vi "myRIO_BRig_RT_v0,78__PortC.vi"() -> ()   [LabVIEW 2014]
uses:
  myRIO_BRig_RT__Case_Exp_stateList.ctl
  myRIO_BRig_RT__Case_NonExp_stateList.ctl
  <vilib>/Platform/TimedLoop/XDataNode/timing_clust.ctl
  <vilib>/Platform/TimedLoop/XDataNode/nitl_modes.ctl
  <vilib>/Platform/TimedLoop/XDataNode/wakeup.ctl
  <vilib>/WebDAVClient/Advanced/SessionHandle.ctl
  <vilib>/myRIO/Common/Instrument Driver Framework/myRIO v1.0/UART/vis/myRIO v1.0 Close UART.vi
  <vilib>/FPGAPlugInAG/myRIO-1900/niLvFpga_Open_myRIO-1900.vi
  <vilib>/rvi/interface/common/dynamic/niFpgaDynamicAddResources.vi
  <vilib>/Utility/error.llb/Error Cluster From Error Code.vi
  <vilib>/rvi/errors/niLvFpgaAdjustHostInterfaceError.vi
  <vilib>/FPGAPlugInAG/Dynamic/niLvFpga_Close_Dynamic.vi
  <vilib>/myRIO/Common/Instrument Driver Framework/Utilities/vis/FPGA Ref Manager.vi
  <vilib>/myRIO/Common/Instrument Driver Framework/myRIO v1.0/myRIO v1.0 Reset FPGA.vi
  <vilib>/myRIO/Common/Instrument Driver Framework/myRIO v1.0/IRQ/vis/myRIO v1.0 IRQ Info FGV.vi
  <vilib>/myRIO/Common/Instrument Driver Framework/myRIO v1.0/IRQ/vis/myRIO v1.0 Timer IRQ Info FGV.vi
  <vilib>/myRIO/Common/Instrument Driver Framework/myRIO v1.0/IRQ/vis/myRIO v1.0 ISR Agent.vi
  <vilib>/rvi/interface/nirviOpenFPGA/nirviOpenFPGA.xnode
  FPGA Bitfiles/myRIOBRig_FPGATarget_myRIOBRigFPGAv3,_Jim92IOu6W4.lvbitx
  myRIO_BRig_FPGA_v3,70__PortC.vi
  <vilib>/rvi/interface/nirviReadWriteControl/nirviReadWriteControl.xnode
  <vilib>/Platform/TimedLoop/XDataNode/XDataNode.xnode
  <vilib>/rvi/interface/nirviCloseFPGA/nirviCloseFPGA.xnode
  <vilib>/Platform/TimedLoop/XDataNode/XDNodeRunTimeDep.lvlib
  <vilib>/rvi/interface/Simulation/niFpgaSimulationCallBeginRW.vi
  <vilib>/myRIO/Instrument Drivers/Utilities/Utilities.lvlib
  <vilib>/WebDAVClient/NI_WebDAV.lvlib
  NiFpgaLv.dll
panel:
  out "error out 6":errorcluster
  in  "MTrig_Laser_Switch":bool
  in  "Cue1Param_AudioLed_Count_NS":u16
  in  "Cue1Param_AudioLed_Count_Switch":u16
  in  "Cue1Param_AudioLed_Probability_NS":u16
  in  "Cue1Param_CueType_NS":u16(slide) max=2 step=1 scale=0.0..2.0
  in  "Cue1Param_AudioLed_Probability_Switch":u16
  in  "Cue1Param_CueType_Switch":u16(slide) max=2 step=1 scale=0.0..2.0
  in  "CueLed_Freq":dbl=10.0
  in  "CueLed_Tpeak":dbl=2.0
  in  "CueLed_duration":u16
  in  "Laser_power_step_l2":dbl
  in  "Laser_power_max_l2":dbl
  in  "Laser_power_min_l2":dbl
  in  "Laser_Tshutter_l2":dbl=2.0
  in  "Laser_Freq_l2":dbl=10.0
  in  "Laser_Tpeak_l2":dbl=2.0
  in  "Laser_duration_l2":u16
  in  "LC_Sel_Count_NS_l2":u16
  in  "LC_Sel_Count_Switch_l2":u16
  in  "LC_Sel_Probability_NS_l2":u16
  in  "LC_Sel_Block_NS_l2":u16(slide) max=2 step=1 scale=0.0..2.0
  in  "LC_Sel_OnOff_NS_l2":bool
  in  "LC_Sel_Probability_Switch_l2":u16
  in  "LC_Sel_Block_Switch_l2":u16(slide) max=2 step=1 scale=0.0..2.0
  in  "LC_Sel_OnOff_Switch_l2":bool
  in  "LC_Sel_Tdelay_NS_l2":u16
  in  "LC_Sel_Tdelay_Switch_l2":u16
  in  "LC_Cue1_Count_NS_l2":u16
  in  "LC_Cue1_Count_Switch_l2":u16
  in  "LC_Cue1_delayOpt_NS_l2":bool
  in  "LC_ENL1_delayOpt_NS_l2":bool
  in  "LC_ENL1_Count_NS_l2":u16
  in  "LC_ENL1_Count_Switch_l2":u16
  in  "LC_Cue1_delayOpt_Switch_l2":bool
  in  "LC_ENL1_delayOpt_Switch_l2":bool
  in  "LC_Cue1_Probability_NS_l2":u16
  in  "LC_Cue1_Block_NS_l2":u16(slide) max=2 step=1 scale=0.0..2.0
  in  "LC_Cue1_OnOff_NS_l2":bool
  in  "LC_Cue1_Probability_Switch_l2":u16
  in  "LC_Cue1_Block_Switch_l2":u16(slide) max=2 step=1 scale=0.0..2.0
  in  "LC_Cue1_OnOff_Switch_l2":bool
  in  "LC_ENL1_Probability_NS_l2":u16 max=100 step=1
  in  "LC_ENL1_Block_NS_l2":u16(slide) max=2 step=1 scale=0.0..2.0
  in  "LC_ENL1_OnOff_NS_l2":bool
  in  "LC_ENL1_Probability_Switch_l2":u16 max=100 step=1
  in  "LC_ENL1_Block_Switch_l2":u16(slide) max=2 step=1 scale=0.0..2.0
  in  "LC_Cue1_Tdelay_NS_l2":u16
  in  "LC_ENL1_Tdelay_NS_l2":u16
  in  "LC_Cue1_Tdelay_Switch_l2":u16
  in  "LC_ENL1_Tdelay_Switch_l2":u16
  in  "LC_ENL1_OnOff_Switch_l2":bool
  in  "LC_Wrong_Probability_l2":u16
  in  "LC_Wrong_Trial_l2":u16(slide) max=2 step=1 scale=0.0..2.0
  in  "LC_Wrong_Block_l2":u16(slide) max=2 step=1 scale=0.0..2.0
  in  "LC_Wrong_OnOff_l2":bool
  in  "LC_Reward_Probability_l2":u16
  in  "LC_Reward_Trial_l2":u16(slide) max=2 step=1 scale=0.0..2.0
  in  "LC_Reward_Block_l2":u16(slide) max=2 step=1 scale=0.0..2.0
  in  "LC_Reward_OnOff_l2":bool
  in  "LC_Wrong_Tdelay_l2":u16
  in  "LC_Reward_Tdelay_l2":u16
  in  "LC_Sel_Count_NS_l1":u16
  in  "LC_Sel_Count_Switch_l1":u16
  in  "LC_Sel_Probability_NS_l1":u16
  in  "LC_Sel_Block_NS_l1":u16(slide) max=2 step=1 scale=0.0..2.0
  in  "LC_Sel_OnOff_NS_l1":bool
  in  "LC_Sel_Probability_Switch_l1":u16
  in  "LC_Sel_Block_Switch_l1":u16(slide) max=2 step=1 scale=0.0..2.0
  in  "LC_Sel_OnOff_Switch_l1":bool
  in  "LC_Sel_Tdelay_NS_l1":u16
  in  "LC_Sel_Tdelay_Switch_l1":u16
  out "I_connect_TCP":bool
  out "error out 5":errorcluster
  in  "get_countPerMS":bool
  in  "count_warmup_R_reset":bool
  in  "count_warmup_L_reset":bool
  out "count_warmup_R":u16
  out "count_warmup_L":u16
  out "SolenoidReward":bool
  in  "SolenoidProbability_L":u16=50 caption="Reward Time [ms]" min=1 max=1000 step=1
  in  "SolenoidProbability_R":u16=50 caption="Reward Time [ms]" min=1 max=1000 step=1
  out "output_PortA":dbl caption="LaserPower"
  out "error out 4":errorcluster
  in  "Laser_power_step_l1":dbl
  in  "Laser_power_max_l1":dbl
  in  "Recording":bool
  out "error out 3":errorcluster
  out "error out 2":errorcluster
  in  "Laser_power_min_l1":dbl
  in  "FPGA_count2ms":dbl=159.0
  in  "Laser_Tshutter_l1":dbl=2.0
  in  "Laser_Freq_l1":dbl=10.0
  in  "Laser_Tpeak_l1":dbl=2.0
  in  "Laser_duration_l1":u16
  out "error out":errorcluster
  in  "LC_Cue1_Count_NS_l1":u16
  in  "LC_Cue1_Count_Switch_l1":u16
  in  "LC_Cue1_delayOpt_NS_l1":bool
  in  "LC_ENL1_delayOpt_NS_l1":bool
  in  "LC_ENL1_Count_NS_l1":u16
  in  "LC_ENL1_Count_Switch_l1":u16
  in  "LC_Cue1_delayOpt_Switch_l1":bool
  in  "LC_ENL1_delayOpt_Switch_l1":bool
  in  "Tcycle_Cue_max":u16=1000 caption="Max" min=5 max=5000 step=5
  in  "Tcycle_Cue_min":u16=1000 caption="Min" min=5 max=5000 step=5
  in  "SendData":bool
  out "cSpout":enum16{"Left", "Right"}(ring) caption="Left or Right Spout"
  out "A4":u32 caption="LickCounter_Right"
  out "A2":u32 caption="LickCounter_Left"
  in  "LR_wrong_Event":bool
  out "error_initTrial":errorcluster
  out "error_Selection_pre":errorcluster
  out "error_Selection":errorcluster
  out "SelectWrong":bool
  out "SelectReward":bool
  in  "Left(F)_or_Right(T)":bool
  in  "ignoreWrong":bool
  in  "SelectionState":bool
  in  "LR_wrong_Laser":bool
  in  "LR_reward_Laser":bool
  in  "LR_reward_Event":bool
  out "nRewards_Right":u16 caption="# Rewards Total (Right)"
  out "nRewards_Left":u16 caption="# Rewards Total (Left)"
  out "nRewards_cur":u16 caption="# Rewards in Current Block"
  out "TpB_target":u16 caption="Target Trials Per Block"
  out "cState_NonExp":T1 caption="WarmUp State"
  out "iBlock":u16 caption="Current Block"
  out "cState":T2 caption="Experimental State"
  out "iTrial":u16 caption="Current Trial"
  in  "warmupType":u8(slide) max=2 step=1 scale=0.0..2.0
  in  "TestConnection":bool
  in  "warmup":bool caption="WarmUp"
  in  "Data Set Prefix":string="Exp1_TM2"
  out "Connected To Host?":bool
  in  "Host Password":string="sabalab"
  in  "Host UserName":string="Test2"
  in  "sp_RightSpout":u16(slide)=2 max=2 step=1 scale=0.0..2.0
  in  "sp_LeftSpout":u16(slide)=2 max=2 step=1 scale=0.0..2.0
  in  "BUR_max":u16 caption="Count Reward Structure  (0 = off)"
  in  "LC_Wrong_Probability_l1":u16
  in  "LC_Wrong_Trial_l1":u16(slide) max=2 step=1 scale=0.0..2.0
  in  "LC_Wrong_Block_l1":u16(slide) max=2 step=1 scale=0.0..2.0
  in  "LC_Wrong_OnOff_l1":bool
  in  "LC_Reward_Probability_l1":u16
  in  "LC_Reward_Trial_l1":u16(slide) max=2 step=1 scale=0.0..2.0
  in  "LC_Reward_Block_l1":u16(slide) max=2 step=1 scale=0.0..2.0
  in  "LC_Reward_OnOff_l1":bool
  in  "LC_Cue1_Probability_NS_l1":u16
  in  "LC_Cue1_Block_NS_l1":u16(slide) max=2 step=1 scale=0.0..2.0
  in  "LC_Cue1_OnOff_NS_l1":bool
  in  "LC_Cue1_Probability_Switch_l1":u16
  in  "LC_Cue1_Block_Switch_l1":u16(slide) max=2 step=1 scale=0.0..2.0
  in  "LC_Cue1_OnOff_Switch_l1":bool
  in  "LC_ENL1_Probability_NS_l1":u16 max=100 step=1
  in  "LC_ENL1_Block_NS_l1":u16(slide) max=2 step=1 scale=0.0..2.0
  in  "LC_ENL1_OnOff_NS_l1":bool
  in  "LC_ENL1_Probability_Switch_l1":u16 max=100 step=1
  in  "LC_ENL1_Block_Switch_l1":u16(slide) max=2 step=1 scale=0.0..2.0
  in  "Tcycle_Timeout":u16=1000 caption="Timeout Time [ms]" min=10 max=10000 step=1
  in  "Tcycle_Wrong":u16=1000 caption="Wrong Time [ms]" min=10 max=10000 step=1
  in  "Tcycle_Selection":u16=1000 caption="Answer Time [ms]" min=1 max=10000 step=1
  in  "Tcycle_RewardPost":u16=1000 caption="Consumption Time [ms]" min=250 max=10000 step=250
  in  "Tcycle_Reward_L":u16=500 caption="Reward Time [ms]" min=1 max=1000 step=1
  in  "Tcycle_Reward_R":u16=500 caption="Reward Time [ms]" min=1 max=1000 step=1
  in  "TpB_Max_R":u16=4 caption="Max TrialsPerBlock" min=1 max=12 step=1
  in  "TpB_Min_R":u16=4 caption="Min TrialsPerBlock" min=1 max=12 step=1
  in  "TpB_Max_L":u16=4 caption="Max TrialsPerBlock" min=1 max=12 step=1
  in  "TpB_Min_L":u16=4 caption="Min TrialsPerBlock" min=1 max=12 step=1
  in  "BUR_min":u16 caption="Count Reward Structure\n(0 = off)"
  in  "TrialUntilReward":bool caption="Ignore Wrong Selection"
  in  "CueCycles":u16=1 caption="Cue Structure" min=1 max=1 step=1
  in  "MTrig_Laser_Tcycle":u16=10 caption="Time [ms]"
  in  "MTrig_Laser_trig":bool
  in  "MTrig_Audio_trig__R":bool caption="Trigger Audio"
  in  "MTrig_Audio_trig__L":bool caption="Trigger Audio"
  in  "RewCalib_Trig_R":bool caption="Calibrate_R"
  in  "RewCalib_Trig_L":bool caption="Calibrate_L"
  in  "MTrig_Solenoid_Tcycle__R":u16=300 caption="Time [ms]"
  in  "MTrig_Solenoid_Tcycle__L":u16=300 caption="Time [ms]"
  in  "MTrig_Solenoid_trig__R":bool caption="Solenoid"
  in  "MTrig_Solenoid_trig__L":bool caption="Solenoid"
  in  "STOP_abort":bool caption="Stop LabView\n(Stops myRio and FPGA)"
  in  "STOP_endBlock":bool caption="Stop Experiment\n@ End of Block"
  in  "STOP_endTrial":bool caption="Stop Experiment\n@ End of Trial"
  in  "START":bool caption="Start Experiment"
  in  "Tcycle_CuePenalty":u16=1000 caption="Penalty" min=1 max=10000 step=1
  in  "Audio_Amp__R":u16=100 caption="Amp"
  in  "Audio_Freq__R":u8=5 caption="Freq [kHz]" max=14 step=1
  in  "Audio_Amp__L":u16=100 caption="Amp"
  in  "Audio_Freq__L":u8=5 caption="Freq [kHz]" max=14 step=1
  in  "LC_Wrong_Tdelay_l1":u16
  in  "LC_Cue1_Tdelay_NS_l1":u16
  in  "LC_ENL1_Tdelay_NS_l1":u16
  in  "LC_Reward_Tdelay_l1":u16
  in  "LC_Cue1_Tdelay_Switch_l1":u16
  in  "LC_ENL1_Tdelay_Switch_l1":u16
  in  "LC_ENL1_OnOff_Switch_l1":bool
  in  "Tcycle_ENLPenalty":u16=100 caption="Penalty" min=10 max=10000 step=10
  in  "Tcycle_ENL_max":u16=1000 caption="Max" min=250 max=10000 step=250
  in  "Tcycle_ENL_min":u16=1000 caption="Min" min=250 max=10000 step=250
  # "Communication (Host PC)"
  # "Recording Rig"
  # "Experimental Run"
  # "Current State"
  # "STOP experiment at"
  # "Global Parameters                                                         Trial Parameters"
  # "Left/Right        Give Reward?        Laser Power [V]"
  # "FPGA Count per [ms]"
  # "Experiment Task Structure"
  # "Timing [ms]"
  # "Block                   Trial            Target Trials       # Rewards \n                                                            Per Block             Current"
  # "Min            Max            Penalty"
  # "(1) = Switching\n(2) = Two Choice"
  # "WarmUp State"
  # "Lick Counter"
  # "Enforced\nNonLick"
  # "WarmUp"
  # "Left           Right"
  # "Cue then reward (no lick)\n \nLeft                    Right"
  # "# Rewards Total\n                                                                  Left                    Right"
  # "Cue"
  # "Experimental State"
  # "Selection\n \n\n \nReward\n    Dispense\n    Time\n \n    Dispense\n    Probability\n \n\n    Consumption\n    Time\n\nWrong Choice\n \n \nTimeout Penalty"
  # "Laser1 Control\n                               On/Off      Block        Probability [%]   Delay [ms]                              Count"
  # "Left                  Right"
  # "Manual Control"
  # "Enforced\nNonLick\n      1"
  # "Min"
  # "Max"
  # "from end"
  # "Solenoid\n \nLeft              Right"
  # "Switch\nTrial"
  # "Speaker\n \nLeft                    Right"
  # "Laser 1  |  Laser 2"
  # "from start"
  # "Trial Per Block Structure \n               Left                        Right"
  # "from end"
  # "NonSwitch\nTrials"
  # "from start"
  # "Time\n[ms]"
  # "Time\n[ms]"
  # "Time = Cue Min"
  # "Min"
  # "Cue 1"
  # "Power = Min"
  # "from end"
  # "Switch\nTrial"
  # "Max"
  # "from start"
  # "Cue Audio Parameters"
  # "Laser1 Parameters"
  # "Left                  Right"
  # "from end"
  # "Laser1 Response\n                               On/Off      Block       Trial       Probability [%]   Delay [ms]"
  # "Frequency\n[Hz]"
  # "NonSwitch\nTrials"
  # "Frequency\n[kHz]"
  # "from start"
  # "Timing [ms]\n Duration     Peak Width   Shutter"
  # "Selection Reward"
  # "Selection"
  # "Amp\n(0 - 32,000)"
  # "from start"
  # "Switch\nTrial"
  # "Laser Power [V]\nMin          Max              Step"
  # "Speaker\nPattern\nDuring Cue"
  # "Selection Wrong"
  # "from start"
  # "NonSwitch\nTrials"
  # "Cue LED Parameters"
  # "Laser2 Parameters"
  # "Laser2 Response\n                               On/Off      Block       Trial       Probability [%]   Delay [ms]"
  # "Laser2 Control\n                               On/Off      Block        Probability [%]   Delay [ms]                              Count"
  # "Frequency\n[Hz]"
  # "Frequency\n[Hz]"
  # "Selection Reward"
  # "Enforced\nNonLick\n      1"
  # "from end"
  # "Timing [ms]\n Duration     Peak Width"
  # "Timing [ms]\n Duration     Peak Width   Shutter"
  # "Switch\nTrial"
  # "from start"
  # "Selection Wrong"
  # "from end"
  # "Laser Power [V]\nMin          Max              Step"
  # "NonSwitch\nTrials"
  # "from start"
  # "Cue 1"
  # "from end"
  # "Switch\nTrial"
  # "from start"
  # "Cue1 Control\n                                         Cue Type                     Audio or LED       LED Probability [%]      Count"
  # "from end"
  # "NonSwitch\nTrials"
  # "Cue 1"
  # "from start"
  # "Switch\nTrial"
  # "Selection"
  # "from start"
  # "Switch\nTrial"
  # "NonSwitch\nTrials"
  # "from start"
  # "NonSwitch\nTrials"
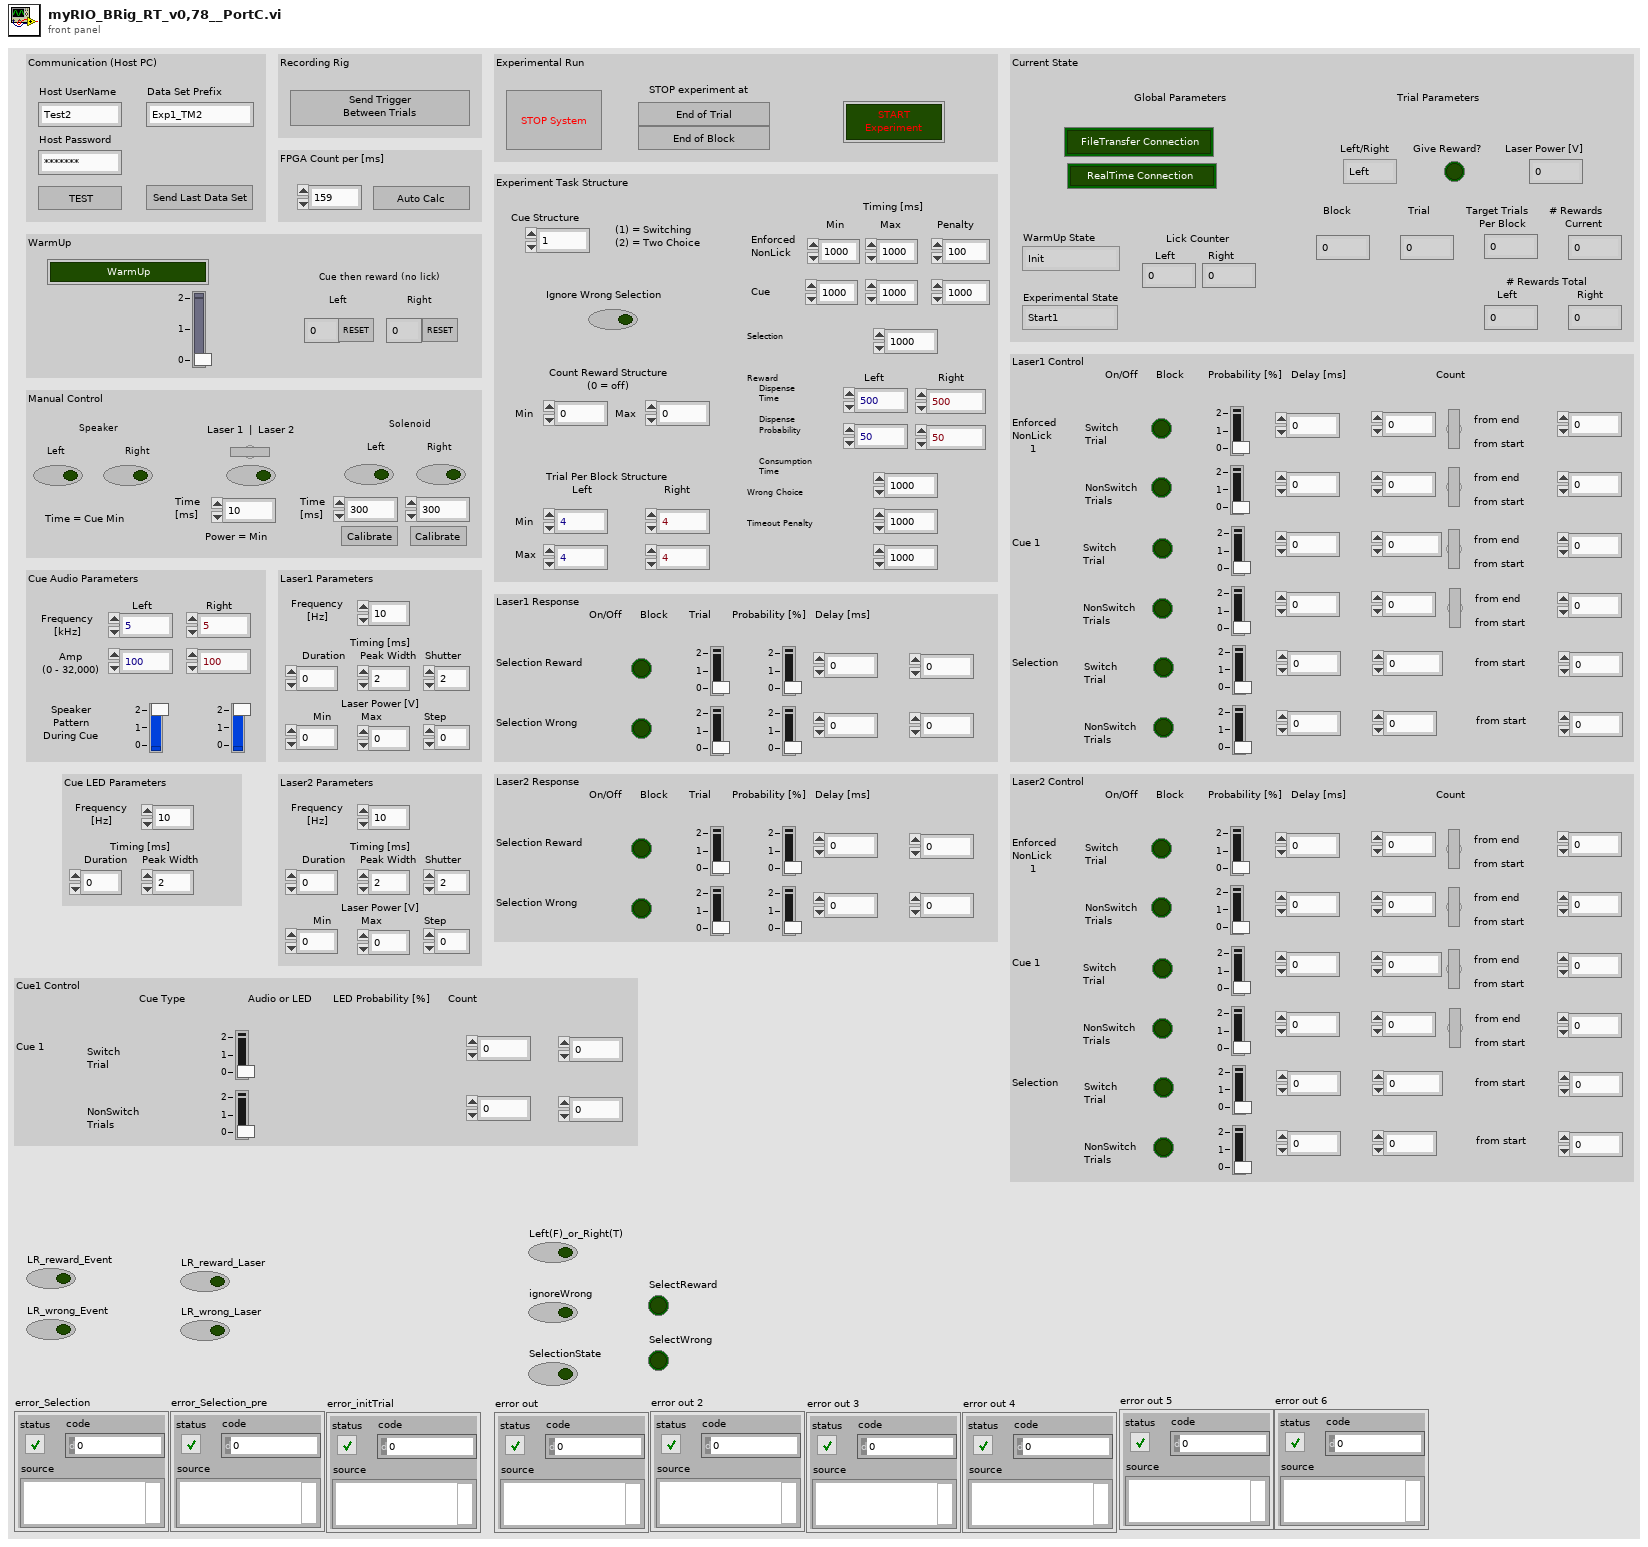
[diagram p1: front panel]
types:
  T1 = typedef "myRIO_BRig_RT__Case_NonExp_stateList.ctl" = enum16{"Init", "UploadSettings_pre", "UploadSettings_Read_dataExp", "UploadSettings_dataExp_1", "UploadSettings_dataExp_2", "UploadSettings_Read_dataLC", "UploadSettings_dataLC_1", "UploadSettings_dataLC_2", "UploadSettings_dataLC_3", "UploadSettings_dataLC_4", "UploadSettings_Read_dataMTrig", "UploadSettings_dataMTrig_1", "UploadSettings_post", "Idle_pre", "IdleEmpty", "IdleEmpty2", "IdleEmpty3", "IdleEmpty4", "Idle", "Idle_2", "Idle_3", "Idle_4", "Idle_5", "Idle_6", "Idle_post", "Cue_pre__pre", "Cue_pre", "Cue", "Cue_LED", "Cue_post", "RewardCalibration_pre", "DispenseWater_pre__pre", "DispenseWater_pre", "DispenseWater", "DispenseWater_post", "TestConnection", "SendData", "Get_FPGA_count_per_ms", "End"}
  T2 = typedef "myRIO_BRig_RT__Case_Exp_stateList.ctl" = enum16{"Start1", "Start2", "Start3", "saveSettings1", "saveSettings2", "saveSettings3", "saveSettings4", "saveSettings_LC_ENL_l1", "saveSettings_LC_ENL_l2", "saveSettings_LC_Cue_l1", "saveSettings_LC_Cue_l2", "saveSettings6_LC_l1_Other", "SaveSettings6_LC_l2_Other", "setSettings_Audio", "setSettings_Laser", "initBlock_pre", "initBlock", "initBlock2", "initBlock_post", "initTrial_pre", "initTrial", "initTrial2", "initTrial3", "initTrial4", "initTrial_LC_ENL1", "initTrial_LC_Cue1", "initTrial_LC_Cue1_2", "initTrial_LC_Sel", "initTrial_post", "ENL1_pre", "ENL1", "ENL1_post", "ENL1Penalty_pre", "ENL1Penalty", "ENL2_pre", "ENL2", "ENL2Penalty_pre", "ENL2Penalty", "Cue1_pre", "Cue1", "Cue1_post", "Cue1Penalty_pre", "Cue1Penalty", "Cue2_pre", "Cue2", "Cue2Penalty_pre", "Cue2Penalty", "Selection_pre", "Selection", "Select_post", "SelectReward_pre", "SelectReward", "SelectRewardPost_pre", "SelectRewardPost", "SelectWrong_pre", "SelectWrong", "SelectWrong_post", "SelectTimeout_pre", "SelectTimeout", "SelectTimeout_post", "endTrial_pre", "endTrial1", "endTrial2", "endTrial3", "endTrial_post", "endBlock_pre", "endBlock", "endBlock_post", "endExp", "commConnect", "commUpload_pre", "commUpload_dataBlock", "commUpload_dataCurrent", "commUpload_dataExp", "commUpload_dataLC", "commUpload_dataTrial", "commUpload_post", "saveData_pre", "saveData_dataBlock", "saveData_dataCurrent", "saveData_dataExp", "saveData_dataLC", "saveData_dataTrial", "saveData_post", "empty_endBlock1", "empty_endBlock2", "empty_endTrial1", "empty_endTrial2", "empty_endTrial3", "empty_endTrial4", "empty_endTrial5", "dummyState", "dummyState_endBlock"}
  T3 = typedef "XDNodeRunTimeDep.lvlib/timing_clust.ctl" = cluster{"Expected End [f-1]":u64, "Actual End [f-1]":u64, "Finished Late? [f-1]":bool, "Expected End [i-1]":u64, "Actual End [i-1]":u64, "Finished Late? [i-1]":bool, "Expected Start [i]":u64, "Actual Start [i]":u64, "Expected Start [f]":u64, "Actual Start [f]":u64, "Source Name":string, "Structure Name":string, "Period":i64, "Deadline":i64, "Offset":i64, "Start":i64, "Priority":i32, "Timeout":i32, "Mode":T4, "Wakeup Reason":T5, "Error":errorcluster, "Source Type":string, "Secondary Source Type":string, "Global End Time":u64, "Global Start Time":u64, "Frame Duration":u64, "Iteration Duration":u64, "Assigned CPU":i32, "I/O Scan Engine Mode":u32}
  T4 = typedef "XDNodeRunTimeDep.lvlib/nitl_modes.ctl" = enum32{"No Change", "Process missed periods, maintain original phase", "Discard missed periods, maintain original phase", "Process missed periods, ignore original phase", "Discard missed periods, ignore original phase"}
  T5 = typedef "XDNodeRunTimeDep.lvlib/wakeup.ctl" = enum32{"Normal", "Aborted", "Asynchronous wakeup", "Timing source error", "Timed loop error", "Timeout"}
  T6 = typedef "NI_WebDAV.lvlib/SessionHandle.ctl" = refnum<k1>
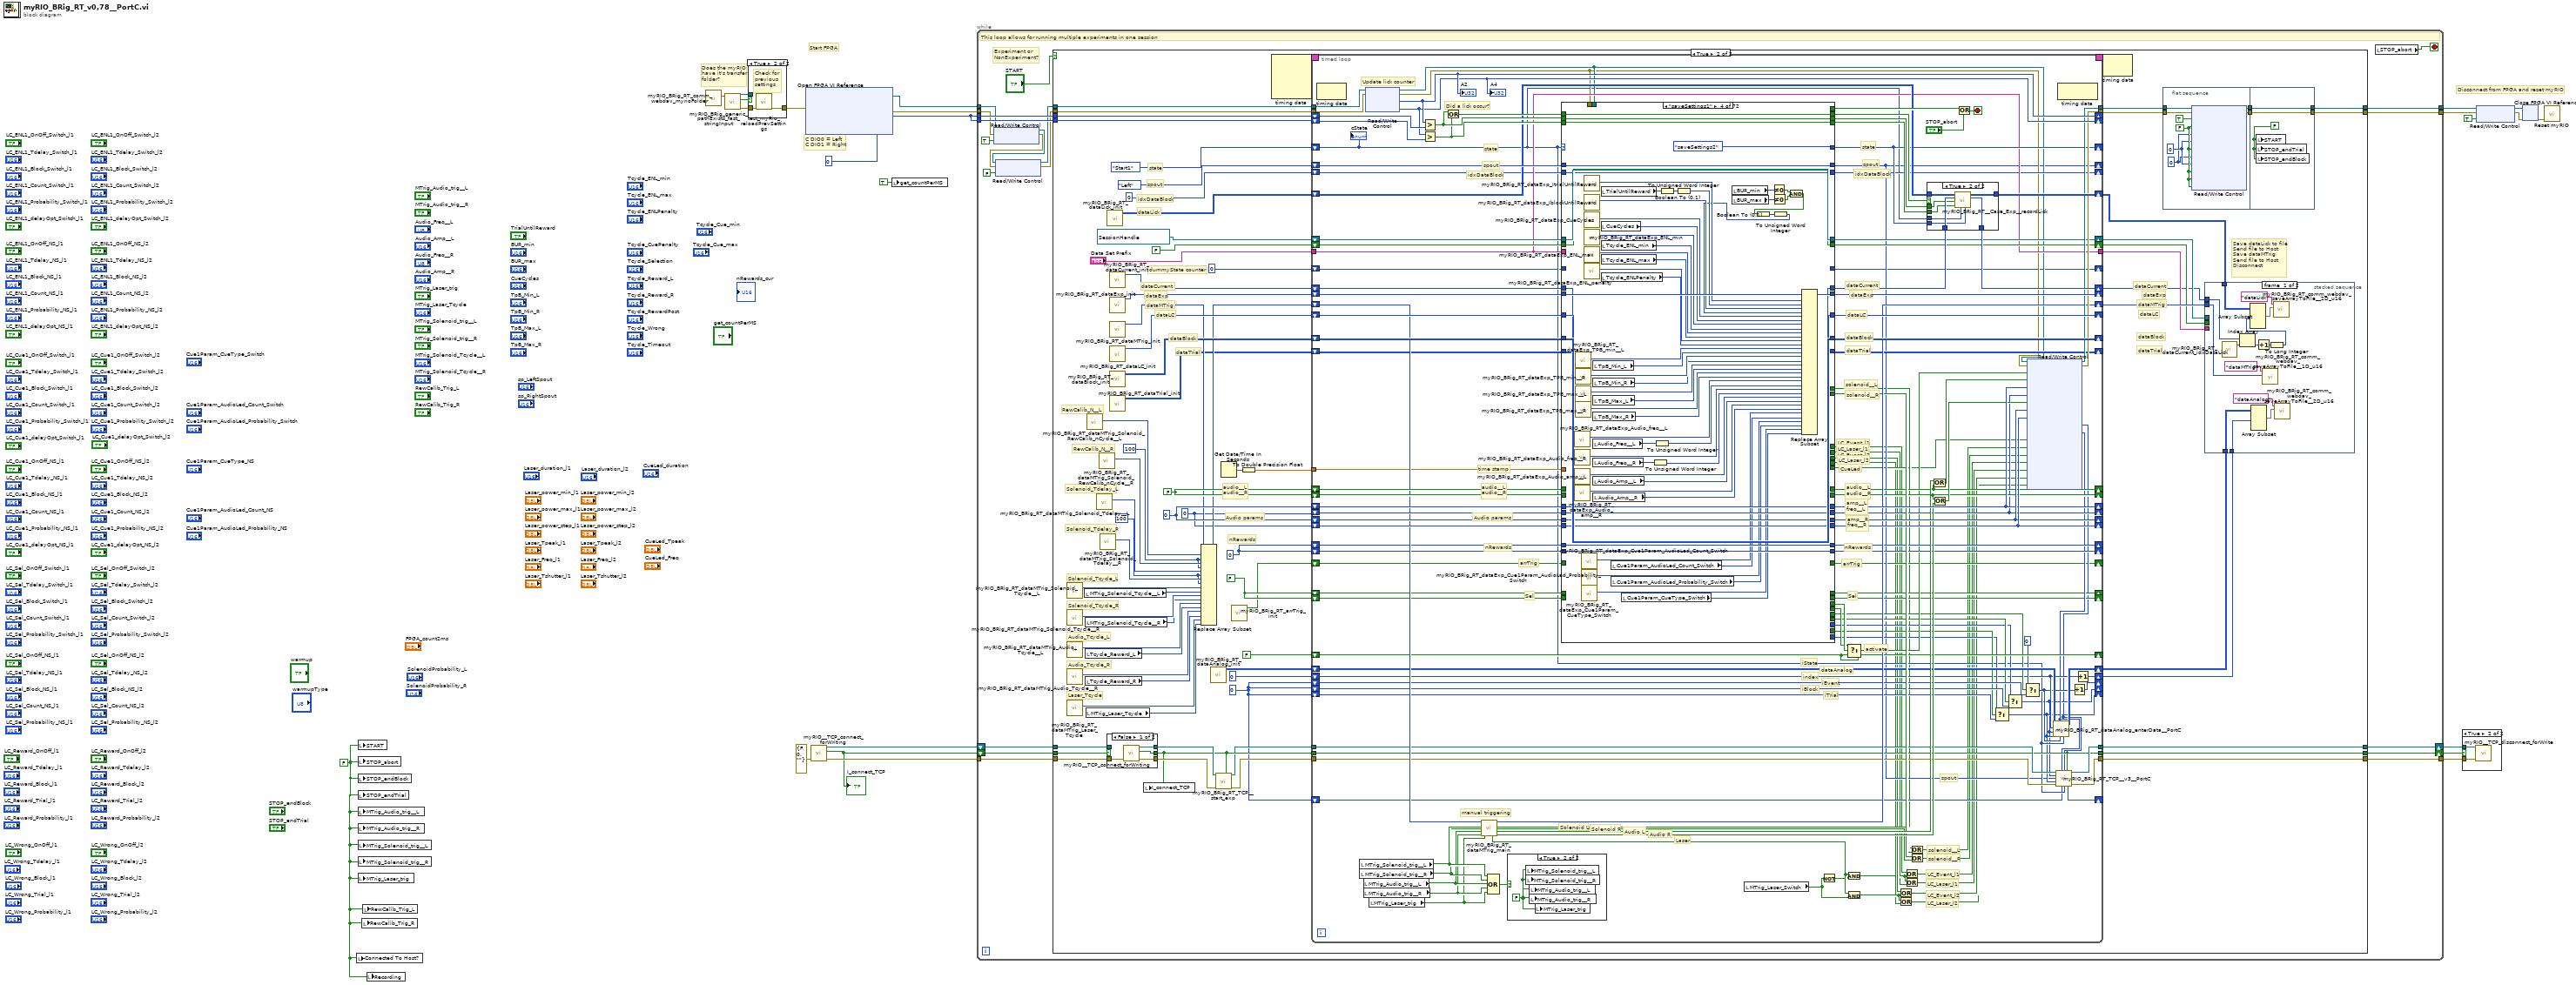
[diagram p0: block diagram]
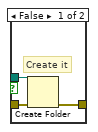
[diagram p3: hidden frame]
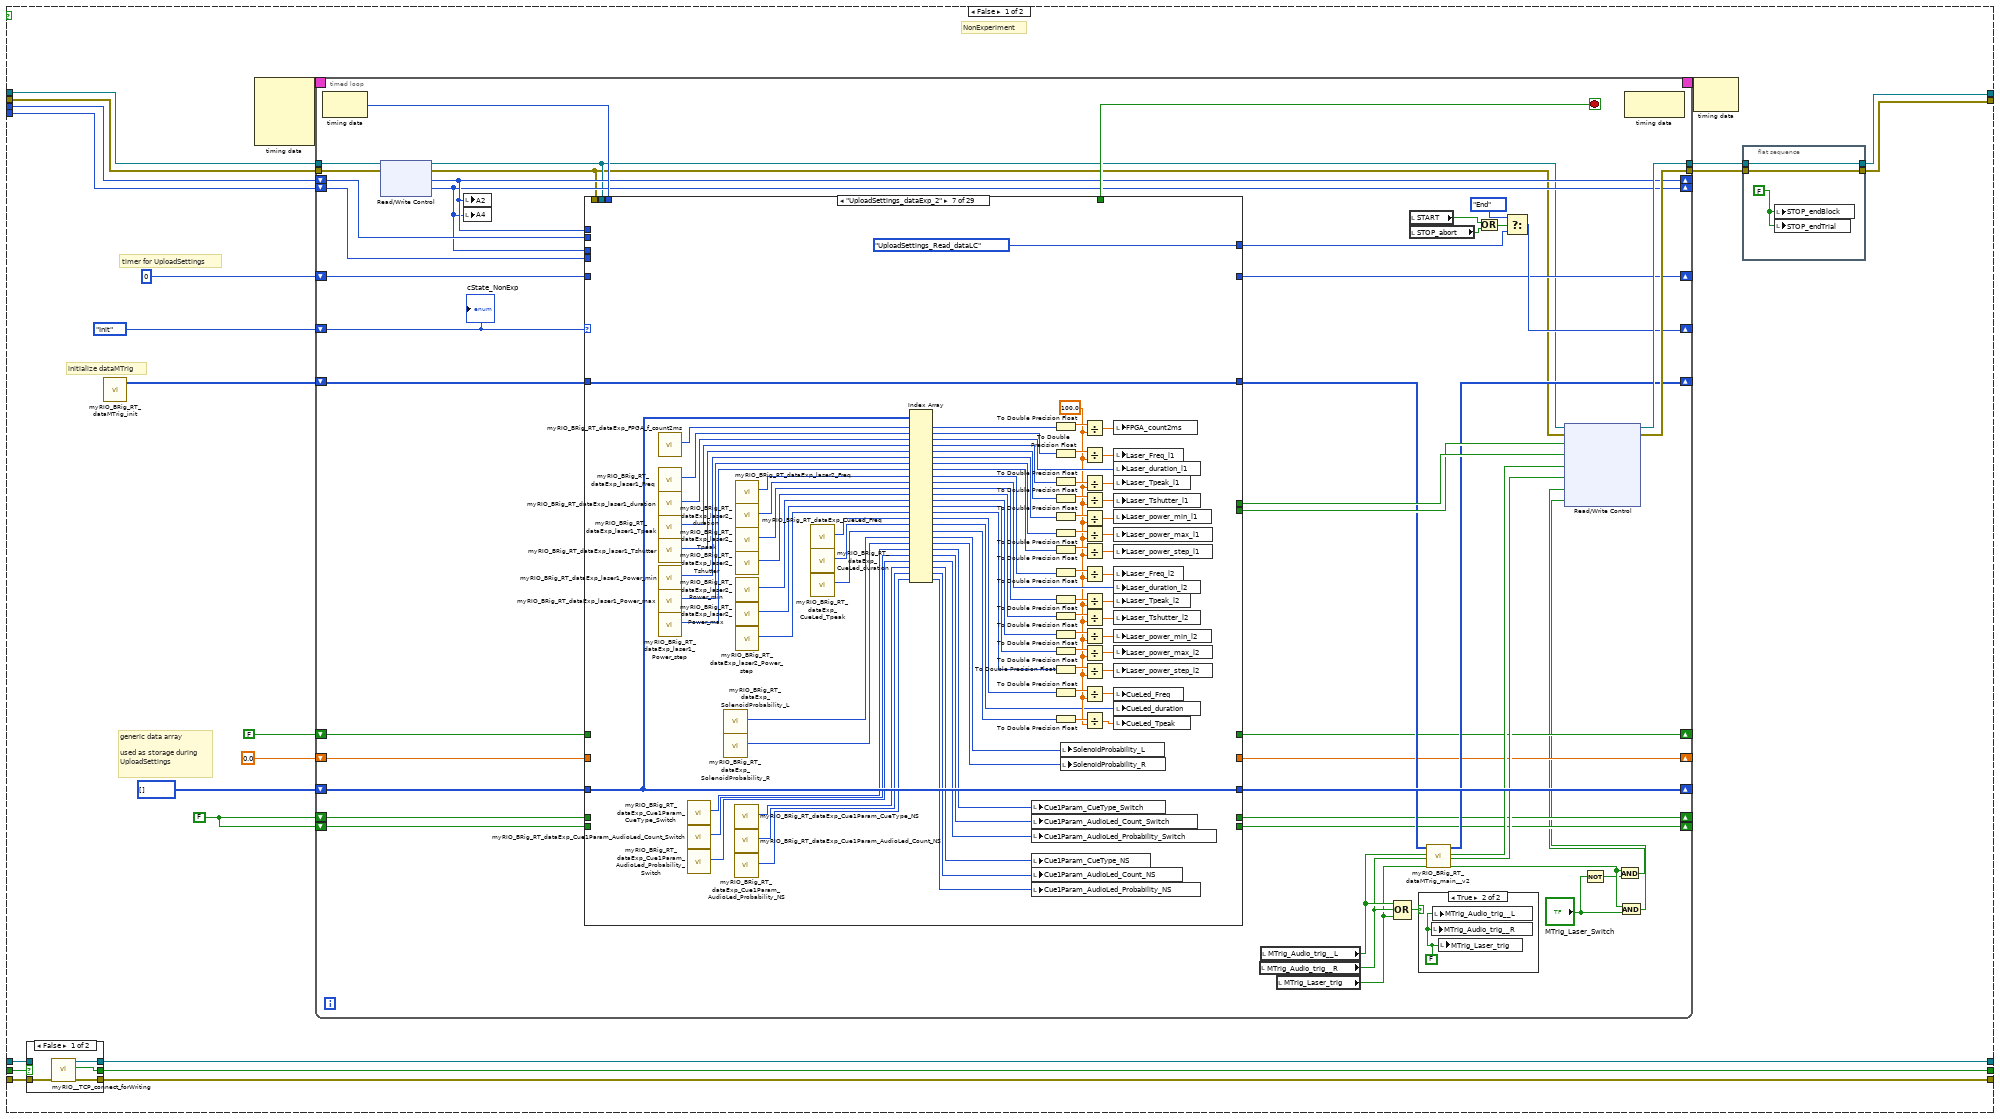
[diagram p4: hidden frame]
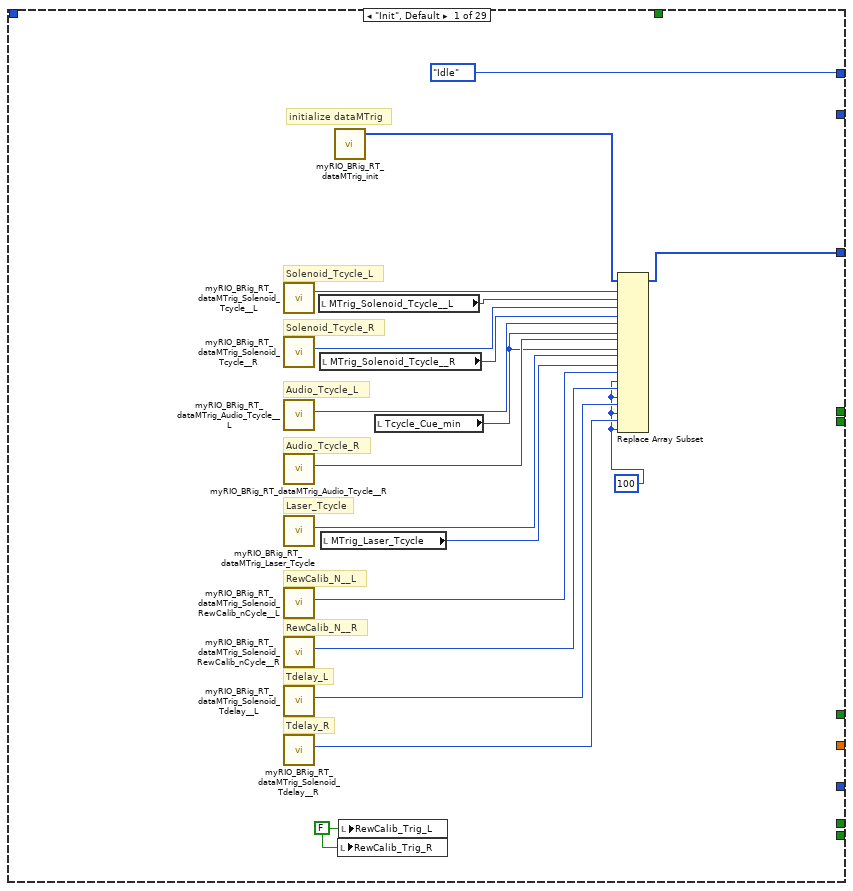
[diagram p7: hidden frame]
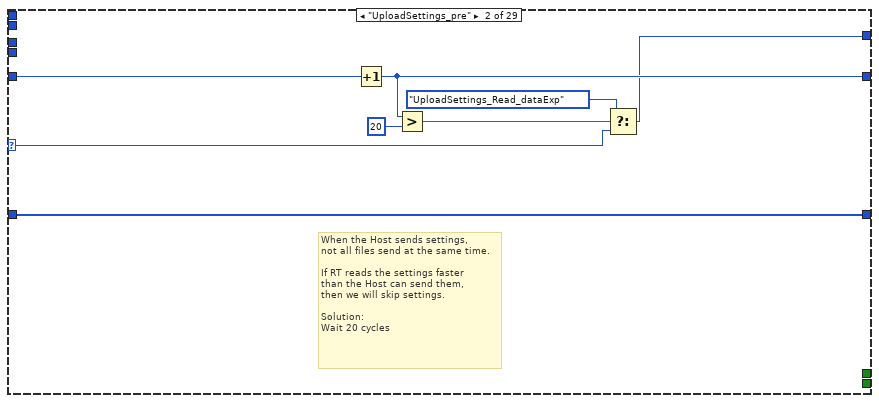
[diagram p8: hidden frame]
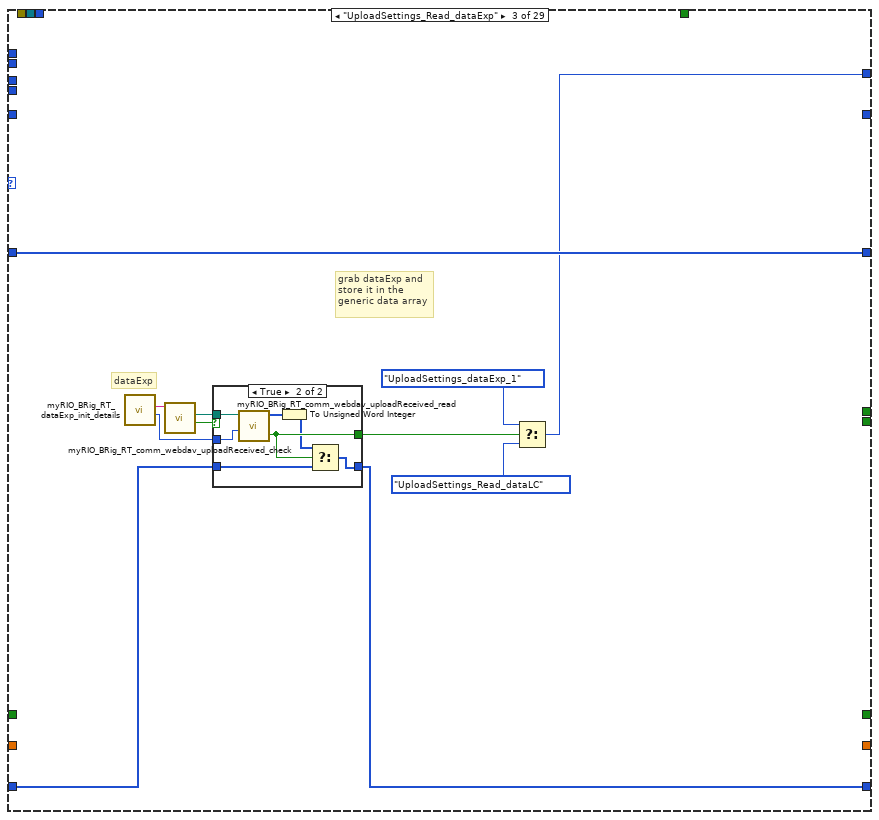
[diagram p9: hidden frame]
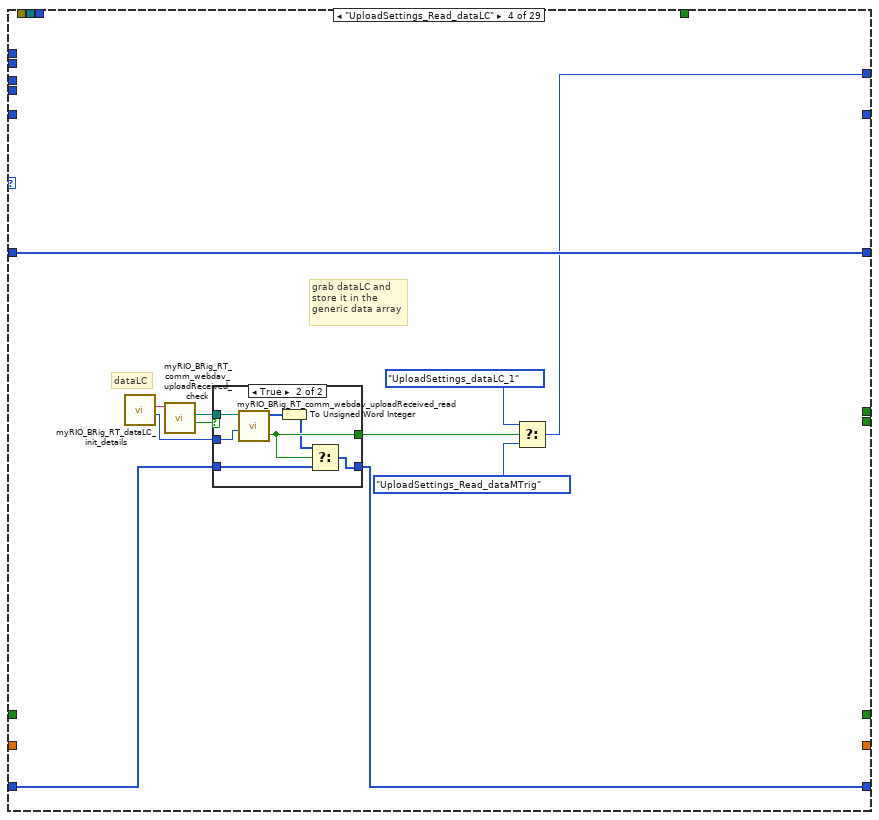
[diagram p11: hidden frame]
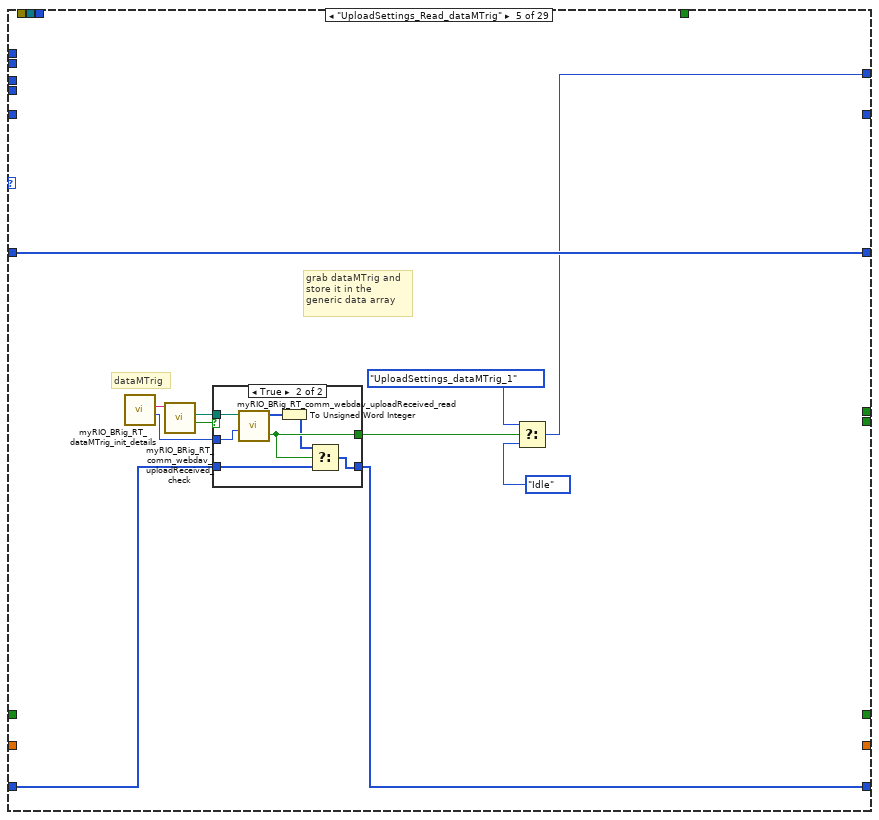
[diagram p13: hidden frame]
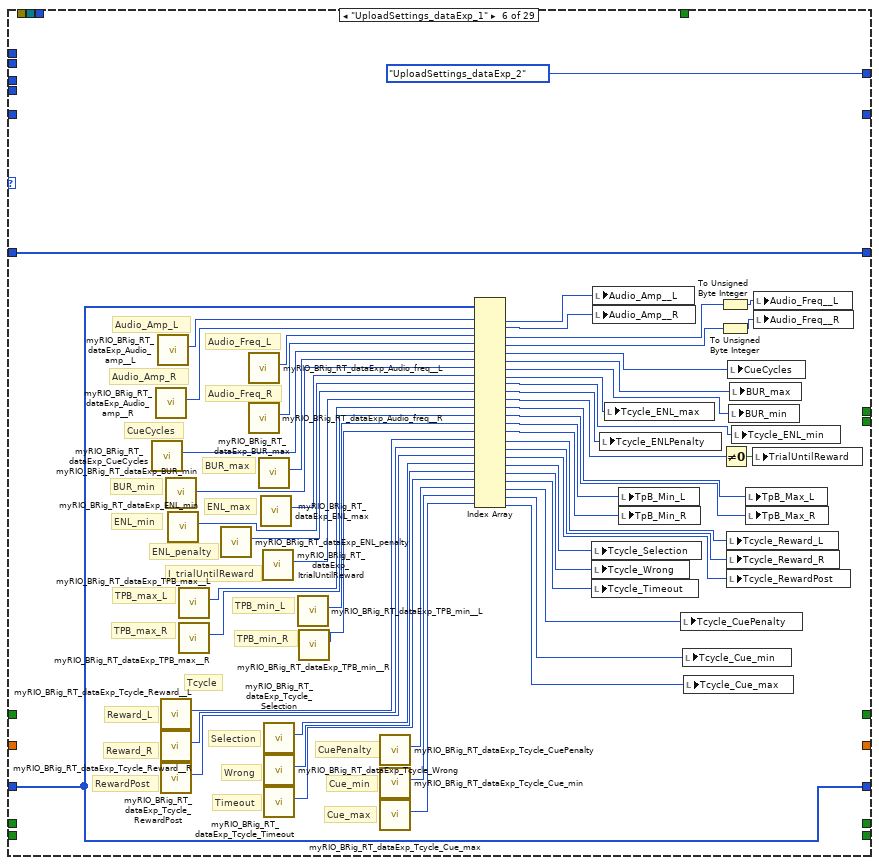
[diagram p15: hidden frame]
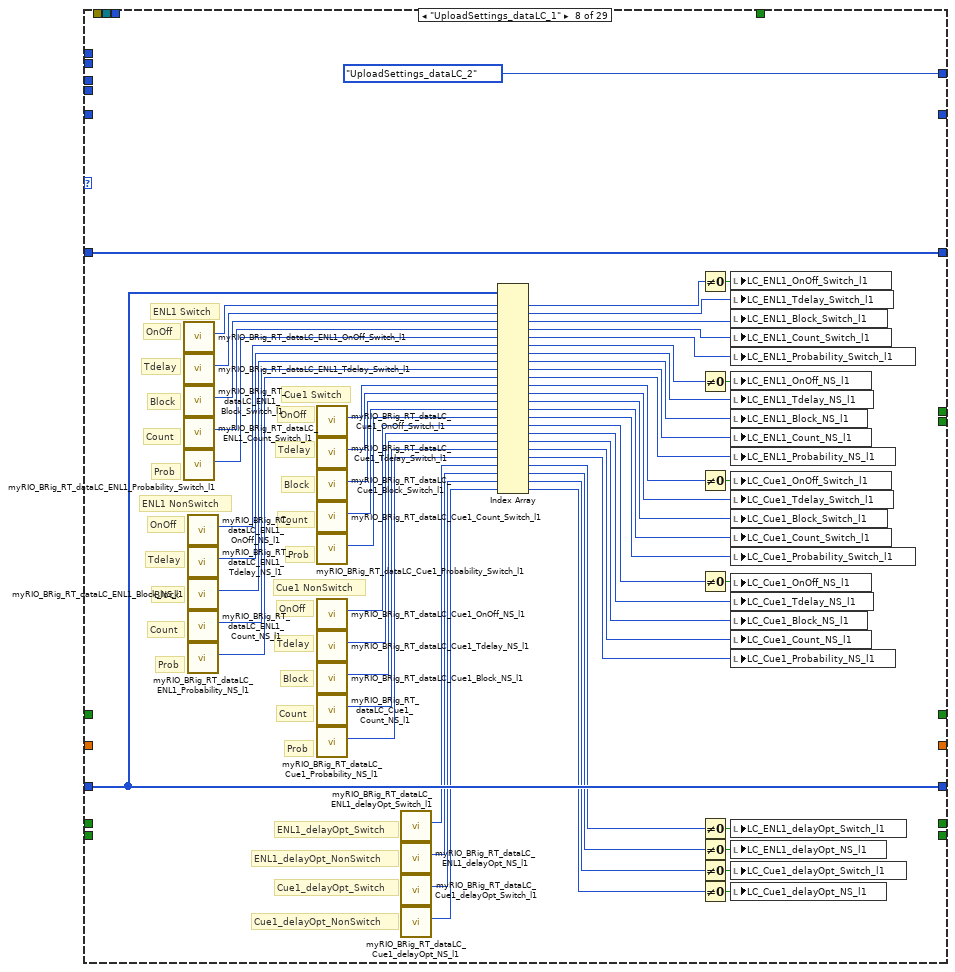
[diagram p16: hidden frame]
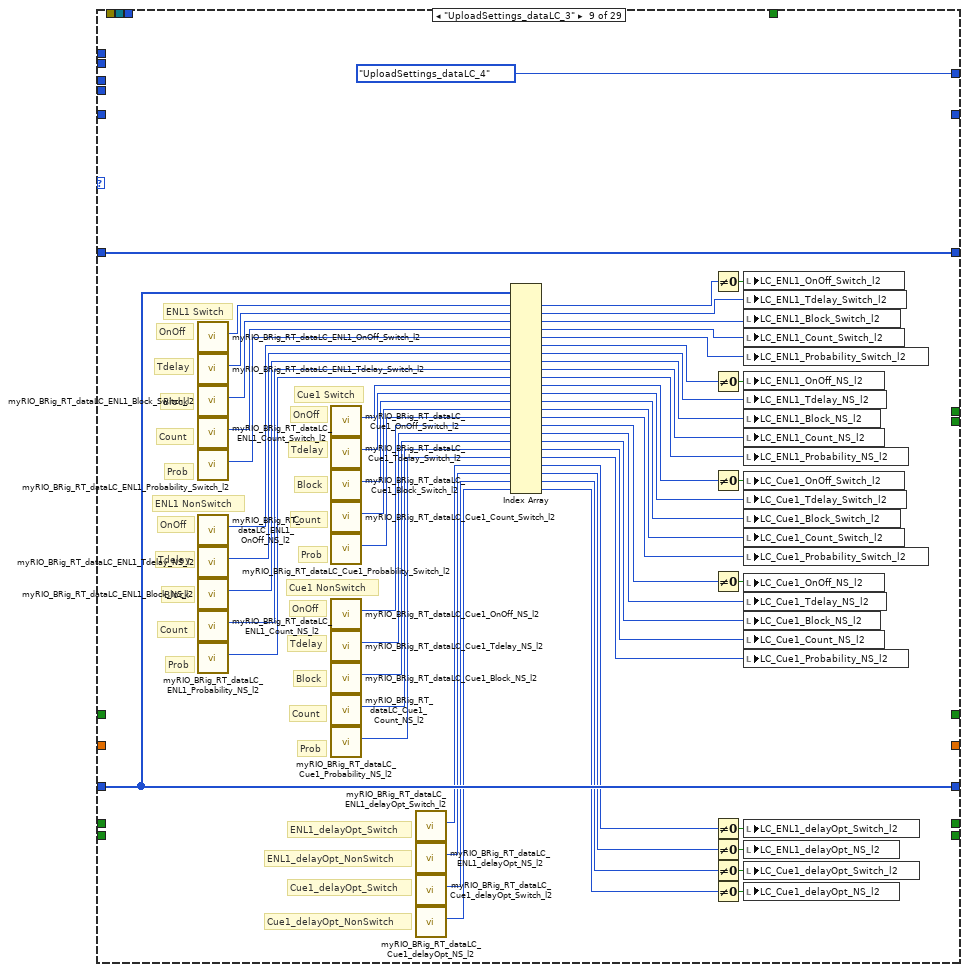
[diagram p17: hidden frame]
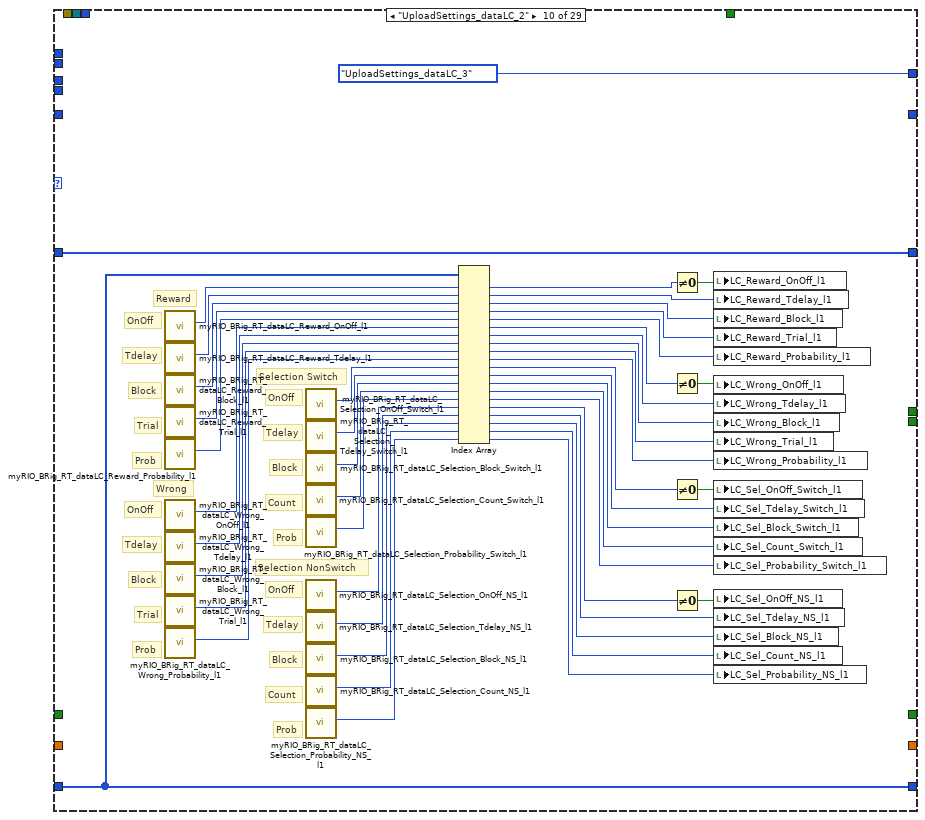
[diagram p18: hidden frame]
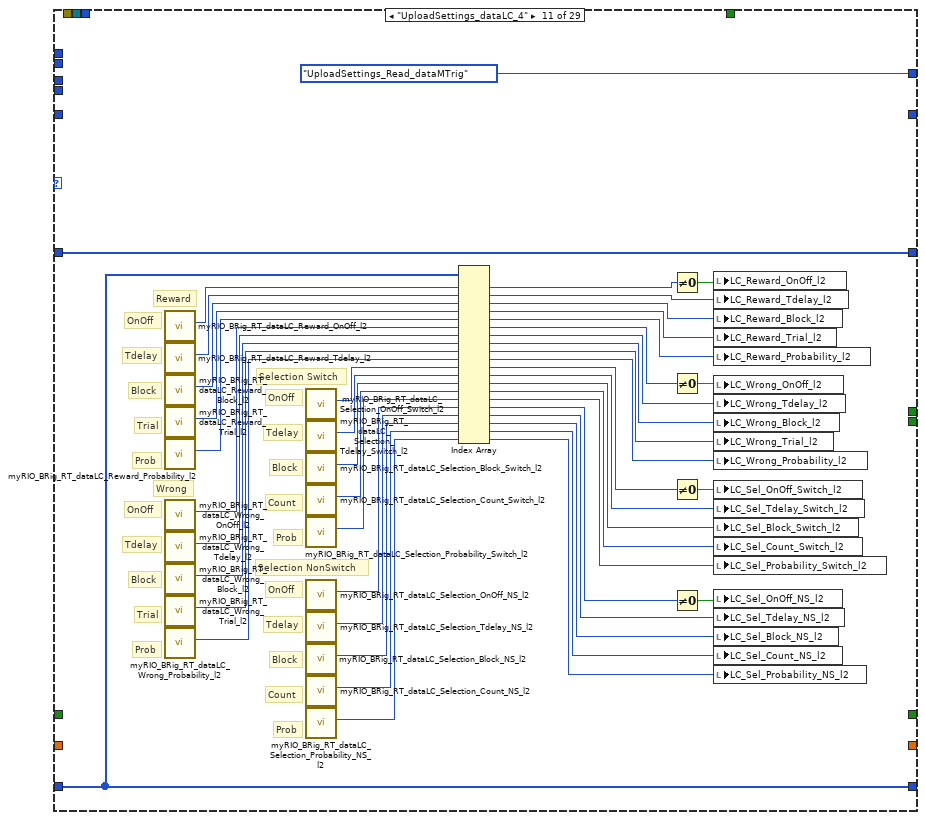
[diagram p19: hidden frame]
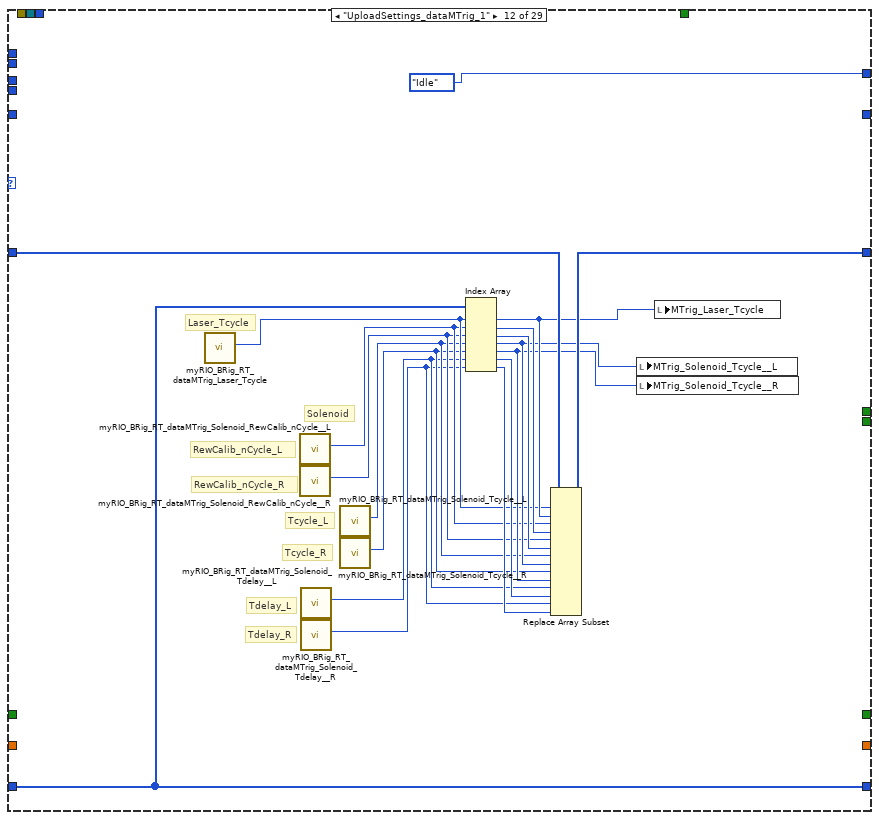
[diagram p20: hidden frame]
diagram:
  w17 = u32 0
  w1 = FALSE
  # "Does the myRIO\nhave it's transfer\nfolder?"
  # "C DIO0 = Left\nC DIO1 = Right"
  # "Start FPGA"
  # "Disconnect from FPGA and reset myRIO"
  n1 = local write "Connected To Host?"(w1) -> ()
  n2 = local write "START"(w1) -> ()
  n3 = local write "STOP_abort"(w1) -> ()
  n4 = local write "STOP_endBlock"(w1) -> ()
  n5 = local write "STOP_endTrial"(w1) -> ()
  n6 = local write "MTrig_Audio_trig__L"(w1) -> ()
  n7 = local write "MTrig_Audio_trig__R"(w1) -> ()
  n8 = local write "MTrig_Solenoid_trig__L"(w1) -> ()
  n9 = local write "MTrig_Solenoid_trig__R"(w1) -> ()
  n10 = local write "MTrig_Laser_trig"(w1) -> ()
  n11 = local write "RewCalib_Trig_R"(w1) -> ()
  n12 = local write "RewCalib_Trig_L"(w1) -> ()
  n13 = local write "Recording"(w1) -> ()
  n14 = call "myRIO_BRig_RT_comm_webdav_myrioFolder.vi"() -> ("output_myrioFolder"=w14:string)  [unwired: 11 in]
  n15 = call "myRIO_BRig_generic_pathExists_fast_stringInput.vi"("input_filePath"=w14) -> ("output_error"=w13:errorcluster, "output_Iexist"=w12:bool, "output_filePath"=w11:path)  [unwired: 8 in]
  n16 = case shown="True" w12 {
    tunnel: w11 -> [w26 _]
    tunnel: w13 -> [w25 w28]
    tunnel: [w24 w27] -> w9
    frame False {
      # "Create it"
      n17 = Create Folder(path (use dialog)=w26, error in=w25) -> (error out=w24:errorcluster)  [unwired: 1 in, 2 out]
    }
    frame True {
      # "Check for\nprevious\nsettings"
      n18 = call "test_myRio_reloadPrevSettings.vi"("input_error"=w28) -> ("output_error"=w27:errorcluster)  [unwired: 10 in]
    }
  }
  n19 = xnode "Open FPGA VI Reference"("error in"=w9) -> ("FPGA VI Reference Out"=w19:refnum<k20>, "error out"=w18:errorcluster)  [unwired: 1 in]
  n20 = call "myRIO__TCP_connect_forWriting.vi"("input_error"=errorcluster {"status"=FALSE, "code"=0, "source"=""}) -> ("output_error"=w7:errorcluster, "output_connected"=w6:bool, "output_hTCP"=w10:refnum<k5>)  [unwired: 8 in]
  "I_connect_TCP" <- w6
  n21 = local write "get_countPerMS"(TRUE ("get_countPerMS")) -> ()
  n22 = while {
    tunnel: w19 -> [w38]
    tunnel: w18 -> [w43]
    tunnel: w17 -> [w46]
    tunnel: w17 -> [w45]
    tunnel: [w36] -> w16
    tunnel: [w35] -> w15
    shift-right: [w32] -> w5
    shift-left: w6 -> [w33]
    tunnel: w7 -> [w31]
    shift-right: [w30] -> w4
    shift-left: w10 -> [w34]
    tunnel: [w29] -> w3
    stop <- w44 stop-if-true
    # "Experiment or\nNonExperiment?"
    # "This loop allows for running multiple experiments in one session"
    n23 = xnode "Read/Write Control"("FPGA VI Reference In"=w38, "error in"=w43, "Counts_Reset"=TRUE) -> ("FPGA VI Reference Out"=w40:refnum<k20>, "error out"=w41:errorcluster)
    n24 = xnode "Read/Write Control"("FPGA VI Reference In"=w40, "error in"=w41, "Counts_Reset"=FALSE) -> ("FPGA VI Reference Out"=w37:refnum<k20>, "error out"=w39:errorcluster)
    n25 = case shown="True" "START" {
      tunnel: w46 -> [w67 w1291]
      tunnel: w45 -> [w66 w1290]
      tunnel: w39 -> [w64 w1221]
      tunnel: w37 -> [w65 w1222]
      tunnel: [w62 w1287] -> w36
      tunnel: [w60 w1282] -> w35
      tunnel: w34 -> [w53 w1233]
      tunnel: [w51 w1237] -> w30
      tunnel: w33 -> [w52 w1235]
      tunnel: [w50 w1236] -> w32
      tunnel: w31 -> [w54 w1234]
      tunnel: [w49 w1232] -> w29
      frame False {
        w57 = FALSE
        # "generic data array\n\nused as storage during\nUploadSettings"
        # "timer for UploadSettings"
        # "initialize dataMTrig"
        # "NonExperiment"
        n26 = case shown="False" w52 {
          selector: w52 -> [_ w76]
          tunnel: w54 -> [w73 w78]
          tunnel: [w74 w78] -> w49
          tunnel: w53 -> [_ w77]
          tunnel: [w75 w77] -> w51
          tunnel: [w72 w76] -> w50
          frame False {
            n27 = call "myRIO__TCP_connect_forWriting.vi"("input_error"=w73) -> ("output_error"=w74:errorcluster, "output_connected"=w72:bool, "output_hTCP"=w75:refnum<k5>)  [unwired: 8 in]
          }
          frame True {
          }
        }
        n28 = call "myRIO_BRig_RT_dataMTrig_init.vi"() -> ("output_dataMTrig"=w68:u16[])  [unwired: 5 in]
        n29 = node-c288() -> (w71:T3)  [unwired: 4 in]
        n30 = timed-loop {
          timing: w71 -> [_]
          timing-out: [_] -> w70
          shift-right: [w115] -> _
          shift-left: w68 -> [w127]
          shift-right: [w109] -> _
          shift-left: myRIO_BRig_RT__Case_NonExp_stateList."Init" ("Enum") -> [w121]
          shift-right: [w103] -> _
          shift-left: w67 -> [w104]
          shift-right: [w101] -> _
          shift-left: w66 -> [w102]
          tunnel: [w123] -> w63
          tunnel: [w122] -> w61
          tunnel: w64 -> [w125]
          tunnel: w65 -> [w124]
          shift-right: [w120] -> _
          shift-left: u16[] [] ("output_data") -> [w119]
          shift-right: [w105] -> _
          shift-left: u16 0 ("Audio_Amp__L") -> [w106]
          shift-right: [w98] -> _
          shift-left: w57 -> [w100]
          shift-right: [w97] -> _
          shift-left: w57 -> [w99]
          shift-right: [w93] -> _
          shift-left: FALSE -> [w94]
          shift-right: [w91] -> _
          shift-left: 0.0 -> [w92]
          stop <- w128 stop-if-true
          n31 = node-c288() -> (w126:i64)  [unwired: 1 in]
          n32 = xnode "Read/Write Control"("FPGA VI Reference In"=w124, "error in"=w125) -> ("FPGA VI Reference Out"=w96:refnum<k20>, "error out"=w95:errorcluster, "A2_LickL"=w103:u32, "A4_LickR"=w101:u32)
          n33 = local write "A2"(w103) -> ()
          n34 = local write "A4"(w101) -> ()
          n35 = case shown="\"UploadSettings_dataExp_2\"" w121 {
            selector: w121 -> [_ w151 _ _ _ _ _ _ _ _ _ _ _ _ _ _ _ _ _ w840 w896 _ _ w1101 _ _ _ w1173 w1215]
            tunnel: [myRIO_BRig_RT__Case_NonExp_stateList."Idle" ("Enum") w149 w156 w175 w194 myRIO_BRig_RT__Case_NonExp_stateList."UploadSettings_dataExp_2" ("Enum") myRIO_BRig_RT__Case_NonExp_stateList."UploadSettings_Read_dataLC" ("Enum") myRIO_BRig_RT__Case_NonExp_stateList."UploadSettings_dataLC_2" ("Enum") myRIO_BRig_RT__Case_NonExp_stateList."UploadSettings_dataLC_4" ("Enum") myRIO_BRig_RT__Case_NonExp_stateList."UploadSettings_dataLC_3" ("f") myRIO_BRig_RT__Case_NonExp_stateList."UploadSettings_Read_dataMTrig" ("f") myRIO_BRig_RT__Case_NonExp_stateList."Idle" ("Enum") w600 w615 myRIO_BRig_RT__Case_NonExp_stateList."Idle_4" ("Enum") myRIO_BRig_RT__Case_NonExp_stateList."Idle_5" ("Enum") w712 w792 w802 w835 w891 myRIO_BRig_RT__Case_NonExp_stateList."DispenseWater_pre" ("Enum") w1047 w1099 w1121 myRIO_BRig_RT__Case_NonExp_stateList."Idle" ("Enum") myRIO_BRig_RT__Case_NonExp_stateList."Idle" ("Enum") w1172 w1215] -> w110
            tunnel: [w139 w148 w166 w185 w204 w266 w352 w405 w464 w517 w564 w580 w604 w630 w643 w698 w717 w790 w817 w841 w897 w958 w1084 w1106 w1132 w1166 w1171 w1183 w1213] -> w116
            tunnel: [_ _ _ _ _ _ _ _ _ _ _ _ _ _ _ _ _ _ _ _ _ _ _ _ _ _ _ _ TRUE] -> w128
            tunnel: w127 -> [_ w148 w166 w185 w204 w266 w352 w405 w464 w517 w564 w581 w603 w630 w643 w698 w718 w790 w818 w842 w898 w944 w1080 w1107 w1133 w1166 w1171 w1183 w1213]
            tunnel: w126 -> [_ _ _ _ _ _ _ _ _ _ _ _ _ _ _ _ _ _ _ _ _ _ _ w1111 _ _ _ _ _]
            tunnel: [_ _ w157 w176 w195 w215 w350 w406 w465 w513 w560 w565 _ _ _ _ _ _ w798 _ w885 _ _ _ _ _ _ _ _] -> w120
            tunnel: w119 -> [_ _ w158 w177 w196 w215 w350 w406 w465 w513 w560 w565 _ _ _ _ _ _ _ _ w886 _ _ _ _ _ _ _ _]
            tunnel: [_ _ _ _ _ _ _ _ _ _ _ _ _ _ _ _ _ _ _ _ _ _ _ w1108 _ _ _ _ _] -> w118
            tunnel: [_ _ _ _ _ _ _ _ _ _ _ _ _ _ _ _ _ _ _ _ _ _ _ w1090 _ _ _ _ _] -> w117
            tunnel: w106 -> [_ w155 _ _ _ _ _ _ _ _ _ _ _ _ _ _ _ _ _ _ _ _ _ _ _ _ _ _ _]
            tunnel: [_ w154 _ _ _ _ _ _ _ _ _ _ _ _ _ _ _ _ _ _ _ _ _ _ _ _ _ _ _] -> w105
            tunnel: w104 -> [_ _ _ _ _ _ _ _ _ _ _ _ _ _ _ _ _ _ _ w846 w902 _ _ _ _ _ _ _ _]
            tunnel: w103 -> [_ _ _ _ _ _ _ _ _ _ _ _ _ _ _ _ _ _ _ w847 w903 _ _ _ _ _ _ _ _]
            tunnel: w102 -> [_ _ _ _ _ _ _ _ _ _ _ _ _ _ _ _ _ _ _ w844 w900 _ _ _ _ _ _ _ _]
            tunnel: w101 -> [_ _ _ _ _ _ _ _ _ _ _ _ _ _ _ _ _ _ _ w845 w901 _ _ _ _ _ _ _ _]
            tunnel: w100 -> [_ _ _ _ _ _ _ _ _ _ _ _ _ _ _ _ _ _ _ w832 w888 _ _ _ _ _ _ _ _]
            tunnel: w99 -> [_ _ _ _ _ _ _ _ _ _ _ _ _ _ _ _ _ _ _ w831 w887 _ _ _ _ _ _ _ _]
            tunnel: [_ _ _ _ _ _ _ _ _ _ _ _ _ _ _ _ _ _ w800 w832 w888 _ _ _ _ _ _ _ _] -> w98
            tunnel: [_ _ _ _ _ _ _ _ _ _ _ _ _ _ _ _ _ _ w799 w831 w887 _ _ _ _ _ _ _ _] -> w97
            tunnel: w96 -> [_ _ _ _ _ _ _ _ _ _ _ _ w593 _ w664 w700 _ _ _ _ w884 _ _ _ _ _ _ w1178 _]
            tunnel: w95 -> [_ _ _ _ _ _ _ _ _ _ _ _ w592 _ w663 w699 _ _ _ _ w883 _ _ _ _ _ _ w1177 _]
            tunnel: w94 -> [_ _ _ _ _ _ _ _ _ _ _ _ _ _ _ _ _ _ _ _ _ _ _ _ _ _ _ w1182 _]
            tunnel: [_ _ _ _ _ _ _ _ _ _ _ _ _ _ _ _ _ _ _ _ _ _ _ _ _ _ _ TRUE _] -> w93
            tunnel: w92 -> [_ _ _ _ _ _ _ _ _ _ _ _ _ _ _ _ _ _ _ _ _ _ _ _ _ _ _ w1180 _]
            tunnel: [_ _ _ _ _ _ _ _ _ _ _ _ _ _ _ _ _ _ _ _ _ _ _ _ _ _ _ w1179 _] -> w91
            frame "Init", Default {
              w133 = FALSE ("RewCalib_Trig_L")
              w130 = u16 100 ("new element/subarray")
              # "Tdelay_R"
              # "Tdelay_L"
              # "RewCalib_N__R"
              # "RewCalib_N__L"
              # "Solenoid_Tcycle_R"
              # "Solenoid_Tcycle_L"
              # "Laser_Tcycle"
              # "Audio_Tcycle_R"
              # "Audio_Tcycle_L"
              # "initialize dataMTrig"
              n36 = call "myRIO_BRig_RT_dataMTrig_Solenoid_Tcycle__L.vi"() -> ("output_Solenoid_Tcycle__L"=w141:i32)  [unwired: 11 in]
              n37 = call "myRIO_BRig_RT_dataMTrig_Solenoid_Tcycle__R.vi"() -> ("output_Solenoid_Tcycle__R"=w142:i32)  [unwired: 11 in]
              n38 = call "myRIO_BRig_RT_dataMTrig_Audio_Tcycle__L.vi"() -> ("output_Audio_Tcycle__L"=w143:i32)  [unwired: 11 in]
              n39 = call "myRIO_BRig_RT_dataMTrig_Audio_Tcycle__R.vi"() -> ("output_Audio_Tcycle__R"=w144:i32)  [unwired: 11 in]
              n40 = call "myRIO_BRig_RT_dataMTrig_Laser_Tcycle.vi"() -> ("output_Laser_Tcycle"=w145:i32)  [unwired: 11 in]
              n41 = call "myRIO_BRig_RT_dataMTrig_Solenoid_RewCalib_nCycle__L.vi"() -> ("output_Solenoid_RewCalib_nCycle__L"=w137:i32)  [unwired: 11 in]
              n42 = call "myRIO_BRig_RT_dataMTrig_Solenoid_RewCalib_nCycle__R.vi"() -> ("output_Solenoid_RewCalib_nCycle__R"=w136:i32)  [unwired: 11 in]
              n43 = call "myRIO_BRig_RT_dataMTrig_Solenoid_Tdelay__L.vi"() -> ("output_Solenoid_Tdelay__L"=w135:i32)  [unwired: 11 in]
              n44 = call "myRIO_BRig_RT_dataMTrig_Solenoid_Tdelay__R.vi"() -> ("output_Solenoid_Tdelay__R"=w134:i32)  [unwired: 11 in]
              n45 = local read "MTrig_Solenoid_Tcycle__L"() -> (w146:u16)
              n46 = local read "MTrig_Solenoid_Tcycle__R"() -> (w147:u16)
              n47 = local read "MTrig_Laser_Tcycle"() -> (w131:u16)
              n48 = call "myRIO_BRig_RT_dataMTrig_init.vi"() -> ("output_dataMTrig"=w140:u16[])  [unwired: 5 in]
              n49 = local write "RewCalib_Trig_R"(w133) -> ()
              n50 = local write "RewCalib_Trig_L"(w133) -> ()
              n51 = local read "Tcycle_Cue_min"() -> (w132:u16)
              n52 = Replace Array Subset(array=w140, new element #1=w146, index #1=w141, new element #2=w147, index #2=w142, new element #3=w132, index #3=w143, new element #4=w132, index #4=w144, new element #5=w131, index #5=w145, new element #6=w130, index #6=w137, new element #7=w130, index #7=w136, new element #8=w130, index #8=w135, new element #9=w130, index #9=w134) -> (w139:u16[])
            }
            frame "UploadSettings_pre" {
              # "When the Host sends settings,\nnot all files send at the same time.\n\nIf RT reads the settings faster\nthan the Host can send them,\nthen we will skip settings.\n\nSolution:\nWait 20 cycles"
              n53 = Increment(x=w155) -> (x+1=w154:u16)
              n54 = Greater?(x=w154, y=u16 20) -> (0:w152:bool)
              n55 = Select(t=myRIO_BRig_RT__Case_NonExp_stateList."UploadSettings_Read_dataExp", s=w152, f=w151) -> (s? t:f=w149:T1)
            }
            frame "UploadSettings_Read_dataExp" {
              # "grab dataExp and\nstore it in the\ngeneric data array"
              # "dataExp"
              n56 = call "myRIO_BRig_RT_dataExp_init_details.vi"() -> ("output_dataSize"=w162:i32, "output_dataName"=w165:string)  [unwired: 10 in]
              n57 = call "myRIO_BRig_RT_comm_webdav_uploadReceived_check.vi"("input_dataName"=w165) -> ("output_Iexist"=w164:bool, "output_dataPath"=w163:path)  [unwired: 9 in]
              n58 = case shown="True" w164 {
                tunnel: w163 -> [_ w174]
                tunnel: w162 -> [_ w173]
                tunnel: [_ w172] -> w161
                tunnel: w158 -> [w167 w171]
                tunnel: [w167 w168] -> w157
                frame False {
                }
                frame True {
                  n59 = call "myRIO_BRig_RT_comm_webdav_uploadReceived_read.vi"("input_dataSize"=w173, "input_filePath"=w174) -> ("output_Ivalid"=w172:bool, "output_data"=w170:i64[])  [unwired: 8 in]
                  n60 = To Unsigned Word Integer(number=w170) -> (unsigned 16bit integer=w169:u16[])
                  n61 = Select(t=w169, s=w172, f=w171) -> (s? t:f=w168:u16[])
                }
              }
              n62 = Select(t=myRIO_BRig_RT__Case_NonExp_stateList."UploadSettings_dataExp_1", s=w161, f=myRIO_BRig_RT__Case_NonExp_stateList."UploadSettings_Read_dataLC" ("t")) -> (s? t:f=w156:T1)
            }
            frame "UploadSettings_Read_dataLC" {
              # "grab dataLC and\nstore it in the\ngeneric data array"
              # "dataLC"
              n63 = call "myRIO_BRig_RT_dataLC_init_details.vi"() -> ("output_dataSize"=w181:i32, "output_dataName"=w184:string)  [unwired: 10 in]
              n64 = call "myRIO_BRig_RT_comm_webdav_uploadReceived_check.vi"("input_dataName"=w184) -> ("output_Iexist"=w183:bool, "output_dataPath"=w182:path)  [unwired: 9 in]
              n65 = case shown="True" w183 {
                tunnel: w182 -> [_ w193]
                tunnel: w181 -> [_ w192]
                tunnel: [_ w191] -> w180
                tunnel: w177 -> [w186 w190]
                tunnel: [w186 w187] -> w176
                frame False {
                }
                frame True {
                  n66 = call "myRIO_BRig_RT_comm_webdav_uploadReceived_read.vi"("input_dataSize"=w192, "input_filePath"=w193) -> ("output_Ivalid"=w191:bool, "output_data"=w189:i64[])  [unwired: 8 in]
                  n67 = To Unsigned Word Integer(number=w189) -> (unsigned 16bit integer=w188:u16[])
                  n68 = Select(t=w188, s=w191, f=w190) -> (s? t:f=w187:u16[])
                }
              }
              n69 = Select(t=myRIO_BRig_RT__Case_NonExp_stateList."UploadSettings_dataLC_1", s=w180, f=myRIO_BRig_RT__Case_NonExp_stateList."UploadSettings_Read_dataMTrig" ("t")) -> (s? t:f=w175:T1)
            }
            frame "UploadSettings_Read_dataMTrig" {
              # "grab dataMTrig and\nstore it in the\ngeneric data array"
              # "dataMTrig"
              n70 = call "myRIO_BRig_RT_dataMTrig_init_details.vi"() -> ("output_dataSize"=w200:i32, "output_dataName"=w203:string)  [unwired: 10 in]
              n71 = call "myRIO_BRig_RT_comm_webdav_uploadReceived_check.vi"("input_dataName"=w203) -> ("output_Iexist"=w202:bool, "output_dataPath"=w201:path)  [unwired: 9 in]
              n72 = case shown="True" w202 {
                tunnel: w201 -> [_ w212]
                tunnel: w200 -> [_ w211]
                tunnel: [_ w210] -> w199
                tunnel: w196 -> [w205 w209]
                tunnel: [w205 w206] -> w195
                frame False {
                }
                frame True {
                  n73 = call "myRIO_BRig_RT_comm_webdav_uploadReceived_read.vi"("input_dataSize"=w211, "input_filePath"=w212) -> ("output_Ivalid"=w210:bool, "output_data"=w208:i64[])  [unwired: 8 in]
                  n74 = To Unsigned Word Integer(number=w208) -> (unsigned 16bit integer=w207:u16[])
                  n75 = Select(t=w207, s=w210, f=w209) -> (s? t:f=w206:u16[])
                }
              }
              n76 = Select(t=myRIO_BRig_RT__Case_NonExp_stateList."UploadSettings_dataMTrig_1", s=w199, f=myRIO_BRig_RT__Case_NonExp_stateList."Idle" ("t")) -> (s? t:f=w194:T1)
            }
            frame "UploadSettings_dataExp_1" {
              # "Cue_max"
              # "Cue_min"
              # "CuePenalty"
              # "Timeout"
              # "Wrong"
              # "Selection"
              # "RewardPost"
              # "Reward_R"
              # "Reward_L"
              # "Tcycle"
              # "TPB_min_R"
              # "TPB_min_L"
              # "TPB_max_R"
              # "TPB_max_L"
              # "I_trialUntilReward"
              # "ENL_penalty"
              # "ENL_min"
              # "ENL_max"
              # "BUR_max"
              # "BUR_min"
              # "CueCycles"
              # "Audio_Freq_R"
              # "Audio_Freq_L"
              # "Audio_Amp_R"
              # "Audio_Amp_L"
              n77 = call "myRIO_BRig_RT_dataExp_CueCycles.vi"() -> ("output_CueCycles"=w258:i32)  [unwired: 11 in]
              n78 = call "myRIO_BRig_RT_dataExp_Audio_amp__R.vi"() -> ("output_Audio_amp__R"=w262:i32)  [unwired: 11 in]
              n79 = call "myRIO_BRig_RT_dataExp_Audio_amp__L.vi"() -> ("output_Audio_amp__L"=w264:i32)  [unwired: 11 in]
              n80 = call "myRIO_BRig_RT_dataExp_Tcycle_Reward__L.vi"() -> ("output_Tcycle_Reward__L"=w235:i32)  [unwired: 11 in]
              n81 = call "myRIO_BRig_RT_dataExp_Tcycle_Reward__R.vi"() -> ("output_Tcycle_Reward__R"=w234:i32)  [unwired: 11 in]
              n82 = call "myRIO_BRig_RT_dataExp_Tcycle_RewardPost.vi"() -> ("output_Tcycle_RewardPost"=w233:i32)  [unwired: 11 in]
              n83 = call "myRIO_BRig_RT_dataExp_BUR_min.vi"() -> ("output_BUR_min"=w255:i32)  [unwired: 11 in]
              n84 = call "myRIO_BRig_RT_dataExp_ENL_min.vi"() -> ("output_ENL_min"=w251:i32)  [unwired: 11 in]
              n85 = call "myRIO_BRig_RT_dataExp_TPB_max__L.vi"() -> ("output_TPB_max__L"=w243:i32)  [unwired: 11 in]
              n86 = call "myRIO_BRig_RT_dataExp_TPB_max__R.vi"() -> ("output_TPB_max__R"=w242:i32)  [unwired: 11 in]
              n87 = call "myRIO_BRig_RT_dataExp_ENL_penalty.vi"() -> ("output_ENL_penalty"=w250:i32)  [unwired: 11 in]
              n88 = call "myRIO_BRig_RT_dataExp_Audio_freq__L.vi"() -> ("output_Audio_freq__L"=w260:i32)  [unwired: 11 in]
              n89 = call "myRIO_BRig_RT_dataExp_Audio_freq__R.vi"() -> ("output_Audio_freq__R"=w259:i32)  [unwired: 11 in]
              n90 = call "myRIO_BRig_RT_dataExp_BUR_max.vi"() -> ("output_BUR_max"=w256:i32)  [unwired: 11 in]
              n91 = call "myRIO_BRig_RT_dataExp_ENL_max.vi"() -> ("output_ENL_max"=w252:i32)  [unwired: 11 in]
              n92 = call "myRIO_BRig_RT_dataExp_ItrialUntilReward.vi"() -> ("output_I_trialUntilReward"=w246:i32)  [unwired: 11 in]
              n93 = call "myRIO_BRig_RT_dataExp_Tcycle_Selection.vi"() -> ("output_Tcycle_Selection"=w232:i32)  [unwired: 11 in]
              n94 = call "myRIO_BRig_RT_dataExp_Tcycle_Wrong.vi"() -> ("output_Tcycle_Wrong"=w231:i32)  [unwired: 11 in]
              n95 = call "myRIO_BRig_RT_dataExp_Tcycle_Timeout.vi"() -> ("output_Tcycle_Timeout"=w230:i32)  [unwired: 11 in]
              n96 = call "myRIO_BRig_RT_dataExp_TPB_min__L.vi"() -> ("output_TPB_min__L"=w241:i32)  [unwired: 11 in]
              n97 = call "myRIO_BRig_RT_dataExp_TPB_min__R.vi"() -> ("output_TPB_min__R"=w240:i32)  [unwired: 11 in]
              n98 = call "myRIO_BRig_RT_dataExp_Tcycle_CuePenalty.vi"() -> ("output_Tcycle_CuePenalty"=w223:i32)  [unwired: 11 in]
              n99 = call "myRIO_BRig_RT_dataExp_Tcycle_Cue_min.vi"() -> ("output_Tcycle_Cue_min"=w222:i32)  [unwired: 11 in]
              n100 = call "myRIO_BRig_RT_dataExp_Tcycle_Cue_max.vi"() -> ("output_Tcycle_Cue_max"=w221:i32)  [unwired: 11 in]
              n101 = Index Array(array=w215, index #1=w264, index #2=w262, index #3=w260, index #4=w259, index #5=w258, index #6=w256, index #7=w255, index #8=w252, index #9=w251, index #10=w250, index #11=w246, index #12=w243, index #13=w242, index #14=w241, index #15=w240, index #16=w235, index #17=w234, index #18=w233, index #19=w232, index #20=w231, index #21=w230, index #22=w223, index #23=w222, index #24=w221) -> (element #1=w263:u16, element #2=w261:u16, element #3=w218:u16, element #4=w217:u16, element #5=w257:u16, element #6=w254:u16, element #7=w253:u16, element #8=w249:u16, element #9=w248:u16, element #10=w247:u16, element #11=w244:u16, element #12=w239:u16, element #13=w238:u16, element #14=w237:u16, element #15=w236:u16, element #16=w229:u16, element #17=w228:u16, element #18=w227:u16, element #19=w226:u16, element #20=w225:u16, element #21=w224:u16, element #22=w220:u16, element #23=w214:u16, element #24=w213:u16)
              n102 = local write "Tcycle_Selection"(w226) -> ()
              n103 = local write "Tcycle_Wrong"(w225) -> ()
              n104 = local write "Tcycle_Timeout"(w224) -> ()
              n105 = local write "Audio_Amp__L"(w263) -> ()
              n106 = local write "Audio_Amp__R"(w261) -> ()
              n107 = local write "Tcycle_ENLPenalty"(w247) -> ()
              n108 = local write "Tcycle_ENL_max"(w249) -> ()
              n109 = local write "TpB_Min_L"(w237) -> ()
              n110 = local write "TpB_Min_R"(w236) -> ()
              n111 = local write "Tcycle_CuePenalty"(w220) -> ()
              n112 = local write "Tcycle_Cue_min"(w214) -> ()
              n113 = local write "Tcycle_Cue_max"(w213) -> ()
              n114 = To Unsigned Byte Integer(number=w218) -> (unsigned 8bit integer=w219:u8)
              n115 = To Unsigned Byte Integer(number=w217) -> (unsigned 8bit integer=w216:u8)
              n116 = Not Equal To 0?(x=w244) -> (x != 0?=w245:bool)
              n117 = local write "Tcycle_Reward_L"(w229) -> ()
              n118 = local write "Tcycle_Reward_R"(w228) -> ()
              n119 = local write "Tcycle_RewardPost"(w227) -> ()
              n120 = local write "CueCycles"(w257) -> ()
              n121 = local write "BUR_min"(w253) -> ()
              n122 = local write "BUR_max"(w254) -> ()
              n123 = local write "Tcycle_ENL_min"(w248) -> ()
              n124 = local write "TpB_Max_L"(w239) -> ()
              n125 = local write "TpB_Max_R"(w238) -> ()
              n126 = local write "TrialUntilReward"(w245) -> ()
              n127 = local write "Audio_Freq__L"(w219) -> ()
              n128 = local write "Audio_Freq__R"(w216) -> ()
            }
            frame "UploadSettings_dataExp_2" {
              w286 = 100.0 ("y")
              n129 = call "myRIO_BRig_RT_dataExp_FPGA_f_count2ms.vi"() -> ("output_FPGA_f_count2ms"=w349:i32)  [unwired: 11 in]
              n130 = call "myRIO_BRig_RT_dataExp_laser1_Freq.vi"() -> ("output_laser1_Freq"=w337:i32)  [unwired: 11 in]
              n131 = call "myRIO_BRig_RT_dataExp_laser1_duration.vi"() -> ("output_laser1_duration"=w336:i32)  [unwired: 11 in]
              n132 = call "myRIO_BRig_RT_dataExp_laser1_Tpeak.vi"() -> ("output_laser1_Tpeak"=w335:i32)  [unwired: 11 in]
              n133 = call "myRIO_BRig_RT_dataExp_laser1_Tshutter.vi"() -> ("output_laser1_Tshutter"=w334:i32)  [unwired: 11 in]
              n134 = call "myRIO_BRig_RT_dataExp_laser1_Power_min.vi"() -> ("output_laser1_Power_min"=w333:i32)  [unwired: 11 in]
              n135 = call "myRIO_BRig_RT_dataExp_laser1_Power_max.vi"() -> ("output_laser1_Power_max"=w332:i32)  [unwired: 11 in]
              n136 = call "myRIO_BRig_RT_dataExp_laser1_Power_step.vi"() -> ("output_laser1_Power_step"=w331:i32)  [unwired: 11 in]
              n137 = call "myRIO_BRig_RT_dataExp_Cue1Param_CueType_Switch.vi"() -> ("output_Cue1Param_CueType_Switch"=w278:i32)  [unwired: 11 in]
              n138 = call "myRIO_BRig_RT_dataExp_Cue1Param_AudioLed_Count_Switch.vi"() -> ("output_Cue1Param_AudioLed_Count_Switch"=w277:i32)  [unwired: 11 in]
              n139 = call "myRIO_BRig_RT_dataExp_Cue1Param_AudioLed_Probability_Switch.vi"() -> ("output_Cue1Param_AudioLed_Probability_Switch"=w276:i32)  [unwired: 11 in]
              n140 = call "myRIO_BRig_RT_dataExp_SolenoidProbability_L.vi"() -> ("output_SolenoidProbability_L"=w282:i32)  [unwired: 11 in]
              n141 = call "myRIO_BRig_RT_dataExp_SolenoidProbability_R.vi"() -> ("output_SolenoidProbability_R"=w281:i32)  [unwired: 11 in]
              n142 = call "myRIO_BRig_RT_dataExp_Cue1Param_CueType_NS.vi"() -> ("output_Cue1Param_CueType_NS"=w275:i32)  [unwired: 11 in]
              n143 = call "myRIO_BRig_RT_dataExp_Cue1Param_AudioLed_Count_NS.vi"() -> ("output_Cue1Param_AudioLed_Count_NS"=w274:i32)  [unwired: 11 in]
              n144 = call "myRIO_BRig_RT_dataExp_Cue1Param_AudioLed_Probability_NS.vi"() -> ("output_Cue1Param_AudioLed_Probability_NS"=w273:i32)  [unwired: 11 in]
              n145 = call "myRIO_BRig_RT_dataExp_laser2_Freq.vi"() -> ("output_laser2_Freq"=w330:i32)  [unwired: 11 in]
              n146 = call "myRIO_BRig_RT_dataExp_laser2_duration.vi"() -> ("output_laser2_duration"=w329:i32)  [unwired: 11 in]
              n147 = call "myRIO_BRig_RT_dataExp_laser2_Tpeak.vi"() -> ("output_laser2_Tpeak"=w328:i32)  [unwired: 11 in]
              n148 = call "myRIO_BRig_RT_dataExp_laser2_Tshutter.vi"() -> ("output_laser2_Tshutter"=w327:i32)  [unwired: 11 in]
              n149 = call "myRIO_BRig_RT_dataExp_laser2_Power_min.vi"() -> ("output_laser2_Power_min"=w326:i32)  [unwired: 11 in]
              n150 = call "myRIO_BRig_RT_dataExp_laser2_Power_max.vi"() -> ("output_laser2_Power_max"=w325:i32)  [unwired: 11 in]
              n151 = call "myRIO_BRig_RT_dataExp_laser2_Power_step.vi"() -> ("output_laser2_Power_step"=w324:i32)  [unwired: 11 in]
              n152 = call "myRIO_BRig_RT_dataExp_CueLed_Freq.vi"() -> ("output_CueLed_Freq"=w293:i32)  [unwired: 11 in]
              n153 = call "myRIO_BRig_RT_dataExp_CueLed_duration.vi"() -> ("output_CueLed_duration"=w292:i32)  [unwired: 11 in]
              n154 = call "myRIO_BRig_RT_dataExp_CueLed_Tpeak.vi"() -> ("output_CueLed_Tpeak"=w291:i32)  [unwired: 11 in]
              n155 = Index Array(array=w350, index #1=w349, index #2=w337, index #3=w336, index #4=w335, index #5=w334, index #6=w333, index #7=w332, index #8=w331, index #9=w330, index #10=w329, index #11=w328, index #12=w327, index #13=w326, index #14=w325, index #15=w324, index #16=w293, index #17=w292, index #18=w291, index #19=w282, index #20=w281, index #21=w278, index #22=w277, index #23=w276, index #24=w275, index #25=w274, index #26=w273) -> (element #1=w348:u16, element #2=w323:u16, element #3=w322:u16, element #4=w321:u16, element #5=w320:u16, element #6=w319:u16, element #7=w309:u16, element #8=w308:u16, element #9=w304:u16, element #10=w303:u16, element #11=w302:u16, element #12=w301:u16, element #13=w300:u16, element #14=w295:u16, element #15=w294:u16, element #16=w285:u16, element #17=w284:u16, element #18=w283:u16, element #19=w280:u16, element #20=w279:u16, element #21=w272:u16, element #22=w271:u16, element #23=w270:u16, element #24=w269:u16, element #25=w268:u16, element #26=w267:u16)
              n156 = local write "Cue1Param_CueType_Switch"(w272) -> ()
              n157 = local write "Cue1Param_AudioLed_Count_Switch"(w271) -> ()
              n158 = local write "Cue1Param_AudioLed_Probability_Switch"(w270) -> ()
              n159 = local write "Cue1Param_CueType_NS"(w269) -> ()
              n160 = local write "Cue1Param_AudioLed_Count_NS"(w268) -> ()
              n161 = local write "Cue1Param_AudioLed_Probability_NS"(w267) -> ()
              n162 = To Double Precision Float(number=w348) -> (double precision float=w347:dbl)
              n163 = To Double Precision Float(number=w323) -> (double precision float=w345:dbl)
              n164 = To Double Precision Float(number=w321) -> (double precision float=w342:dbl)
              n165 = To Double Precision Float(number=w320) -> (double precision float=w341:dbl)
              n166 = To Double Precision Float(number=w319) -> (double precision float=w343:dbl)
              n167 = To Double Precision Float(number=w309) -> (double precision float=w314:dbl)
              n168 = To Double Precision Float(number=w308) -> (double precision float=w310:dbl)
              n169 = To Double Precision Float(number=w304) -> (double precision float=w315:dbl)
              n170 = To Double Precision Float(number=w302) -> (double precision float=w317:dbl)
              n171 = To Double Precision Float(number=w301) -> (double precision float=w318:dbl)
              n172 = To Double Precision Float(number=w300) -> (double precision float=w316:dbl)
              n173 = To Double Precision Float(number=w295) -> (double precision float=w298:dbl)
              n174 = To Double Precision Float(number=w294) -> (double precision float=w299:dbl)
              n175 = To Double Precision Float(number=w285) -> (double precision float=w290:dbl)
              n176 = To Double Precision Float(number=w283) -> (double precision float=w289:dbl)
              n177 = local write "SolenoidProbability_L"(w280) -> ()
              n178 = local write "SolenoidProbability_R"(w279) -> ()
              n179 = Divide(x=w347, y=w286) -> (x/y=w346:dbl)
              n180 = Divide(x=w345, y=w286) -> (x/y=w344:dbl)
              n181 = Divide(x=w342, y=w286) -> (x/y=w339:dbl)
              n182 = Divide(x=w341, y=w286) -> (x/y=w338:dbl)
              n183 = Divide(x=w343, y=w286) -> (x/y=w340:dbl)
              n184 = Divide(x=w314, y=w286) -> (x/y=w312:dbl)
              n185 = Divide(x=w310, y=w286) -> (x/y=w311:dbl)
              n186 = Divide(x=w315, y=w286) -> (x/y=w313:dbl)
              n187 = Divide(x=w317, y=w286) -> (x/y=w307:dbl)
              n188 = Divide(x=w318, y=w286) -> (x/y=w306:dbl)
              n189 = Divide(x=w316, y=w286) -> (x/y=w305:dbl)
              n190 = Divide(x=w298, y=w286) -> (x/y=w297:dbl)
              n191 = Divide(x=w299, y=w286) -> (x/y=w296:dbl)
              n192 = Divide(x=w290, y=w286) -> (x/y=w288:dbl)
              n193 = Divide(x=w289, y=w286) -> (x/y=w287:dbl)
              n194 = local write "FPGA_count2ms"(w346) -> ()
              n195 = local write "Laser_Freq_l1"(w344) -> ()
              n196 = local write "Laser_duration_l1"(w322) -> ()
              n197 = local write "Laser_Tpeak_l1"(w339) -> ()
              n198 = local write "Laser_Tshutter_l1"(w338) -> ()
              n199 = local write "Laser_power_min_l1"(w340) -> ()
              n200 = local write "Laser_power_max_l1"(w312) -> ()
              n201 = local write "Laser_power_step_l1"(w311) -> ()
              n202 = local write "Laser_Freq_l2"(w313) -> ()
              n203 = local write "Laser_duration_l2"(w303) -> ()
              n204 = local write "Laser_Tpeak_l2"(w307) -> ()
              n205 = local write "Laser_Tshutter_l2"(w306) -> ()
              n206 = local write "Laser_power_min_l2"(w305) -> ()
              n207 = local write "Laser_power_max_l2"(w297) -> ()
              n208 = local write "Laser_power_step_l2"(w296) -> ()
              n209 = local write "CueLed_Freq"(w288) -> ()
              n210 = local write "CueLed_duration"(w284) -> ()
              n211 = local write "CueLed_Tpeak"(w287) -> ()
            }
            frame "UploadSettings_dataLC_1" {
              # "Cue1_delayOpt_NonSwitch"
              # "ENL1_delayOpt_NonSwitch"
              # "Cue1_delayOpt_Switch"
              # "ENL1_delayOpt_Switch"
              # "Count"
              # "Tdelay"
              # "Prob"
              # "OnOff"
              # "Block"
              # "Count"
              # "Tdelay"
              # "Prob"
              # "OnOff"
              # "Block"
              # "Count"
              # "Tdelay"
              # "Prob"
              # "OnOff"
              # "Block"
              # "ENL1 Switch"
              # "Cue1 NonSwitch"
              # "Cue1 Switch"
              # "ENL1 NonSwitch"
              # "Count"
              # "Tdelay"
              # "Prob"
              # "OnOff"
              # "Block"
              n212 = call "myRIO_BRig_RT_dataLC_ENL1_OnOff_Switch_l1.vi"() -> ("output_ENL1_OnOff_Switch_l1"=w404:i32)  [unwired: 11 in]
              n213 = call "myRIO_BRig_RT_dataLC_ENL1_Tdelay_Switch_l1.vi"() -> ("output_ENL1_Tdelay_Switch_l1"=w403:i32)  [unwired: 11 in]
              n214 = call "myRIO_BRig_RT_dataLC_ENL1_Block_Switch_l1.vi"() -> ("output_ENL1_Block_Switch_l1"=w402:i32)  [unwired: 11 in]
              n215 = call "myRIO_BRig_RT_dataLC_ENL1_Count_Switch_l1.vi"() -> ("output_ENL1_Count_Switch_l1"=w401:i32)  [unwired: 11 in]
              n216 = call "myRIO_BRig_RT_dataLC_ENL1_Probability_Switch_l1.vi"() -> ("output_ENL1_Probability_Switch_l1"=w400:i32)  [unwired: 11 in]
              n217 = call "myRIO_BRig_RT_dataLC_ENL1_OnOff_NS_l1.vi"() -> ("output_ENL1_OnOff_NS_l1"=w399:i32)  [unwired: 11 in]
              n218 = call "myRIO_BRig_RT_dataLC_ENL1_Tdelay_NS_l1.vi"() -> ("output_ENL1_Tdelay_NS_l1"=w398:i32)  [unwired: 11 in]
              n219 = call "myRIO_BRig_RT_dataLC_ENL1_Block_NS_l1.vi"() -> ("output_ENL1_All_Block"=w397:i32)  [unwired: 11 in]
              n220 = call "myRIO_BRig_RT_dataLC_ENL1_Count_NS_l1.vi"() -> ("output_ENL1_Count_NS_l1"=w396:i32)  [unwired: 11 in]
              n221 = call "myRIO_BRig_RT_dataLC_ENL1_Probability_NS_l1.vi"() -> ("output_ENL1_Probability_NS_l1"=w395:i32)  [unwired: 11 in]
              n222 = call "myRIO_BRig_RT_dataLC_Cue1_OnOff_Switch_l1.vi"() -> ("output_Cue1_OnOff_Switch_l1"=w394:i32)  [unwired: 11 in]
              n223 = call "myRIO_BRig_RT_dataLC_Cue1_Tdelay_Switch_l1.vi"() -> ("output_Cue1_Tdelay_Switch_l1"=w393:i32)  [unwired: 11 in]
              n224 = call "myRIO_BRig_RT_dataLC_Cue1_Block_Switch_l1.vi"() -> ("output_Cue1_Block_Switch_l1"=w392:i32)  [unwired: 11 in]
              n225 = call "myRIO_BRig_RT_dataLC_Cue1_Count_Switch_l1.vi"() -> ("output_Cue1_Count_Switch_l1"=w391:i32)  [unwired: 11 in]
              n226 = call "myRIO_BRig_RT_dataLC_Cue1_Probability_Switch_l1.vi"() -> ("output_Cue1_Probability_Switch_l1"=w390:i32)  [unwired: 11 in]
              n227 = call "myRIO_BRig_RT_dataLC_Cue1_OnOff_NS_l1.vi"() -> ("output_Cue1_OnOff_NS_l1"=w389:i32)  [unwired: 11 in]
              n228 = call "myRIO_BRig_RT_dataLC_Cue1_Tdelay_NS_l1.vi"() -> ("output_Cue1_Tdelay_NS_l1"=w388:i32)  [unwired: 11 in]
              n229 = call "myRIO_BRig_RT_dataLC_Cue1_Block_NS_l1.vi"() -> ("output_Cue1_Block_NS_l1"=w387:i32)  [unwired: 11 in]
              n230 = call "myRIO_BRig_RT_dataLC_Cue1_Count_NS_l1.vi"() -> ("output_Cue1_Count_NS_l1"=w386:i32)  [unwired: 11 in]
              n231 = call "myRIO_BRig_RT_dataLC_Cue1_Probability_NS_l1.vi"() -> ("output_Cue1_l1_All_Probability"=w385:i32)  [unwired: 11 in]
              n232 = call "myRIO_BRig_RT_dataLC_ENL1_delayOpt_Switch_l1.vi"() -> ("output_ENL1_delayOpt_Switch_l1"=w364:i32)  [unwired: 11 in]
              n233 = call "myRIO_BRig_RT_dataLC_ENL1_delayOpt_NS_l1.vi"() -> ("output_ENL1_delayOpt_NS_l1"=w363:i32)  [unwired: 11 in]
              n234 = call "myRIO_BRig_RT_dataLC_Cue1_delayOpt_Switch_l1.vi"() -> ("output_Cue1_delayOpt_Switch_l1"=w362:i32)  [unwired: 11 in]
              n235 = call "myRIO_BRig_RT_dataLC_Cue1_delayOpt_NS_l1.vi"() -> ("output_Cue1_delayOpt_NS_l1"=w361:i32)  [unwired: 11 in]
              n236 = Index Array(array=w406, index #1=w404, index #2=w403, index #3=w402, index #4=w401, index #5=w400, index #6=w399, index #7=w398, index #8=w397, index #9=w396, index #10=w395, index #11=w394, index #12=w393, index #13=w392, index #14=w391, index #15=w390, index #16=w389, index #17=w388, index #18=w387, index #19=w386, index #20=w385, index #21=w364, index #22=w363, index #23=w362, index #24=w361) -> (element #1=w384:u16, element #2=w383:u16, element #3=w382:u16, element #4=w381:u16, element #5=w380:u16, element #6=w379:u16, element #7=w378:u16, element #8=w377:u16, element #9=w376:u16, element #10=w375:u16, element #11=w374:u16, element #12=w373:u16, element #13=w372:u16, element #14=w371:u16, element #15=w370:u16, element #16=w369:u16, element #17=w368:u16, element #18=w367:u16, element #19=w366:u16, element #20=w365:u16, element #21=w356:u16, element #22=w355:u16, element #23=w354:u16, element #24=w353:u16)
              n237 = Not Equal To 0?(x=w384) -> (x != 0?=w408:bool)
              n238 = Not Equal To 0?(x=w379) -> (x != 0?=w407:bool)
              n239 = Not Equal To 0?(x=w374) -> (x != 0?=w410:bool)
              n240 = Not Equal To 0?(x=w369) -> (x != 0?=w409:bool)
              n241 = Not Equal To 0?(x=w356) -> (x != 0?=w358:bool)
              n242 = Not Equal To 0?(x=w355) -> (x != 0?=w359:bool)
              n243 = Not Equal To 0?(x=w354) -> (x != 0?=w360:bool)
              n244 = Not Equal To 0?(x=w353) -> (x != 0?=w357:bool)
              n245 = local write "LC_ENL1_OnOff_Switch_l1"(w408) -> ()
              n246 = local write "LC_ENL1_Tdelay_Switch_l1"(w383) -> ()
              n247 = local write "LC_ENL1_Block_Switch_l1"(w382) -> ()
              n248 = local write "LC_ENL1_Count_Switch_l1"(w381) -> ()
              n249 = local write "LC_ENL1_Probability_Switch_l1"(w380) -> ()
              n250 = local write "LC_ENL1_OnOff_NS_l1"(w407) -> ()
              n251 = local write "LC_ENL1_Tdelay_NS_l1"(w378) -> ()
              n252 = local write "LC_ENL1_Block_NS_l1"(w377) -> ()
              n253 = local write "LC_ENL1_Count_NS_l1"(w376) -> ()
              n254 = local write "LC_ENL1_Probability_NS_l1"(w375) -> ()
              n255 = local write "LC_Cue1_OnOff_Switch_l1"(w410) -> ()
              n256 = local write "LC_Cue1_Tdelay_Switch_l1"(w373) -> ()
              n257 = local write "LC_Cue1_Block_Switch_l1"(w372) -> ()
              n258 = local write "LC_Cue1_Count_Switch_l1"(w371) -> ()
              n259 = local write "LC_Cue1_Probability_Switch_l1"(w370) -> ()
              n260 = local write "LC_Cue1_OnOff_NS_l1"(w409) -> ()
              n261 = local write "LC_Cue1_Tdelay_NS_l1"(w368) -> ()
              n262 = local write "LC_Cue1_Block_NS_l1"(w367) -> ()
              n263 = local write "LC_Cue1_Count_NS_l1"(w366) -> ()
              n264 = local write "LC_Cue1_Probability_NS_l1"(w365) -> ()
              n265 = local write "LC_ENL1_delayOpt_Switch_l1"(w358) -> ()
              n266 = local write "LC_ENL1_delayOpt_NS_l1"(w359) -> ()
              n267 = local write "LC_Cue1_delayOpt_Switch_l1"(w360) -> ()
              n268 = local write "LC_Cue1_delayOpt_NS_l1"(w357) -> ()
            }
            frame "UploadSettings_dataLC_3" {
              # "Cue1_delayOpt_NonSwitch"
              # "ENL1_delayOpt_NonSwitch"
              # "Cue1_delayOpt_Switch"
              # "ENL1_delayOpt_Switch"
              # "Count"
              # "Tdelay"
              # "Prob"
              # "OnOff"
              # "Block"
              # "Count"
              # "Tdelay"
              # "Prob"
              # "OnOff"
              # "Block"
              # "Count"
              # "Tdelay"
              # "Prob"
              # "OnOff"
              # "Block"
              # "ENL1 Switch"
              # "Cue1 NonSwitch"
              # "Cue1 Switch"
              # "ENL1 NonSwitch"
              # "Count"
              # "Tdelay"
              # "Prob"
              # "OnOff"
              # "Block"
              n269 = call "myRIO_BRig_RT_dataLC_ENL1_OnOff_Switch_l2.vi"() -> ("output_ENL1_OnOff_Switch_l2"=w431:i32)  [unwired: 11 in]
              n270 = call "myRIO_BRig_RT_dataLC_ENL1_Tdelay_Switch_l2.vi"() -> ("output_ENL1_Tdelay_Switch_l2"=w432:i32)  [unwired: 11 in]
              n271 = call "myRIO_BRig_RT_dataLC_ENL1_Block_Switch_l2.vi"() -> ("output_ENL1_Block_Switch_l2"=w433:i32)  [unwired: 11 in]
              n272 = call "myRIO_BRig_RT_dataLC_ENL1_Count_Switch_l2.vi"() -> ("output_ENL1_Count_Switch_l2"=w434:i32)  [unwired: 11 in]
              n273 = call "myRIO_BRig_RT_dataLC_ENL1_Probability_Switch_l2.vi"() -> ("output_ENL1_Probability_Switch_l2"=w435:i32)  [unwired: 11 in]
              n274 = call "myRIO_BRig_RT_dataLC_ENL1_OnOff_NS_l2.vi"() -> ("output_ENL1_OnOff_NS_l2"=w426:i32)  [unwired: 11 in]
              n275 = call "myRIO_BRig_RT_dataLC_ENL1_Tdelay_NS_l2.vi"() -> ("output_ENL1_Tdelay_NS_l2"=w427:i32)  [unwired: 11 in]
              n276 = call "myRIO_BRig_RT_dataLC_ENL1_Block_NS_l2.vi"() -> ("output_ENL1_Block_NS_l2"=w428:i32)  [unwired: 11 in]
              n277 = call "myRIO_BRig_RT_dataLC_ENL1_Count_NS_l2.vi"() -> ("output_ENL1_Count_NS_l2"=w429:i32)  [unwired: 11 in]
              n278 = call "myRIO_BRig_RT_dataLC_ENL1_Probability_NS_l2.vi"() -> ("output_ENL1_Probability_NS_l2"=w430:i32)  [unwired: 11 in]
              n279 = call "myRIO_BRig_RT_dataLC_Cue1_OnOff_Switch_l2.vi"() -> ("output_Cue1_OnOff_Switch_l2"=w421:i32)  [unwired: 11 in]
              n280 = call "myRIO_BRig_RT_dataLC_Cue1_Tdelay_Switch_l2.vi"() -> ("output_Cue1_Tdelay_Switch_l2"=w422:i32)  [unwired: 11 in]
              n281 = call "myRIO_BRig_RT_dataLC_Cue1_Block_Switch_l2.vi"() -> ("output_Cue1_Block_Switch_l2"=w423:i32)  [unwired: 11 in]
              n282 = call "myRIO_BRig_RT_dataLC_Cue1_Count_Switch_l2.vi"() -> ("output_Cue1_Count_Switch_l2"=w424:i32)  [unwired: 11 in]
              n283 = call "myRIO_BRig_RT_dataLC_Cue1_Probability_Switch_l2.vi"() -> ("output_Cue1_l2_First_Probability"=w425:i32)  [unwired: 11 in]
              n284 = call "myRIO_BRig_RT_dataLC_Cue1_OnOff_NS_l2.vi"() -> ("output_Cue1_OnOff_NS_l2"=w416:i32)  [unwired: 11 in]
              n285 = call "myRIO_BRig_RT_dataLC_Cue1_Tdelay_NS_l2.vi"() -> ("output_Cue1_Tdelay_NS_l2"=w417:i32)  [unwired: 11 in]
              n286 = call "myRIO_BRig_RT_dataLC_Cue1_Block_NS_l2.vi"() -> ("output_Cue1_Block_NS_l2"=w418:i32)  [unwired: 11 in]
              n287 = call "myRIO_BRig_RT_dataLC_Cue1_Count_NS_l2.vi"() -> ("output_Cue1_Count_NS_l2"=w419:i32)  [unwired: 11 in]
              n288 = call "myRIO_BRig_RT_dataLC_Cue1_Probability_NS_l2.vi"() -> ("output_Cue1_l2_All_Probability"=w420:i32)  [unwired: 11 in]
              n289 = call "myRIO_BRig_RT_dataLC_ENL1_delayOpt_Switch_l2.vi"() -> ("output_ENL1_delayOpt_Switch_l2"=w412:i32)  [unwired: 11 in]
              n290 = call "myRIO_BRig_RT_dataLC_ENL1_delayOpt_NS_l2.vi"() -> ("output_ENL1_delayOpt_NS_l2"=w413:i32)  [unwired: 11 in]
              n291 = call "myRIO_BRig_RT_dataLC_Cue1_delayOpt_Switch_l2.vi"() -> ("output_Cue1_delayOpt_Switch_l2"=w414:i32)  [unwired: 11 in]
              n292 = call "myRIO_BRig_RT_dataLC_Cue1_delayOpt_NS_l2.vi"() -> ("output_Cue1_delayOpt_NS_l2"=w415:i32)  [unwired: 11 in]
              n293 = Index Array(array=w465, index #1=w431, index #2=w432, index #3=w433, index #4=w434, index #5=w435, index #6=w426, index #7=w427, index #8=w428, index #9=w429, index #10=w430, index #11=w421, index #12=w422, index #13=w423, index #14=w424, index #15=w425, index #16=w416, index #17=w417, index #18=w418, index #19=w419, index #20=w420, index #21=w412, index #22=w413, index #23=w414, index #24=w415) -> (element #1=w463:u16, element #2=w462:u16, element #3=w461:u16, element #4=w460:u16, element #5=w459:u16, element #6=w458:u16, element #7=w457:u16, element #8=w456:u16, element #9=w455:u16, element #10=w454:u16, element #11=w453:u16, element #12=w452:u16, element #13=w451:u16, element #14=w450:u16, element #15=w449:u16, element #16=w448:u16, element #17=w447:u16, element #18=w446:u16, element #19=w445:u16, element #20=w444:u16, element #21=w439:u16, element #22=w438:u16, element #23=w437:u16, element #24=w436:u16)
              n294 = Not Equal To 0?(x=w463) -> (x != 0?=w467:bool)
              n295 = Not Equal To 0?(x=w458) -> (x != 0?=w466:bool)
              n296 = Not Equal To 0?(x=w453) -> (x != 0?=w469:bool)
              n297 = Not Equal To 0?(x=w448) -> (x != 0?=w468:bool)
              n298 = Not Equal To 0?(x=w439) -> (x != 0?=w441:bool)
              n299 = Not Equal To 0?(x=w438) -> (x != 0?=w442:bool)
              n300 = Not Equal To 0?(x=w437) -> (x != 0?=w443:bool)
              n301 = Not Equal To 0?(x=w436) -> (x != 0?=w440:bool)
              n302 = local write "LC_ENL1_OnOff_Switch_l2"(w467) -> ()
              n303 = local write "LC_ENL1_Tdelay_Switch_l2"(w462) -> ()
              n304 = local write "LC_ENL1_Block_Switch_l2"(w461) -> ()
              n305 = local write "LC_ENL1_Count_Switch_l2"(w460) -> ()
              n306 = local write "LC_ENL1_Probability_Switch_l2"(w459) -> ()
              n307 = local write "LC_ENL1_OnOff_NS_l2"(w466) -> ()
              n308 = local write "LC_ENL1_Tdelay_NS_l2"(w457) -> ()
              n309 = local write "LC_ENL1_Block_NS_l2"(w456) -> ()
              n310 = local write "LC_ENL1_Count_NS_l2"(w455) -> ()
              n311 = local write "LC_ENL1_Probability_NS_l2"(w454) -> ()
              n312 = local write "LC_Cue1_OnOff_Switch_l2"(w469) -> ()
              n313 = local write "LC_Cue1_Tdelay_Switch_l2"(w452) -> ()
              n314 = local write "LC_Cue1_Block_Switch_l2"(w451) -> ()
              n315 = local write "LC_Cue1_Count_Switch_l2"(w450) -> ()
              n316 = local write "LC_Cue1_Probability_Switch_l2"(w449) -> ()
              n317 = local write "LC_Cue1_OnOff_NS_l2"(w468) -> ()
              n318 = local write "LC_Cue1_Tdelay_NS_l2"(w447) -> ()
              n319 = local write "LC_Cue1_Block_NS_l2"(w446) -> ()
              n320 = local write "LC_Cue1_Count_NS_l2"(w445) -> ()
              n321 = local write "LC_Cue1_Probability_NS_l2"(w444) -> ()
              n322 = local write "LC_ENL1_delayOpt_Switch_l2"(w441) -> ()
              n323 = local write "LC_ENL1_delayOpt_NS_l2"(w442) -> ()
              n324 = local write "LC_Cue1_delayOpt_Switch_l2"(w443) -> ()
              n325 = local write "LC_Cue1_delayOpt_NS_l2"(w440) -> ()
            }
            frame "UploadSettings_dataLC_2" {
              # "Count"
              # "Tdelay"
              # "Prob"
              # "OnOff"
              # "Block"
              # "Selection NonSwitch"
              # "Count"
              # "Tdelay"
              # "Prob"
              # "OnOff"
              # "Block"
              # "Selection Switch"
              # "Trial"
              # "Tdelay"
              # "Prob"
              # "OnOff"
              # "Block"
              # "Wrong"
              # "Reward"
              # "Trial"
              # "Tdelay"
              # "Prob"
              # "OnOff"
              # "Block"
              n326 = call "myRIO_BRig_RT_dataLC_Reward_OnOff_l1.vi"() -> ("output_Reward_OnOff_l1"=w512:i32)  [unwired: 11 in]
              n327 = call "myRIO_BRig_RT_dataLC_Reward_Tdelay_l1.vi"() -> ("output_Reward_Tdelay_l1"=w511:i32)  [unwired: 11 in]
              n328 = call "myRIO_BRig_RT_dataLC_Reward_Block_l1.vi"() -> ("output_Reward_Block_l1"=w510:i32)  [unwired: 11 in]
              n329 = call "myRIO_BRig_RT_dataLC_Reward_Trial_l1.vi"() -> ("output_Reward_Trial_l1"=w509:i32)  [unwired: 11 in]
              n330 = call "myRIO_BRig_RT_dataLC_Reward_Probability_l1.vi"() -> ("output_Reward_Probability_l1"=w508:i32)  [unwired: 11 in]
              n331 = call "myRIO_BRig_RT_dataLC_Wrong_OnOff_l1.vi"() -> ("output_Wrong_OnOff_l1"=w501:i32)  [unwired: 11 in]
              n332 = call "myRIO_BRig_RT_dataLC_Wrong_Tdelay_l1.vi"() -> ("output_Wrong_Tdelay_l1"=w500:i32)  [unwired: 11 in]
              n333 = call "myRIO_BRig_RT_dataLC_Wrong_Block_l1.vi"() -> ("output_Wrong_Block_l1"=w499:i32)  [unwired: 11 in]
              n334 = call "myRIO_BRig_RT_dataLC_Wrong_Trial_l1.vi"() -> ("output_Wrong_Trial_l1"=w498:i32)  [unwired: 11 in]
              n335 = call "myRIO_BRig_RT_dataLC_Wrong_Probability_l1.vi"() -> ("output_Wrong_Probability_l1"=w497:i32)  [unwired: 11 in]
              n336 = call "myRIO_BRig_RT_dataLC_Selection_OnOff_Switch_l1.vi"() -> ("output_Selection_OnOff_Switch_l1"=w492:i32)  [unwired: 11 in]
              n337 = call "myRIO_BRig_RT_dataLC_Selection_Tdelay_Switch_l1.vi"() -> ("output_Selection_Tdelay_Switch_l1"=w491:i32)  [unwired: 11 in]
              n338 = call "myRIO_BRig_RT_dataLC_Selection_Block_Switch_l1.vi"() -> ("output_Selection_Block_Switch_l1"=w490:i32)  [unwired: 11 in]
              n339 = call "myRIO_BRig_RT_dataLC_Selection_Count_Switch_l1.vi"() -> ("output_Selection_Count_Switch_l1"=w489:i32)  [unwired: 11 in]
              n340 = call "myRIO_BRig_RT_dataLC_Selection_Probability_Switch_l1.vi"() -> ("output_Selection_Probability_Switch_l1"=w488:i32)  [unwired: 11 in]
              n341 = call "myRIO_BRig_RT_dataLC_Selection_OnOff_NS_l1.vi"() -> ("output_Selection_OnOff_NS_l1"=w487:i32)  [unwired: 11 in]
              n342 = call "myRIO_BRig_RT_dataLC_Selection_Tdelay_NS_l1.vi"() -> ("output_Selection_Tdelay_NS_l1"=w486:i32)  [unwired: 11 in]
              n343 = call "myRIO_BRig_RT_dataLC_Selection_Block_NS_l1.vi"() -> ("output_Selection_Block_NS_l1"=w485:i32)  [unwired: 11 in]
              n344 = call "myRIO_BRig_RT_dataLC_Selection_Count_NS_l1.vi"() -> ("output_Selection_Count_NS_l1"=w484:i32)  [unwired: 11 in]
              n345 = call "myRIO_BRig_RT_dataLC_Selection_Probability_NS_l1.vi"() -> ("output_Selection_Probability_NS_l1"=w483:i32)  [unwired: 11 in]
              n346 = Index Array(array=w513, index #1=w512, index #2=w511, index #3=w510, index #4=w509, index #5=w508, index #6=w501, index #7=w500, index #8=w499, index #9=w498, index #10=w497, index #11=w492, index #12=w491, index #13=w490, index #14=w489, index #15=w488, index #16=w487, index #17=w486, index #18=w485, index #19=w484, index #20=w483) -> (element #1=w507:u16, element #2=w506:u16, element #3=w505:u16, element #4=w504:u16, element #5=w503:u16, element #6=w502:u16, element #7=w496:u16, element #8=w495:u16, element #9=w494:u16, element #10=w493:u16, element #11=w480:u16, element #12=w479:u16, element #13=w478:u16, element #14=w477:u16, element #15=w476:u16, element #16=w475:u16, element #17=w474:u16, element #18=w473:u16, element #19=w472:u16, element #20=w471:u16)
              n347 = Not Equal To 0?(x=w507) -> (x != 0?=w515:bool)
              n348 = Not Equal To 0?(x=w502) -> (x != 0?=w514:bool)
              n349 = Not Equal To 0?(x=w480) -> (x != 0?=w482:bool)
              n350 = Not Equal To 0?(x=w475) -> (x != 0?=w481:bool)
              n351 = local write "LC_Reward_OnOff_l1"(w515) -> ()
              n352 = local write "LC_Reward_Tdelay_l1"(w506) -> ()
              n353 = local write "LC_Reward_Block_l1"(w505) -> ()
              n354 = local write "LC_Reward_Trial_l1"(w504) -> ()
              n355 = local write "LC_Reward_Probability_l1"(w503) -> ()
              n356 = local write "LC_Wrong_OnOff_l1"(w514) -> ()
              n357 = local write "LC_Wrong_Tdelay_l1"(w496) -> ()
              n358 = local write "LC_Wrong_Block_l1"(w495) -> ()
              n359 = local write "LC_Wrong_Trial_l1"(w494) -> ()
              n360 = local write "LC_Wrong_Probability_l1"(w493) -> ()
              n361 = local write "LC_Sel_OnOff_Switch_l1"(w482) -> ()
              n362 = local write "LC_Sel_Tdelay_Switch_l1"(w479) -> ()
              n363 = local write "LC_Sel_Block_Switch_l1"(w478) -> ()
              n364 = local write "LC_Sel_Count_Switch_l1"(w477) -> ()
              n365 = local write "LC_Sel_Probability_Switch_l1"(w476) -> ()
              n366 = local write "LC_Sel_OnOff_NS_l1"(w481) -> ()
              n367 = local write "LC_Sel_Tdelay_NS_l1"(w474) -> ()
              n368 = local write "LC_Sel_Block_NS_l1"(w473) -> ()
              n369 = local write "LC_Sel_Count_NS_l1"(w472) -> ()
              n370 = local write "LC_Sel_Probability_NS_l1"(w471) -> ()
            }
            frame "UploadSettings_dataLC_4" {
              # "Count"
              # "Tdelay"
              # "Prob"
              # "OnOff"
              # "Block"
              # "Selection NonSwitch"
              # "Count"
              # "Tdelay"
              # "Prob"
              # "OnOff"
              # "Block"
              # "Selection Switch"
              # "Trial"
              # "Tdelay"
              # "Prob"
              # "OnOff"
              # "Block"
              # "Wrong"
              # "Reward"
              # "Trial"
              # "Tdelay"
              # "Prob"
              # "OnOff"
              # "Block"
              n371 = call "myRIO_BRig_RT_dataLC_Reward_OnOff_l2.vi"() -> ("output_Reward_OnOff_l2"=w523:i32)  [unwired: 11 in]
              n372 = call "myRIO_BRig_RT_dataLC_Reward_Tdelay_l2.vi"() -> ("output_Reward_Tdelay_l2"=w524:i32)  [unwired: 11 in]
              n373 = call "myRIO_BRig_RT_dataLC_Reward_Block_l2.vi"() -> ("output_Reward_Block_l2"=w525:i32)  [unwired: 11 in]
              n374 = call "myRIO_BRig_RT_dataLC_Reward_Trial_l2.vi"() -> ("output_Reward_Trial_l2"=w526:i32)  [unwired: 11 in]
              n375 = call "myRIO_BRig_RT_dataLC_Reward_Probability_l2.vi"() -> ("output_Reward_Probability_l2"=w527:i32)  [unwired: 11 in]
              n376 = call "myRIO_BRig_RT_dataLC_Wrong_OnOff_l2.vi"() -> ("output_Wrong_OnOff_l2"=w518:i32)  [unwired: 11 in]
              n377 = call "myRIO_BRig_RT_dataLC_Wrong_Tdelay_l2.vi"() -> ("output_Wrong_Tdelay_l2"=w519:i32)  [unwired: 11 in]
              n378 = call "myRIO_BRig_RT_dataLC_Wrong_Block_l2.vi"() -> ("output_Wrong_Block_l2"=w520:i32)  [unwired: 11 in]
              n379 = call "myRIO_BRig_RT_dataLC_Wrong_Trial_l2.vi"() -> ("output_Wrong_Trial_l2"=w521:i32)  [unwired: 11 in]
              n380 = call "myRIO_BRig_RT_dataLC_Wrong_Probability_l2.vi"() -> ("output_Wrong_Probability_l2"=w522:i32)  [unwired: 11 in]
              n381 = call "myRIO_BRig_RT_dataLC_Selection_OnOff_Switch_l2.vi"() -> ("output_Selection_OnOff_Switch_l2"=w533:i32)  [unwired: 11 in]
              n382 = call "myRIO_BRig_RT_dataLC_Selection_Tdelay_Switch_l2.vi"() -> ("output_Selection_Tdelay_Switch_l2"=w534:i32)  [unwired: 11 in]
              n383 = call "myRIO_BRig_RT_dataLC_Selection_Block_Switch_l2.vi"() -> ("output_Selection_Block_Switch_l2"=w535:i32)  [unwired: 11 in]
              n384 = call "myRIO_BRig_RT_dataLC_Selection_Count_Switch_l2.vi"() -> ("output_Selection_Count_Switch_l2"=w536:i32)  [unwired: 11 in]
              n385 = call "myRIO_BRig_RT_dataLC_Selection_Probability_Switch_l2.vi"() -> ("output_Selection_Probability_Switch_l1"=w537:i32)  [unwired: 11 in]
              n386 = call "myRIO_BRig_RT_dataLC_Selection_OnOff_NS_l2.vi"() -> ("output_Selection_OnOff_NS_l2"=w528:i32)  [unwired: 11 in]
              n387 = call "myRIO_BRig_RT_dataLC_Selection_Tdelay_NS_l2.vi"() -> ("output_Selection_Tdelay_NS_l2"=w529:i32)  [unwired: 11 in]
              n388 = call "myRIO_BRig_RT_dataLC_Selection_Block_NS_l2.vi"() -> ("output_Selection_Block_NS_l2"=w530:i32)  [unwired: 11 in]
              n389 = call "myRIO_BRig_RT_dataLC_Selection_Count_NS_l2.vi"() -> ("output_Selection_Count_NS_l2"=w531:i32)  [unwired: 11 in]
              n390 = call "myRIO_BRig_RT_dataLC_Selection_Probability_NS_l2.vi"() -> ("output_Selection_Probability_NS_l2"=w532:i32)  [unwired: 11 in]
              n391 = Index Array(array=w560, index #1=w523, index #2=w524, index #3=w525, index #4=w526, index #5=w527, index #6=w518, index #7=w519, index #8=w520, index #9=w521, index #10=w522, index #11=w533, index #12=w534, index #13=w535, index #14=w536, index #15=w537, index #16=w528, index #17=w529, index #18=w530, index #19=w531, index #20=w532) -> (element #1=w559:u16, element #2=w558:u16, element #3=w557:u16, element #4=w556:u16, element #5=w555:u16, element #6=w554:u16, element #7=w553:u16, element #8=w552:u16, element #9=w551:u16, element #10=w550:u16, element #11=w547:u16, element #12=w546:u16, element #13=w545:u16, element #14=w544:u16, element #15=w543:u16, element #16=w542:u16, element #17=w541:u16, element #18=w540:u16, element #19=w539:u16, element #20=w538:u16)
              n392 = Not Equal To 0?(x=w559) -> (x != 0?=w562:bool)
              n393 = Not Equal To 0?(x=w554) -> (x != 0?=w561:bool)
              n394 = Not Equal To 0?(x=w547) -> (x != 0?=w549:bool)
              n395 = Not Equal To 0?(x=w542) -> (x != 0?=w548:bool)
              n396 = local write "LC_Reward_OnOff_l2"(w562) -> ()
              n397 = local write "LC_Reward_Tdelay_l2"(w558) -> ()
              n398 = local write "LC_Reward_Block_l2"(w557) -> ()
              n399 = local write "LC_Reward_Trial_l2"(w556) -> ()
              n400 = local write "LC_Reward_Probability_l2"(w555) -> ()
              n401 = local write "LC_Wrong_OnOff_l2"(w561) -> ()
              n402 = local write "LC_Wrong_Tdelay_l2"(w553) -> ()
              n403 = local write "LC_Wrong_Block_l2"(w552) -> ()
              n404 = local write "LC_Wrong_Trial_l2"(w551) -> ()
              n405 = local write "LC_Wrong_Probability_l2"(w550) -> ()
              n406 = local write "LC_Sel_OnOff_Switch_l2"(w549) -> ()
              n407 = local write "LC_Sel_Tdelay_Switch_l2"(w546) -> ()
              n408 = local write "LC_Sel_Block_Switch_l2"(w545) -> ()
              n409 = local write "LC_Sel_Count_Switch_l2"(w544) -> ()
              n410 = local write "LC_Sel_Probability_Switch_l2"(w543) -> ()
              n411 = local write "LC_Sel_OnOff_NS_l2"(w548) -> ()
              n412 = local write "LC_Sel_Tdelay_NS_l2"(w541) -> ()
              n413 = local write "LC_Sel_Block_NS_l2"(w540) -> ()
              n414 = local write "LC_Sel_Count_NS_l2"(w539) -> ()
              n415 = local write "LC_Sel_Probability_NS_l2"(w538) -> ()
            }
            frame "UploadSettings_dataMTrig_1" {
              # "Tdelay_R"
              # "Tdelay_L"
              # "Tcycle_R"
              # "Tcycle_L"
              # "RewCalib_nCycle_R"
              # "RewCalib_nCycle_L"
              # "Solenoid"
              # "Laser_Tcycle"
              n416 = call "myRIO_BRig_RT_dataMTrig_Laser_Tcycle.vi"() -> ("output_Laser_Tcycle"=w572:i32)  [unwired: 11 in]
              n417 = call "myRIO_BRig_RT_dataMTrig_Solenoid_RewCalib_nCycle__L.vi"() -> ("output_Solenoid_RewCalib_nCycle__L"=w571:i32)  [unwired: 11 in]
              n418 = call "myRIO_BRig_RT_dataMTrig_Solenoid_RewCalib_nCycle__R.vi"() -> ("output_Solenoid_RewCalib_nCycle__R"=w570:i32)  [unwired: 11 in]
              n419 = call "myRIO_BRig_RT_dataMTrig_Solenoid_Tdelay__L.vi"() -> ("output_Solenoid_Tdelay__L"=w567:i32)  [unwired: 11 in]
              n420 = call "myRIO_BRig_RT_dataMTrig_Solenoid_Tdelay__R.vi"() -> ("output_Solenoid_Tdelay__R"=w566:i32)  [unwired: 11 in]
              n421 = call "myRIO_BRig_RT_dataMTrig_Solenoid_Tcycle__L.vi"() -> ("output_Solenoid_Tcycle__L"=w569:i32)  [unwired: 11 in]
              n422 = call "myRIO_BRig_RT_dataMTrig_Solenoid_Tcycle__R.vi"() -> ("output_Solenoid_Tcycle__R"=w568:i32)  [unwired: 11 in]
              n423 = Index Array(array=w565, index #1=w572, index #2=w571, index #3=w570, index #4=w569, index #5=w568, index #6=w567, index #7=w566) -> (element #1=w579:u16, element #2=w578:u16, element #3=w577:u16, element #4=w576:u16, element #5=w575:u16, element #6=w574:u16, element #7=w573:u16)
              n424 = Replace Array Subset(array=w581, new element #1=w579, index #1=w572, new element #2=w578, index #2=w571, new element #3=w577, index #3=w570, new element #4=w576, index #4=w569, new element #5=w575, index #5=w568, new element #6=w574, index #6=w567, new element #7=w573, index #7=w566) -> (w580:u16[])
              n425 = local write "MTrig_Solenoid_Tcycle__L"(w576) -> ()
              n426 = local write "MTrig_Solenoid_Tcycle__R"(w575) -> ()
              n427 = local write "MTrig_Laser_Tcycle"(w579) -> ()
            }
            frame "Idle" {
              # "To ensure timing, we split the\nidle state into 4 phases"
              # "Laser_Tcycle"
              # "Audio_Tcycle_R"
              # "Audio_Tcycle_L"
              n428 = local read "Laser_power_min_l1"() -> (w587:dbl)
              n429 = local read "Laser_power_min_l2"() -> (w585:dbl)
              n430 = local read "Audio_Amp__R"() -> (w589:u16)
              n431 = local read "Audio_Amp__L"() -> (w591:u16)
              n432 = local read "Audio_Freq__R"() -> (w588:u8)
              n433 = local read "Audio_Freq__L"() -> (w590:u8)
              n434 = Select(t=myRIO_BRig_RT__Case_NonExp_stateList."SendData" ("Enum"), s="SendData", f=myRIO_BRig_RT__Case_NonExp_stateList."Idle_2" ("Enum")) -> (s? t:f=w596:T1)
              n435 = call "myRIO__convert__Voltage_to_FPGAvalue.vi"("input_voltage"=w587) -> ("output_PortC"=w586:i16)  [unwired: 9 in, 1 out]
              n436 = call "myRIO__convert__Voltage_to_FPGAvalue.vi"("input_voltage"=w585) -> ("output_PortC"=w584:i16)  [unwired: 9 in, 1 out]
              n437 = Select(t=myRIO_BRig_RT__Case_NonExp_stateList."TestConnection" ("Enum"), s="TestConnection", f=w596) -> (s? t:f=w600:T1)
              n438 = xnode "Read/Write Control"("FPGA VI Reference In"=w593, "error in"=w592, "audioAmp_L"=w591, "audioFreq_L_kHz"=w590, "audioAmp_R"=w589, "audioFreq_R_kHz"=w588, "AnaOut_0"=w586, "AnaOut_1"=w584) -> ("error out"=w583:errorcluster)  [unwired: 1 out]
              n439 = local write "error out"(w583) -> ()
              n440 = call "myRIO_BRig_RT_dataMTrig_Audio_Tcycle__L.vi"() -> ("output_Audio_Tcycle__L"=w607:i32)  [unwired: 11 in]
              n441 = call "myRIO_BRig_RT_dataMTrig_Audio_Tcycle__R.vi"() -> ("output_Audio_Tcycle__R"=w606:i32)  [unwired: 11 in]
              n442 = call "myRIO_BRig_RT_dataMTrig_Laser_Tcycle.vi"() -> ("output_Laser_Tcycle"=w605:i32)  [unwired: 11 in]
              n443 = local read "MTrig_Laser_Tcycle"() -> (w594:u16)
              n444 = local read "Tcycle_Cue_min"() -> (w595:u16)
              n445 = Replace Array Subset(array=w603, new element #1=w595, index #1=w607, new element #2=w595, index #2=w606, new element #3=w594, index #3=w605) -> (w604:u16[])
            }
            frame "Idle_2" {
              w609 = u16 0 ("t")
              # "To ensure timing, we split the\nidle state into 4 phases"
              # "Ncycles"
              # "Ncycles"
              # "RewCalib"
              # "RewCalib"
              # "Solenoid R"
              # "Solenoid L"
              n446 = call "myRIO_BRig_RT_dataMTrig_Solenoid_RewCalib_OnOff__L.vi"() -> ("output_Solenoid_RewCalib_OnOff__L"=w639:i32)  [unwired: 11 in]
              n447 = call "myRIO_BRig_RT_dataMTrig_Solenoid_N__L.vi"() -> ("output_Solenoid_N__L"=w627:i32)  [unwired: 11 in]
              n448 = call "myRIO_BRig_RT_dataMTrig_Solenoid_RewCalib_OnOff__R.vi"() -> ("output_Solenoid_RewCalib_OnOff__R"=w624:i32)  [unwired: 11 in]
              n449 = call "myRIO_BRig_RT_dataMTrig_Solenoid_N__R.vi"() -> ("output_Solenoid_N__R"=w623:i32)  [unwired: 11 in]
              n450 = Index Array(array=w630, index #1=w639, index #2=w627, index #3=w624, index #4=w623) -> (element #1=w626:u16, element #2=w621:u16, element #3=w622:u16, element #4=w620:u16)
              n451 = local read "RewCalib_Trig_L"() -> (w619:bool)
              n452 = local read "RewCalib_Trig_R"() -> (w618:bool)
              n453 = Equal To 0?(x=w621) -> (x = 0?=w629:bool)
              n454 = Equal To 0?(x=w620) -> (x = 0?=w628:bool)
              n455 = Not Equal To 0?(x=w622) -> (x != 0?=w640:bool)
              n456 = Not Equal To 0?(x=w626) -> (x != 0?=w641:bool)
              n457 = And(x=w629, y=w628) -> (x .and. y?=w633:bool)
              n458 = Or(x=w619, y=w618) -> (x .or. y?=w634:bool)
              n459 = Not Exclusive Or(1:w641, 2:w619) -> (0:w636:bool)
              n460 = Not Exclusive Or(1:w640, 2:w618) -> (0:w638:bool)
              n461 = And(x=w634, y=w633) -> (x .and. y?=w616:bool)
              n462 = Not(x=w636) -> (.not. x?=w635:bool)
              n463 = Not(x=w638) -> (.not. x?=w637:bool)
              n464 = Or(x=w635, y=w637) -> (x .or. y?=w617:bool)
              n465 = Or(x=w616, y=w617) -> (x .or. y?=w632:bool)
              n466 = local read "count_warmup_R"() -> (w608:u16)
              n467 = local read "count_warmup_L"() -> (w613:u16)
              n468 = Select(t=myRIO_BRig_RT__Case_NonExp_stateList."RewardCalibration_pre" ("Enum"), s=w632, f=myRIO_BRig_RT__Case_NonExp_stateList."Idle_3" ("Enum")) -> (s? t:f=w615:T1)
              n469 = Select(t=w609, s="count_warmup_L_reset", f=w613) -> (s? t:f=→"count_warmup_L":u16)
              n470 = Select(t=w609, s="count_warmup_R_reset", f=w608) -> (s? t:f=→"count_warmup_R":u16)
            }
            frame "Idle_3" {
              n471 = local read "MTrig_Laser_Switch"() -> (w656:bool)
              n472 = case shown="False" w656 {
                tunnel: "LR_reward_Event" -> [w668 w672]
                tunnel: "LR_wrong_Event" -> [w667 w671]
                tunnel: "LR_reward_Laser" -> [w666 w670]
                tunnel: "LR_wrong_Laser" -> [w665 w669]
                tunnel: [w668 _] -> w651
                tunnel: [w667 _] -> w650
                tunnel: [w666 _] -> w649
                tunnel: [w665 _] -> w648
                tunnel: [_ w672] -> w647
                tunnel: [_ w671] -> w646
                tunnel: [_ w670] -> w645
                tunnel: [_ w669] -> w644
                frame False {
                }
                frame True {
                }
              }
              n473 = xnode "Read/Write Control"("FPGA VI Reference In"=w664, "error in"=w663, "Left(F)_or_Right(T)"="Left(F)_or_Right(T)", "SelectionState"="SelectionState", "ignoreWrong"="ignoreWrong", "LR_reward_Event_l1"=w651, "LR_wrong_Event_l1"=w650, "LR_reward_Laser_l1"=w649, "LR_wrong_Laser_l1"=w648, "LR_reward_Event_l2"=w647, "LR_wrong_Event_l2"=w646, "LR_reward_Laser_l2"=w645, "LR_wrong_laser_l2"=w644) -> ("error out"=→"error out 6":errorcluster, "SelectReward"=→"SelectReward":bool, "SelectWrong"=→"SelectWrong":bool)  [unwired: 1 out]
            }
            frame "Idle_4" {
              n474 = local read "Laser_Tshutter_l1"() -> (w692:dbl)
              n475 = local read "Laser_duration_l1"() -> (w691:u16)
              n476 = local read "Laser_Tshutter_l2"() -> (w688:dbl)
              n477 = local read "Laser_duration_l2"() -> (w687:u16)
              n478 = local read "CueLed_duration"() -> (w683:u16)
              n479 = local read "Laser_Tpeak_l1"() -> (w694:dbl)
              n480 = local read "Laser_Tpeak_l2"() -> (w690:dbl)
              n481 = local read "CueLed_Tpeak"() -> (w685:dbl)
              n482 = local read "Laser_Freq_l1"() -> (w693:dbl)
              n483 = local read "Laser_Freq_l2"() -> (w689:dbl)
              n484 = local read "CueLed_Freq"() -> (w684:dbl)
              n485 = local read "FPGA_count2ms"() -> (w686:dbl)
              n486 = To Unsigned Word Integer(number=w686) -> (unsigned 16bit integer=w695:u16)
              n487 = call "myRIO_BRig_RT__calc_laser_FPGA_N.vi"("input_FPGA_count2ms"=w686, "input_Tpeak"=w694, "input_Freq"=w693, "input_Tshutter"=w692, "input_duration"=w691) -> ("output_laser_Npeak"=w682:u32, "output_laser_Nvalley"=w680:u32, "output_laser_Nshutter"=w678:u32, "output_laser_Nduration"=w676:u32)  [unwired: 6 in, 1 out]
              n488 = call "myRIO_BRig_RT__calc_laser_FPGA_N.vi"("input_FPGA_count2ms"=w686, "input_Tpeak"=w690, "input_Freq"=w689, "input_Tshutter"=w688, "input_duration"=w687) -> ("output_laser_Npeak"=w681:u32, "output_laser_Nvalley"=w679:u32, "output_laser_Nshutter"=w677:u32, "output_laser_Nduration"=w675:u32)  [unwired: 6 in, 1 out]
              n489 = call "myRIO_BRig_RT__calc_laser_FPGA_N__CueLed.vi"("input_FPGA_count2ms"=w686, "input_Tpeak"=w685, "input_Freq"=w684, "input_duration"=w683) -> ("output_laser_Npeak"=w674:u32, "output_laser_Nvalley"=w673:u32)  [unwired: 9 in, 1 out]
              n490 = xnode "Read/Write Control"("FPGA VI Reference In"=w700, "error in"=w699, "k1__counter_per_ms"=w695, "LC_nPeak_l1"=w682, "LC_nPeak_l2"=w681, "LC_nValley_l1"=w680, "LC_nValley_l2"=w679, "LC_nShutter_l1"=w678, "LC_nShutter_l2"=w677, "LR_reward_nTotal_l1"=w676, "LR_wrong_nTotal_l1"=w676, "LR_reward_nTotal_l2"=w675, "LR_wrong_nTotal_l2"=w675, "CueLed_nPeak"=w674, "CueLed_nValley"=w673) -> ("error out"=w696:errorcluster)  [unwired: 1 out]
              n491 = local write "error out"(w696) -> ()
            }
            frame "Idle_5" {
              w722 = u8 0 ("f")
              # "To ensure timing, we split the\nidle state into 4 phases"
              n492 = local read "MTrig_Solenoid_trig__L"() -> (w713:bool)
              n493 = local read "MTrig_Solenoid_trig__R"() -> (w723:bool)
              n494 = local read "warmupType"() -> (w706:u8)
              n495 = local read "warmup"() -> (w715:bool)
              n496 = Not Equal To 0?(x=w706) -> (x != 0?=w705:bool)
              n497 = Not(x=w705) -> (.not. x?=w716:bool)
              n498 = Select(t=u8 1, s=w713, f=w722) -> (s? t:f=w721:u8)
              n499 = Select(t=u8 2, s=w723, f=w722) -> (s? t:f=w720:u8)
              n500 = And(x=w715, y=w716) -> (x .and. y?=w714:bool)
              n501 = And(x=w715, y=w705) -> (x .and. y?=w709:bool)
              n502 = Add(x=w721, y=w720) -> (x+y=w719:u8)
              n503 = case shown="3" w719 {
                tunnel: w718 -> [w726 w730 w748 w766]
                tunnel: [w726 w729 w747 w765] -> w717
                tunnel: w714 -> [_ w728 w746 w764]
                tunnel: [_ TRUE TRUE TRUE] -> w711
                frame 0, Default {
                }
                frame 1 {
                  n504 = case shown="True" w728 {
                    tunnel: w730 -> [w739 w744]
                    tunnel: [w738 w743] -> w729
                    frame True {
                      # "Audio_L"
                      # "Solenoid_L"
                      n505 = call "myRIO_BRig_RT_dataMTrig_Solenoid_N__L.vi"() -> ("output_Solenoid_N__L"=w735:i32)  [unwired: 11 in]
                      n506 = call "myRIO_BRig_RT_dataMTrig_Audio_N__L.vi"() -> ("output_Audio_N__L"=w733:i32)  [unwired: 11 in]
                      n507 = Index Array(array=w739, index #1=w735, index #2=w733) -> (element #1=w737:u16, element #2=w736:u16)
                      n508 = Increment(x=w737) -> (x+1=w734:u16)
                      n509 = Increment(x=w736) -> (x+1=w732:u16)
                      n510 = Replace Array Subset(array=w739, new element #1=w734, index #1=w735, new element #2=w732, index #2=w733) -> (w738:u16[])
                    }
                    frame False {
                      # "Solenoid_L"
                      n511 = call "myRIO_BRig_RT_dataMTrig_Solenoid_N__L.vi"() -> ("output_Solenoid_N__L"=w741:i32)  [unwired: 11 in]
                      n512 = Index Array(array=w744, index=w741) -> (element=w742:u16)
                      n513 = Increment(x=w742) -> (x+1=w740:u16)
                      n514 = Replace Array Subset(array=w744, new element=w740, index=w741) -> (w743:u16[])
                    }
                  }
                  n515 = local write "MTrig_Solenoid_trig__L"(FALSE) -> ()
                }
                frame 2 {
                  n516 = case shown="True" w746 {
                    tunnel: w748 -> [w757 w762]
                    tunnel: [w756 w761] -> w747
                    frame True {
                      # "Audio_R"
                      # "Solenoid_R"
                      n517 = call "myRIO_BRig_RT_dataMTrig_Solenoid_N__R.vi"() -> ("output_Solenoid_N__R"=w753:i32)  [unwired: 11 in]
                      n518 = call "myRIO_BRig_RT_dataMTrig_Audio_N__R.vi"() -> ("output_Audio_N__R"=w752:i32)  [unwired: 11 in]
                      n519 = Index Array(array=w757, index #1=w753, index #2=w752) -> (element #1=w755:u16, element #2=w754:u16)
                      n520 = Increment(x=w754) -> (x+1=w750:u16)
                      n521 = Increment(x=w755) -> (x+1=w751:u16)
                      n522 = Replace Array Subset(array=w757, new element #1=w751, index #1=w753, new element #2=w750, index #2=w752) -> (w756:u16[])
                    }
                    frame False {
                      # "Solenoid_R"
                      n523 = call "myRIO_BRig_RT_dataMTrig_Solenoid_N__R.vi"() -> ("output_Solenoid_N__R"=w758:i32)  [unwired: 11 in]
                      n524 = Index Array(array=w762, index=w758) -> (element=w760:u16)
                      n525 = Increment(x=w760) -> (x+1=w759:u16)
                      n526 = Replace Array Subset(array=w762, new element=w759, index=w758) -> (w761:u16[])
                    }
                  }
                  n527 = local write "MTrig_Solenoid_trig__R"(FALSE) -> ()
                }
                frame 3 {
                  w767 = FALSE
                  n528 = case shown="True" w764 {
                    tunnel: w766 -> [w781 w789]
                    tunnel: [w780 w788] -> w765
                    frame True {
                      # "Audio_R"
                      # "Solenoid_R"
                      # "Audio_L"
                      # "Solenoid_L"
                      n529 = call "myRIO_BRig_RT_dataMTrig_Solenoid_N__L.vi"() -> ("output_Solenoid_N__L"=w775:i32)  [unwired: 11 in]
                      n530 = call "myRIO_BRig_RT_dataMTrig_Audio_N__L.vi"() -> ("output_Audio_N__L"=w773:i32)  [unwired: 11 in]
                      n531 = call "myRIO_BRig_RT_dataMTrig_Solenoid_N__R.vi"() -> ("output_Solenoid_N__R"=w771:i32)  [unwired: 11 in]
                      n532 = call "myRIO_BRig_RT_dataMTrig_Audio_N__R.vi"() -> ("output_Audio_N__R"=w770:i32)  [unwired: 11 in]
                      n533 = Index Array(array=w781, index #1=w775, index #2=w773, index #3=w771, index #4=w770) -> (element #1=w779:u16, element #2=w778:u16, element #3=w777:u16, element #4=w776:u16)
                      n534 = Increment(x=w776) -> (x+1=w768:u16)
                      n535 = Increment(x=w779) -> (x+1=w774:u16)
                      n536 = Increment(x=w778) -> (x+1=w772:u16)
                      n537 = Increment(x=w777) -> (x+1=w769:u16)
                      n538 = Replace Array Subset(array=w781, new element #1=w774, index #1=w775, new element #2=w772, index #2=w773, new element #3=w769, index #3=w771, new element #4=w768, index #4=w770) -> (w780:u16[])
                    }
                    frame False {
                      # "Solenoid_R"
                      # "Solenoid_L"
                      n539 = call "myRIO_BRig_RT_dataMTrig_Solenoid_N__L.vi"() -> ("output_Solenoid_N__L"=w785:i32)  [unwired: 11 in]
                      n540 = call "myRIO_BRig_RT_dataMTrig_Solenoid_N__R.vi"() -> ("output_Solenoid_N__R"=w782:i32)  [unwired: 11 in]
                      n541 = Index Array(array=w789, index #1=w785, index #2=w782) -> (element #1=w787:u16, element #2=w786:u16)
                      n542 = Increment(x=w787) -> (x+1=w784:u16)
                      n543 = Increment(x=w786) -> (x+1=w783:u16)
                      n544 = Replace Array Subset(array=w789, new element #1=w784, index #1=w785, new element #2=w783, index #2=w782) -> (w788:u16[])
                    }
                  }
                  n545 = local write "MTrig_Solenoid_trig__L"(w767) -> ()
                  n546 = local write "MTrig_Solenoid_trig__R"(w767) -> ()
                }
              }
              n547 = local read "get_countPerMS"() -> (w704:bool)
              n548 = Select(t=myRIO_BRig_RT__Case_NonExp_stateList."Get_FPGA_count_per_ms" ("Enum"), s=w704, f=myRIO_BRig_RT__Case_NonExp_stateList."Idle_6" ("Enum")) -> (s? t:f=w702:T1)
              n549 = Select(t=myRIO_BRig_RT__Case_NonExp_stateList."Cue_pre", s=w709, f=myRIO_BRig_RT__Case_NonExp_stateList."DispenseWater_pre" ("Enum")) -> (s? t:f=w707:T1)
              n550 = Select(t=w707, s=w711, f=w702) -> (s? t:f=w712:T1)
            }
            frame "Idle_6" {
              # "use dataMTrig as it is one of the last to transfer"
              # "To ensure timing, we split the\nidle state into 4 phases"
              n551 = call "myRIO_BRig_RT_comm_webdav_uploadReceived_check_v2,0.vi"("input_dataName"="dataMTrig") -> ("output_Iexist"=w794:bool)  [unwired: 9 in, 1 out]
              n552 = Select(t=myRIO_BRig_RT__Case_NonExp_stateList."UploadSettings_pre" ("Enum"), s=w794, f=myRIO_BRig_RT__Case_NonExp_stateList."Idle") -> (s? t:f=w792:T1)
            }
            frame "Cue_pre" {
              w813 = u16 1 ("t")
              w812 = u16 0 ("new element/subarray")
              w809 = u16 0 ("new element/subarray")
              # "Ncycle"
              # "count"
              # "Audio_R"
              # "Solenoid_R"
              # "Solenoid_L"
              # "Ncycle"
              # "count"
              # "Audio_L"
              n553 = local read "Cue1Param_CueType_Switch"() -> (w807:u16)
              n554 = case shown="2" w807 {
                tunnel: [TRUE _ w824] -> w804
                frame 0, Default {
                }
                frame 1 {
                }
                frame 2 {
                  n555 = Random Number (0-1)() -> (number: 0 to 1=w830:dbl)
                  n556 = local read "Cue1Param_AudioLed_Probability_Switch"() -> (w825:u16)
                  n557 = Multiply(x=w830, y=100.0) -> (x*y=w829:dbl)
                  n558 = Round To Nearest(number=w829) -> (nearest integer value=w828:dbl)
                  n559 = To Unsigned Word Integer(number=w828) -> (unsigned 16bit integer=w826:u16)
                  n560 = Less?(x=w825, y=w826) -> (x < y?=w824:bool)
                }
              }
              n561 = call "myRIO_BRig_RT_dataMTrig_Solenoid_N__L.vi"() -> ("output_Solenoid_N__L"=w822:i32)  [unwired: 11 in]
              n562 = call "myRIO_BRig_RT_dataMTrig_Solenoid_N__R.vi"() -> ("output_Solenoid_N__R"=w821:i32)  [unwired: 11 in]
              n563 = Index Array(array=w818, index #1=w822, index #2=w821) -> (element #1=w820:u16, element #2=w819:u16)
              n564 = Not Equal To 0?(x=w819) -> (x != 0?=w799:bool)
              n565 = Not Equal To 0?(x=w820) -> (x != 0?=w800:bool)
              n566 = And(x=w804, y=w800) -> (x .and. y?=w805:bool)
              n567 = And(x=w804, y=w799) -> (x .and. y?=w806:bool)
              n568 = Select(t=w813, s=w805, f=w812) -> (s? t:f=w814:u16)
              n569 = Select(t=w813, s=w806, f=w812) -> (s? t:f=w808:u16)
              n570 = Select(t=myRIO_BRig_RT__Case_NonExp_stateList."Cue", s=w804, f=myRIO_BRig_RT__Case_NonExp_stateList."Cue_LED") -> (s? t:f=w802:T1)
              n571 = call "myRIO_BRig_RT_dataMTrig_Audio_c__L.vi"() -> ("output_Audio_c__L"=w816:i32)  [unwired: 11 in]
              n572 = call "myRIO_BRig_RT_dataMTrig_Audio_N__L.vi"() -> ("output_Audio_N__L"=w815:i32)  [unwired: 11 in]
              n573 = call "myRIO_BRig_RT_dataMTrig_Audio_c__R.vi"() -> ("output_Audio_c__R"=w811:i32)  [unwired: 11 in]
              n574 = call "myRIO_BRig_RT_dataMTrig_Audio_N__R.vi"() -> ("output_Audio_N__R"=w810:i32)  [unwired: 11 in]
              n575 = Initialize Array(u16 0 ("element"), 1 ("dimension size")) -> (w798:u16[])
              n576 = Replace Array Subset(array=w818, new element #1=w809, index #1=w816, new element #2=w814, index #2=w815, new element #3=w809, index #3=w811, new element #4=w808, index #4=w810) -> (w817:u16[])
            }
            frame "Cue" {
              # "lick did not occur or warmupType==1"
              # "lick occurred?"
              # "Ncycle"
              # "Audio_R"
              # "Ncycle"
              # "Audio_L"
              n577 = local read "warmupType"() -> (w839:u8)
              n578 = Greater?(x=w845, y=w844) -> (0:w848:bool)
              n579 = Greater?(x=w847, y=w846) -> (0:w843:bool)
              n580 = Or(x=w843, y=w848) -> (x .or. y?=w837:bool)
              n581 = Equal?(x=w839, y=u8 1) -> (x = y?=w833:bool)
              n582 = Not(x=w837) -> (.not. x?=w836:bool)
              n583 = call "myRIO_BRig_RT_dataMTrig_Audio_N__L.vi"() -> ("output_Audio_N__L"=w850:i32)  [unwired: 11 in]
              n584 = call "myRIO_BRig_RT_dataMTrig_Audio_N__R.vi"() -> ("output_Audio_N__R"=w849:i32)  [unwired: 11 in]
              n585 = Or(x=w836, y=w833) -> (x .or. y?=w834:bool)
              n586 = case shown="True" w834 {
                tunnel: w850 -> [w856 w874]
                tunnel: w849 -> [w855 w873]
                tunnel: w842 -> [w858 w868]
                tunnel: [w857 w868] -> w841
                tunnel: w840 -> [_ w866]
                tunnel: [myRIO_BRig_RT__Case_NonExp_stateList."Idle" ("t") w865] -> w835
                tunnel: w833 -> [_ w864]
                tunnel: w832 -> [_ w860]
                tunnel: w831 -> [_ w859]
                frame False {
                  w851 = u16 0 ("new element/subarray")
                  # "lick occurred and warmupType==2"
                  n587 = call "myRIO_BRig_RT_dataMTrig_Solenoid_N__R.vi"() -> ("output_Solenoid_N__R"=w852:i32)  [unwired: 11 in]
                  n588 = call "myRIO_BRig_RT_dataMTrig_Solenoid_N__L.vi"() -> ("output_Solenoid_N__L"=w853:i32)  [unwired: 11 in]
                  n589 = Replace Array Subset(array=w858, new element #1=w851, index #1=w856, new element #2=w851, index #2=w855, new element #3=w851, index #3=w853, new element #4=w851, index #4=w852) -> (w857:u16[])
                }
                frame True {
                  n590 = Not(x=w864) -> (.not. x?=w863:bool)
                  n591 = Index Array(array=w868, index #1=w874, index #2=w873) -> (element #1=w872:u16, element #2=w871:u16)
                  n592 = Equal To 0?(x=w872) -> (x = 0?=w870:bool)
                  n593 = Equal To 0?(x=w871) -> (x = 0?=w869:bool)
                  n594 = And(x=w870, y=w869) -> (x .and. y?=w862:bool)
                  n595 = And(x=w862, y=w863) -> (x .and. y?=w861:bool)
                  n596 = case shown="True" w861 {
                    tunnel: w860 -> [_ w882]
                    tunnel: w859 -> [_ w877]
                    frame False {
                    }
                    frame True {
                      n597 = local read "count_warmup_R"() -> (w875:u16)
                      n598 = local read "count_warmup_L"() -> (w880:u16)
                      n599 = Increment(x=w875) -> (x+1=w878:u16)
                      n600 = Increment(x=w880) -> (x+1=w881:u16)
                      n601 = Select(t=w878, s=w877, f=w875) -> (s? t:f=w876:u16)
                      n602 = Select(t=w881, s=w882, f=w880) -> (s? t:f=w879:u16)
                      n603 = local write "count_warmup_R"(w876) -> ()
                      n604 = local write "count_warmup_L"(w879) -> ()
                    }
                  }
                  n605 = Select(t=myRIO_BRig_RT__Case_NonExp_stateList."DispenseWater_pre", s=w862, f=w866) -> (s? t:f=w865:T1)
                }
              }
            }
            frame "Cue_LED" {
              # "lick did not occur or warmupType==1"
              # "lick occurred?"
              n606 = local read "warmupType"() -> (w895:u8)
              n607 = Greater?(x=w901, y=w900) -> (0:w904:bool)
              n608 = Greater?(x=w903, y=w902) -> (0:w899:bool)
              n609 = Or(x=w899, y=w904) -> (x .or. y?=w893:bool)
              n610 = Equal?(x=w895, y=u8 1) -> (x = y?=w889:bool)
              n611 = Not(x=w893) -> (.not. x?=w892:bool)
              n612 = Or(x=w892, y=w889) -> (x .or. y?=w890:bool)
              n613 = case shown="True" w890 {
                tunnel: w898 -> [w911 w931]
                tunnel: [w910 w931] -> w897
                tunnel: w896 -> [_ w917]
                tunnel: [myRIO_BRig_RT__Case_NonExp_stateList."Idle" ("t") w930] -> w891
                tunnel: w889 -> [_ w916]
                tunnel: w888 -> [_ w928]
                tunnel: w887 -> [_ w927]
                tunnel: w886 -> [w905 w926]
                tunnel: [w905 w919] -> w885
                tunnel: w884 -> [_ w914]
                tunnel: w883 -> [_ w913]
                frame False {
                  w906 = u16 0 ("new element/subarray")
                  # "lick occurred and warmupType==2"
                  n614 = call "myRIO_BRig_RT_dataMTrig_Solenoid_N__R.vi"() -> ("output_Solenoid_N__R"=w907:i32)  [unwired: 11 in]
                  n615 = call "myRIO_BRig_RT_dataMTrig_Solenoid_N__L.vi"() -> ("output_Solenoid_N__L"=w908:i32)  [unwired: 11 in]
                  n616 = Replace Array Subset(array=w911, new element #1=w906, new element #2=w906, index #2=w908, new element #3=w906, index #3=w907) -> (w910:u16[])  [unwired: 1 in]
                }
                frame True {
                  w924 = 0 ("index")
                  n617 = local read "CueLed_duration"() -> (w920:u16)
                  n618 = Index Array(array=w926, index=w924) -> (element=w925:u16)
                  n619 = Increment(x=w925) -> (x+1=w923:u16)
                  n620 = Multiply(x=w923, y=u16 5) -> (x*y=w921:u16)
                  n621 = Replace Array Subset(array=w926, new element=w923, index=w924) -> (w919:u16[])
                  n622 = Less?(x=w921, y=w920) -> (x < y?=w915:bool)
                  n623 = Not Or(1:w916, 2:w915) -> (0:w929:bool)
                  n624 = case shown="True" w929 {
                    tunnel: w928 -> [_ w939]
                    tunnel: w927 -> [_ w934]
                    frame False {
                    }
                    frame True {
                      n625 = local read "count_warmup_R"() -> (w932:u16)
                      n626 = local read "count_warmup_L"() -> (w937:u16)
                      n627 = Increment(x=w932) -> (x+1=w935:u16)
                      n628 = Increment(x=w937) -> (x+1=w938:u16)
                      n629 = Select(t=w935, s=w934, f=w932) -> (s? t:f=w933:u16)
                      n630 = Select(t=w938, s=w939, f=w937) -> (s? t:f=w936:u16)
                      n631 = local write "count_warmup_R"(w933) -> ()
                      n632 = local write "count_warmup_L"(w936) -> ()
                    }
                  }
                  n633 = Select(t=w917, s=w915, f=myRIO_BRig_RT__Case_NonExp_stateList."DispenseWater_pre" ("t")) -> (s? t:f=w930:T1)
                  n634 = xnode "Read/Write Control"("FPGA VI Reference In"=w914, "error in"=w913, "CueLed_Event"=w915) -> ("error out"=w912:errorcluster)  [unwired: 1 out]
                  n635 = local write "error out"(w912) -> ()
                }
              }
            }
            frame "RewardCalibration_pre" {
              (unwired) FALSE
              w940 = FALSE
              w951 = u8 0
              w967 = u8 0
              # "Are we starting a RewardCalibration?\nOr are we stopping a RewardCalibration?\nOr is a RewardCalibration over?"
              # "RewCalib\nOnOff"
              # "N"
              # "Solenoid R"
              # "RewCalib\nOnOff"
              # "N"
              # "Solenoid L"
              n636 = local read "RewCalib_Trig_L"() -> (w974:bool)
              n637 = local read "RewCalib_Trig_R"() -> (w943:bool)
              n638 = call "myRIO_BRig_RT_dataMTrig_Solenoid_N__R.vi"() -> ("output_Solenoid_N__R"=w945:i32)  [unwired: 11 in]
              n639 = call "myRIO_BRig_RT_dataMTrig_Solenoid_RewCalib_OnOff__R.vi"() -> ("output_Solenoid_RewCalib_OnOff__R"=w942:i32)  [unwired: 11 in]
              n640 = call "myRIO_BRig_RT_dataMTrig_Solenoid_N__L.vi"() -> ("output_Solenoid_N__L"=w960:i32)  [unwired: 11 in]
              n641 = call "myRIO_BRig_RT_dataMTrig_Solenoid_RewCalib_OnOff__L.vi"() -> ("output_Solenoid_RewCalib_OnOff__L"=w961:i32)  [unwired: 11 in]
              n642 = Index Array(array=w944, index #1=w945, index #2=w942) -> (element #1=w955:u16, element #2=w950:u16)
              n643 = Index Array(array=w944, index #1=w960, index #2=w961) -> (element #1=w971:u16, element #2=w966:u16)
              n644 = Equal To 0?(x=w955) -> (x = 0?=w956:bool)
              n645 = Not Equal To 0?(x=w950) -> (x != 0?=w953:bool)
              n646 = Equal To 0?(x=w971) -> (x = 0?=w972:bool)
              n647 = Not Equal To 0?(x=w966) -> (x != 0?=w969:bool)
              n648 = local write "MTrig_Solenoid_trig__L"(w940) -> ()
              n649 = local write "MTrig_Solenoid_trig__R"(w940) -> ()
              n650 = Select(t=u8 1, s=w943, f=w951) -> (s? t:f=w947:u8)
              n651 = Select(t=u8 1, s=w974, f=w967) -> (s? t:f=w963:u8)
              n652 = Select(t=u8 2, s=w956, f=w951) -> (s? t:f=w948:u8)
              n653 = Select(t=u8 4, s=w953, f=w951) -> (s? t:f=w949:u8)
              n654 = Select(t=u8 2, s=w972, f=w967) -> (s? t:f=w964:u8)
              n655 = Select(t=u8 4, s=w969, f=w967) -> (s? t:f=w965:u8)
              n656 = Compound Arithmetic op=ADD(w947, w948, w949) -> (w946:u8)
              n657 = Compound Arithmetic op=ADD(w963, w964, w965) -> (w962:u8)
              n658 = case shown="7" w962 {
                tunnel: w944 -> [w1004 w1009 w1011 w1016 w1021 w1023 w1026 w1031]
                tunnel: [w1004 w1010 w1011 w1017 w1022 w1023 w1027 w1032] -> w959
                tunnel: w961 -> [_ w1007 _ w1014 w1019 _ w1025 w1030]
                tunnel: w960 -> [_ w1008 _ w1015 w1020 _ _ _]
                frame 0, Default {
                }
                frame 1 {
                  n659 = Replace Array Subset(array=w1009, new element #1=u16 100 ("new element/subarray"), index #1=w1008, new element #2=u16 1 ("new element/subarray"), index #2=w1007) -> (w1010:u16[])
                }
                frame 2 {
                }
                frame 3 {
                  n660 = Replace Array Subset(array=w1016, new element #1=u16 100 ("new element/subarray"), index #1=w1015, new element #2=u16 1 ("new element/subarray"), index #2=w1014) -> (w1017:u16[])
                }
                frame 4 {
                  w1018 = u16 0 ("new element/subarray")
                  n661 = Replace Array Subset(array=w1021, new element #1=w1018, index #1=w1020, new element #2=w1018, index #2=w1019) -> (w1022:u16[])
                }
                frame 5 {
                }
                frame 6 {
                  n662 = Replace Array Subset(array=w1026, new element=u16 0 ("new element/subarray"), index=w1025) -> (w1027:u16[])
                }
                frame 7 {
                  n663 = local write "RewCalib_Trig_L"(FALSE ("RewCalib_Trig_L")) -> ()
                  n664 = Replace Array Subset(array=w1031, new element=u16 0 ("new element/subarray"), index=w1030) -> (w1032:u16[])
                }
              }
              n665 = case shown="7" w946 {
                tunnel: w959 -> [w975 w980 w982 w987 w992 w994 w997 w1002]
                tunnel: [w975 w981 w982 w988 w993 w994 w998 w1003] -> w958
                tunnel: w942 -> [_ w978 _ w985 w990 _ w996 w1001]
                tunnel: w945 -> [_ w979 _ w986 w991 _ _ _]
                frame 0, Default {
                }
                frame 1 {
                  n666 = Replace Array Subset(array=w980, new element #1=u16 100 ("new element/subarray"), index #1=w979, new element #2=u16 1 ("new element/subarray"), index #2=w978) -> (w981:u16[])
                }
                frame 2 {
                }
                frame 3 {
                  n667 = Replace Array Subset(array=w987, new element #1=u16 100 ("new element/subarray"), index #1=w986, new element #2=u16 1 ("new element/subarray"), index #2=w985) -> (w988:u16[])
                }
                frame 4 {
                  w989 = u16 0 ("new element/subarray")
                  n668 = Replace Array Subset(array=w992, new element #1=w989, index #1=w991, new element #2=w989, index #2=w990) -> (w993:u16[])
                }
                frame 5 {
                }
                frame 6 {
                  n669 = Replace Array Subset(array=w997, new element=u16 0 ("new element/subarray"), index=w996) -> (w998:u16[])
                }
                frame 7 {
                  n670 = local write "RewCalib_Trig_R"(FALSE ("RewCalib_Trig_L")) -> ()
                  n671 = Replace Array Subset(array=w1002, new element=u16 0 ("new element/subarray"), index=w1001) -> (w1003:u16[])
                }
              }
            }
            frame "DispenseWater_pre" {
              w1038 = u16 0 ("t")
              w1081 = u16 0 ("new element/subarray")
              # "just trust me on this one"
              # "RewCalib\nOnOff"
              # "RewCalib\nOnOff"
              # "nCycle"
              # "Solenoid__R"
              # "Tdelay"
              # "delay"
              # "nCycle"
              # "Solenoid__L"
              # "Tdelay"
              # "delay"
              # "Solenoid__R"
              # "count"
              # "Solenoid_Tcycle_R"
              # "Solenoid_Tcycle_L"
              # "Solenoid__L"
              # "count"
              n672 = call "myRIO_BRig_RT_dataMTrig_Solenoid_RewCalib_OnOff__L.vi"() -> ("output_Solenoid_RewCalib_OnOff__L"=w1045:i32)  [unwired: 11 in]
              n673 = call "myRIO_BRig_RT_dataMTrig_Solenoid_N__L.vi"() -> ("output_Solenoid_N__L"=w1036:i32)  [unwired: 11 in]
              n674 = call "myRIO_BRig_RT_dataMTrig_Solenoid_delay__L.vi"() -> ("output_Solenoid_delay__L"=w1079:i32)  [unwired: 11 in]
              n675 = call "myRIO_BRig_RT_dataMTrig_Solenoid_Tdelay__L.vi"() -> ("output_Solenoid_Tdelay__L"=w1078:i32)  [unwired: 11 in]
              n676 = call "myRIO_BRig_RT_dataMTrig_Solenoid_N__R.vi"() -> ("output_Solenoid_N__R"=w1034:i32)  [unwired: 11 in]
              n677 = call "myRIO_BRig_RT_dataMTrig_Solenoid_delay__R.vi"() -> ("output_Solenoid_delay__R"=w1068:i32)  [unwired: 11 in]
              n678 = call "myRIO_BRig_RT_dataMTrig_Solenoid_Tdelay__R.vi"() -> ("output_Solenoid_Tdelay__R"=w1067:i32)  [unwired: 11 in]
              n679 = call "myRIO_BRig_RT_dataMTrig_Solenoid_RewCalib_OnOff__R.vi"() -> ("output_Solenoid_RewCalib_OnOff__R"=w1041:i32)  [unwired: 11 in]
              n680 = Index Array(array=w1080, index #1=w1036, index #2=w1079, index #3=w1078, index #4=w1034, index #5=w1068, index #6=w1067, index #7=w1045, index #8=w1041) -> (element #1=w1037:u16, element #2=w1077:u16, element #3=w1072:u16, element #4=w1040:u16, element #5=w1062:u16, element #6=w1061:u16, element #7=w1046:u16, element #8=w1043:u16)
              n681 = Equal To 0?(x=w1077) -> (x = 0?=w1076:bool)
              n682 = Equal To 0?(x=w1062) -> (x = 0?=w1066:bool)
              n683 = local read "RewCalib_Trig_L"() -> (w1057:bool)
              n684 = local read "RewCalib_Trig_R"() -> (w1052:bool)
              n685 = Not Equal To 0?(x=w1037) -> (x != 0?=w1075:bool)
              n686 = Not Equal To 0?(x=w1040) -> (x != 0?=w1065:bool)
              n687 = local read "MTrig_Solenoid_Tcycle__L"() -> (w1074:u16)
              n688 = local read "MTrig_Solenoid_Tcycle__R"() -> (w1060:u16)
              n689 = Not Equal To 0?(x=w1046) -> (x != 0?=w1056:bool)
              n690 = Not Equal To 0?(x=w1043) -> (x != 0?=w1054:bool)
              n691 = Not(x=w1057) -> (.not. x?=w1055:bool)
              n692 = Not(x=w1052) -> (.not. x?=w1053:bool)
              n693 = And(x=w1056, y=w1055) -> (x .and. y?=w1051:bool)
              n694 = And(x=w1054, y=w1053) -> (x .and. y?=w1050:bool)
              n695 = call "myRIO_BRig_RT_dataMTrig_Solenoid_c__L.vi"() -> ("output_Solenoid_c__L"=w1083:i32)  [unwired: 11 in]
              n696 = call "myRIO_BRig_RT_dataMTrig_Solenoid_c__R.vi"() -> ("output_Solenoid_c__R"=w1082:i32)  [unwired: 11 in]
              n697 = Select(t=w1074, s=w1075, f=u16 0) -> (s? t:f=w1071:u16)
              n698 = Or(x=w1051, y=w1050) -> (x .or. y?=w1039:bool)
              n699 = Select(t=w1060, s=w1065, f=u16 0) -> (s? t:f=w1063:u16)
              n700 = Select(t=w1071, s=w1076, f=w1072) -> (s? t:f=w1069:u16)
              n701 = Select(t=w1063, s=w1066, f=w1061) -> (s? t:f=w1058:u16)
              n702 = call "myRIO_BRig_RT_dataMTrig_Solenoid_Tcycle__L.vi"() -> ("output_Solenoid_Tcycle__L"=w1070:i32)  [unwired: 11 in]
              n703 = call "myRIO_BRig_RT_dataMTrig_Solenoid_Tcycle__R.vi"() -> ("output_Solenoid_Tcycle__R"=w1059:i32)  [unwired: 11 in]
              n704 = Select(t=w1038, s=w1039, f=w1037) -> (s? t:f=w1035:u16)
              n705 = Select(t=w1038, s=w1039, f=w1040) -> (s? t:f=w1033:u16)
              n706 = Select(t=myRIO_BRig_RT__Case_NonExp_stateList."Idle" ("Enum"), s=w1039, f=myRIO_BRig_RT__Case_NonExp_stateList."DispenseWater" ("Enum")) -> (s? t:f=w1047:T1)
              n707 = Select(t=w1038, s=w1039, f=w1046) -> (s? t:f=w1044:u16)
              n708 = Select(t=w1038, s=w1039, f=w1043) -> (s? t:f=w1042:u16)
              n709 = Replace Array Subset(array=w1080, new element #1=w1081, index #1=w1083, new element #2=w1081, index #2=w1082, new element #3=w1069, index #3=w1070, new element #4=w1058, index #4=w1059, new element #5=w1044, index #5=w1045, new element #6=w1042, index #6=w1041, new element #7=w1035, index #7=w1036, new element #8=w1033, index #8=w1034) -> (w1084:u16[])
            }
            frame "DispenseWater" {
              # "D"
              # "C"
              # "B"
              # "A"
              # "(A) Add COUNT and INCREMENT\n(B) Is (A) smaller than Tcycle?\n(C) Are we dispensing water or in the delay phase?\n(D) If (A) is smaller than Tcycle   AND   if we are dispensing water\n      then send TRUE to solenoid"
              # "delay"
              # "Tcycle"
              # "Solenoid__R"
              # "count"
              # "delay"
              # "Tcycle"
              # "Solenoid__L"
              # "count"
              n710 = To Unsigned Word Integer(number=w1111) -> (unsigned 16bit integer=w1093:u16)
              n711 = call "myRIO_BRig_RT_dataMTrig_Solenoid_delay__R.vi"() -> ("output_Solenoid_delay__R"=w1097:i32)  [unwired: 11 in]
              n712 = call "myRIO_BRig_RT_dataMTrig_Solenoid_c__R.vi"() -> ("output_Solenoid_c__R"=w1096:i32)  [unwired: 11 in]
              n713 = call "myRIO_BRig_RT_dataMTrig_Solenoid_Tcycle__R.vi"() -> ("output_Solenoid_Tcycle__R"=w1098:i32)  [unwired: 11 in]
              n714 = call "myRIO_BRig_RT_dataMTrig_Solenoid_delay__L.vi"() -> ("output_Solenoid_delay__L"=w1113:i32)  [unwired: 11 in]
              n715 = call "myRIO_BRig_RT_dataMTrig_Solenoid_c__L.vi"() -> ("output_Solenoid_c__L"=w1105:i32)  [unwired: 11 in]
              n716 = call "myRIO_BRig_RT_dataMTrig_Solenoid_Tcycle__L.vi"() -> ("output_Solenoid_Tcycle__L"=w1114:i32)  [unwired: 11 in]
              n717 = Index Array(array=w1107, index #1=w1105, index #2=w1114, index #3=w1113, index #4=w1096, index #5=w1098, index #6=w1097) -> (element #1=w1112:u16, element #2=w1102:u16, element #3=w1110:u16, element #4=w1092:u16, element #5=w1089:u16, element #6=w1088:u16)
              n718 = Add(x=w1112, y=w1093) -> (x+y=w1103:u16)
              n719 = Add(x=w1092, y=w1093) -> (x+y=w1094:u16)
              n720 = Less?(x=w1103, y=w1102) -> (x < y?=w1086:bool)
              n721 = Equal To 0?(x=w1110) -> (x = 0?=w1109:bool)
              n722 = Less?(x=w1094, y=w1089) -> (x < y?=w1087:bool)
              n723 = Equal To 0?(x=w1088) -> (x = 0?=w1095:bool)
              n724 = And(x=w1086, y=w1109) -> (x .and. y?=w1108:bool)
              n725 = Or(x=w1086, y=w1087) -> (x .or. y?=w1085:bool)
              n726 = And(x=w1087, y=w1095) -> (x .and. y?=w1090:bool)
              n727 = Select(t=w1103, s=w1086, f=w1102) -> (s? t:f=w1104:u16)
              n728 = Select(t=w1094, s=w1087, f=w1089) -> (s? t:f=w1091:u16)
              n729 = Replace Array Subset(array=w1107, new element #1=w1104, index #1=w1105, new element #2=w1091, index #2=w1096) -> (w1106:u16[])
              n730 = Select(t=w1101, s=w1085, f=myRIO_BRig_RT__Case_NonExp_stateList."DispenseWater_post" ("Enum")) -> (s? t:f=w1099:T1)
            }
            frame "DispenseWater_post" {
              # "nCycle"
              # "delay"
              # "Solenoid__R"
              # "nCycle"
              # "delay"
              # "Solenoid__L"
              n731 = call "myRIO_BRig_RT_dataMTrig_Solenoid_N__L.vi"() -> ("output_Solenoid_N__L"=w1131:i32)  [unwired: 11 in]
              n732 = call "myRIO_BRig_RT_dataMTrig_Solenoid_delay__L.vi"() -> ("output_Solenoid_delay__L"=w1130:i32)  [unwired: 11 in]
              n733 = call "myRIO_BRig_RT_dataMTrig_Solenoid_N__R.vi"() -> ("output_Solenoid_N__R"=w1127:i32)  [unwired: 11 in]
              n734 = call "myRIO_BRig_RT_dataMTrig_Solenoid_delay__R.vi"() -> ("output_Solenoid_delay__R"=w1126:i32)  [unwired: 11 in]
              n735 = Index Array(array=w1133, index #1=w1131, index #2=w1130, index #3=w1127, index #4=w1126) -> (element #1=w1135:u16, element #2=w1134:u16, element #3=w1118:u16, element #4=w1120:u16)
              n736 = Not Equal To 0?(x=w1135) -> (x != 0?=w1136:bool)
              n737 = Not Equal To 0?(x=w1118) -> (x != 0?=w1119:bool)
              n738 = case shown="True" w1119 {
                selector: w1119 -> [_ w1140]
                tunnel: w1118 -> [w1138 w1146]
                tunnel: w1120 -> [_ w1147]
                tunnel: [w1138 w1144] -> w1117
                tunnel: [u16 0 w1143] -> w1116
                tunnel: [_ w1140] -> w1115
                frame False {
                }
                frame True {
                  n739 = Equal To 0?(x=w1147) -> (x = 0?=w1139:bool)
                  n740 = Decrement(x=w1146) -> (x-1=w1145:u16)
                  n741 = Select(t=w1145, s=w1139, f=w1146) -> (s? t:f=w1144:u16)
                  n742 = Select(t=u16 1, s=w1139, f=u16 0) -> (s? t:f=w1143:u16)
                }
              }
              n743 = case shown="True" w1136 {
                selector: w1136 -> [_ w1151]
                tunnel: w1135 -> [w1149 w1157]
                tunnel: w1134 -> [_ w1158]
                tunnel: [w1149 w1155] -> w1129
                tunnel: [u16 0 w1154] -> w1128
                tunnel: [_ w1151] -> w1125
                frame False {
                }
                frame True {
                  n744 = Equal To 0?(x=w1158) -> (x = 0?=w1150:bool)
                  n745 = Decrement(x=w1157) -> (x-1=w1156:u16)
                  n746 = Select(t=w1156, s=w1150, f=w1157) -> (s? t:f=w1155:u16)
                  n747 = Select(t=u16 1, s=w1150, f=u16 0) -> (s? t:f=w1154:u16)
                }
              }
              n748 = Or(x=w1125, y=w1115) -> (x .or. y?=w1124:bool)
              n749 = Replace Array Subset(array=w1133, new element #1=w1129, index #1=w1131, new element #2=w1128, index #2=w1130, new element #3=w1117, index #3=w1127, new element #4=w1116, index #4=w1126) -> (w1132:u16[])
              n750 = Select(t=myRIO_BRig_RT__Case_NonExp_stateList."DispenseWater_pre" ("Enum"), s=w1124, f=myRIO_BRig_RT__Case_NonExp_stateList."Idle" ("Enum")) -> (s? t:f=w1121:T1)
            }
            frame "TestConnection" {
              n751 = local read "Host Password"() -> (w1164:string)
              n752 = local read "Host UserName"() -> (w1165:string)
              n753 = call "myRIO_BRig_RT_comm_webdav_testConnect.vi"("input_password"=w1164, "input_username"=w1165) -> ("output_Iconnected"=w1162:bool)  [unwired: 9 in]
              n754 = Select(t="Connection accepted!" ("message"), s=w1162, f="Error!") -> (s? t:f=w1160:string)
              n755 = One Button Dialog(message=w1160) -> ()  [unwired: 1 in, 1 out]
            }
            frame "SendData" {
              n756 = local read "Data Set Prefix"() -> (w1167:string)
              n757 = local read "Host Password"() -> (w1168:string)
              n758 = local read "Host UserName"() -> (w1169:string)
              n759 = call "myRIO_BRig_RT_comm_webdav_sendData_all.vi"("Host Filename Prefix"=w1167, "Host Password"=w1168, "Host UserName"=w1169) -> ()  [unwired: 9 in]
            }
            frame "Get_FPGA_count_per_ms" {
              n760 = case shown="False" w1182 {
                selector: w1182 -> [w1184 _]
                tunnel: w1180 -> [_ w1197]
                tunnel: [w1188 w1197] -> w1179
                tunnel: w1178 -> [w1187 w1195]
                tunnel: w1177 -> [w1186 w1194]
                tunnel: [w1185 w1192] -> w1176
                tunnel: [w1184 w1191] -> w1175
                frame False {
                  n761 = Get Date/Time In Seconds() -> (seconds since 1Jan1904=w1189:timestamp)
                  n762 = xnode "Read/Write Control"("FPGA VI Reference In"=w1187, "error in"=w1186, "timeTrial_trig"=TRUE ("timeTrial")) -> ("error out"=w1185:errorcluster)  [unwired: 1 out]
                  n763 = To Double Precision Float(number=w1189) -> (double precision float=w1188:dbl)
                  n764 = local write "get_countPerMS"(w1184) -> ()
                }
                frame True {
                  w1193 = 1.0
                  n765 = Get Date/Time In Seconds() -> (seconds since 1Jan1904=w1198:timestamp)
                  n766 = To Double Precision Float(number=w1198) -> (double precision float=w1199:dbl)
                  n767 = Subtract(x=w1199, y=w1197) -> (x-y=w1196:dbl)
                  n768 = Less Or Equal?(x=w1193, y=w1196) -> (x <= y?=w1191:bool)
                  n769 = case shown="True" w1191 {
                    tunnel: w1195 -> [_ w1212]
                    tunnel: w1194 -> [w1200 w1211]
                    tunnel: w1193 -> [_ w1202]
                    tunnel: [w1200 w1201] -> w1192
                    frame False {
                    }
                    frame True {
                      n770 = xnode "Read/Write Control"("FPGA VI Reference In"=w1212, "error in"=w1211) -> ("FPGA VI Reference Out"=w1209:refnum<k20>, "error out"=w1208:errorcluster, "timeTrial_count"=w1203:u32)
                      n771 = Multiply(x=w1202, y=1000.0) -> (x*y=w1206:dbl)
                      n772 = To Double Precision Float(number=w1203) -> (double precision float=w1205:dbl)
                      n773 = Divide(x=w1205, y=w1206) -> (x/y=w1207:dbl)
                      n774 = local write "FPGA_count2ms"(w1207) -> ()
                      n775 = xnode "Read/Write Control"("FPGA VI Reference In"=w1209, "error in"=w1208, "timeTrial_trig"=FALSE ("timeTrial")) -> ("error out"=w1201:errorcluster)  [unwired: 1 out]
                    }
                  }
                }
              }
              "error out 5" <- w1176
              n776 = Select(t=myRIO_BRig_RT__Case_NonExp_stateList."Idle" ("Enum"), s=w1175, f=w1173) -> (s? t:f=w1172:T1)
            }
            frame "End" {
            }
          }
          n777 = local read "MTrig_Audio_trig__R"() -> (w89:bool)
          n778 = local read "MTrig_Audio_trig__L"() -> (w90:bool)
          n779 = local read "MTrig_Laser_trig"() -> (w88:bool)
          n780 = Compound Arithmetic op=OR(w90, w89, w88) -> (w87:bool)
          n781 = local read "START"() -> (w113:bool)
          n782 = local read "STOP_abort"() -> (w112:bool)
          n783 = case shown="True" w87 {
            frame False {
            }
            frame True {
              w129 = FALSE
              n784 = local write "MTrig_Audio_trig__R"(w129) -> ()
              n785 = local write "MTrig_Audio_trig__L"(w129) -> ()
              n786 = local write "MTrig_Laser_trig"(w129) -> ()
            }
          }
          n787 = call "myRIO_BRig_RT_dataMTrig_main__v2.vi"("input_dataMTrig"=w116, "input_Audio_trig_L"=w90, "input_Audio_trig_R"=w89, "input_Laser_trig"=w88) -> ("output_dataMTrig"=w115:u16[], "output_Audio_L"=w107:bool, "output_Audio_R"=w108:bool, "output_Laser"=w86:bool)  [unwired: 12 in]
          n788 = Or(x=w113, y=w112) -> (x .or. y?=w111:bool)
          n789 = Select(t=myRIO_BRig_RT__Case_NonExp_stateList."End" ("Enum"), s=w111, f=w110) -> (s? t:f=w109:T1)
          n790 = Not(x="MTrig_Laser_Switch") -> (.not. x?=w83:bool)
          n791 = And(x=w86, y=w83) -> (x .and. y?=w84:bool)
          n792 = And(x=w86, y="MTrig_Laser_Switch") -> (x .and. y?=w85:bool)
          n793 = xnode "Read/Write Control"("FPGA VI Reference In"=w96, "error in"=w95, "A1_SR"=w117, "A3_SL"=w118, "audioTrigger_L"=w107, "audioTrigger_R"=w108, "LC_Laser_l1"=w84, "LC_Laser_l2"=w85) -> ("FPGA VI Reference Out"=w123:refnum<k20>, "error out"=w122:errorcluster)
          n794 = node-c288() -> ()  [unwired: 1 in, 1 out]
          "cState_NonExp" <- w121
        }
        n795 = node-c288(w70) -> ()  [unwired: 1 out]
        n796 = flat-sequence {
          tunnel: w63 -> [w81]
          tunnel: [w81] -> w62
          tunnel: w61 -> [w80]
          tunnel: [w80] -> w60
          frame #0 {
            w79 = FALSE
            n797 = local write "STOP_endBlock"(w79) -> ()
            n798 = local write "STOP_endTrial"(w79) -> ()
          }
        }
      }
      frame True {
        w1224 = u16 0
        w1243 = u8 0
        w1244 = u16 0 ("idxDataBlock")
        w1246 = u16 100 ("new element/subarray")
        w1247 = u16 100 ("new element/subarray")
        w1267 = T6 refnum items=["Session NI_WebDAV"] ("output_hSession")
        w1276 = FALSE
        w1277 = u16 0
        w1231 = FALSE
        # "dummyState counter"
        # "audio__L\naudio__R"
        # "Audio params"
        # "nRewards"
        # "idxDataBlock"
        # "Solenoid_Tdelay_R"
        # "Solenoid_Tdelay_L"
        # "RewCalib_N__R"
        # "RewCalib_N__L"
        # "Save dataLick to file\nSend file to Host\nSave dataMTrig\nSend file to Host\nDisconnect"
        # "dataTrial"
        # "dataTrial"
        # "Solenoid_Tcycle_R"
        # "Solenoid_Tcycle_L"
        # "Laser_Tcycle"
        # "Audio_Tcycle_R"
        # "Audio_Tcycle_L"
        # "dataLick"
        # "dataLC"
        # "dataLC"
        # "dataBlock"
        # "dataBlock"
        # "dataMTrig"
        # "dataMTrig"
        # "dataExp"
        # "dataCurrent"
        # "dataExp"
        # "dataCurrent"
        # "spout"
        # "state"
        n799 = call "myRIO_BRig_RT_dataMTrig_Solenoid_Tcycle__L.vi"() -> ("output_Solenoid_Tcycle__L"=w1273:i32)  [unwired: 11 in]
        n800 = call "myRIO_BRig_RT_dataMTrig_Solenoid_Tcycle__R.vi"() -> ("output_Solenoid_Tcycle__R"=w1272:i32)  [unwired: 11 in]
        n801 = call "myRIO_BRig_RT_dataMTrig_Audio_Tcycle__L.vi"() -> ("output_Audio_Tcycle__L"=w1271:i32)  [unwired: 11 in]
        n802 = call "myRIO_BRig_RT_dataMTrig_Audio_Tcycle__R.vi"() -> ("output_Audio_Tcycle__R"=w1270:i32)  [unwired: 11 in]
        n803 = call "myRIO_BRig_RT_dataMTrig_Laser_Tcycle.vi"() -> ("output_Laser_Tcycle"=w1269:i32)  [unwired: 11 in]
        n804 = local read "MTrig_Solenoid_Tcycle__L"() -> (w1252:u16)
        n805 = local read "MTrig_Solenoid_Tcycle__R"() -> (w1251:u16)
        n806 = local read "Tcycle_Reward_L"() -> (w1248:u16)
        n807 = local read "Tcycle_Reward_R"() -> (w1249:u16)
        n808 = local read "MTrig_Laser_Tcycle"() -> (w1250:u16)
        n809 = call "myRIO_BRig_RT_dataMTrig_Solenoid_RewCalib_nCycle__L.vi"() -> ("output_Solenoid_RewCalib_nCycle__L"=w1255:i32)  [unwired: 11 in]
        n810 = call "myRIO_BRig_RT_dataMTrig_Solenoid_Tdelay__L.vi"() -> ("output_Solenoid_Tdelay__L"=w1257:i32)  [unwired: 11 in]
        n811 = call "myRIO_BRig_RT_dataMTrig_Solenoid_RewCalib_nCycle__R.vi"() -> ("output_Solenoid_RewCalib_nCycle__R"=w1256:i32)  [unwired: 11 in]
        n812 = call "myRIO_BRig_RT_dataMTrig_Solenoid_Tdelay__R.vi"() -> ("output_Solenoid_Tdelay__R"=w1258:i32)  [unwired: 11 in]
        n813 = case shown="False" w1235 {
          selector: w1235 -> [_ w1299]
          tunnel: w1234 -> [w1296 w1301]
          tunnel: [w1297 w1301] -> w1229
          tunnel: w1233 -> [_ w1300]
          tunnel: [w1298 w1300] -> w1230
          tunnel: [w1295 w1299] -> w1228
          frame False {
            n814 = call "myRIO__TCP_connect_forWriting.vi"("input_error"=w1296) -> ("output_error"=w1297:errorcluster, "output_connected"=w1295:bool, "output_hTCP"=w1298:refnum<k5>)  [unwired: 8 in]
          }
          frame True {
          }
        }
        n815 = call "myRIO_BRig_RT_dataLick_init.vi"() -> ("output_dataLick"=w1279:u16[][])  [unwired: 11 in]
        n816 = call "myRIO_BRig_RT_dataCurrent_init.vi"() -> ("output_dataCurrent"=w1286:u16[])  [unwired: 11 in]
        n817 = call "myRIO_BRig_RT_dataExp_init.vi"() -> ("output_dataExp"=w1285:u16[])  [unwired: 11 in]
        n818 = call "myRIO_BRig_RT_dataMTrig_init.vi"() -> ("output_dataMTrig"=w1275:u16[])  [unwired: 5 in]
        n819 = call "myRIO_BRig_RT_dataLC_init.vi"() -> ("output_dataLC"=w1283:u16[])  [unwired: 11 in]
        n820 = call "myRIO_BRig_RT_dataBlock_init.vi"() -> ("output_dataBlock"=w1284:u16[][])  [unwired: 11 in]
        n821 = call "myRIO_BRig_RT_dataTrial_init.vi"() -> ("output_dataTrial"=w1268:u16[][])  [unwired: 11 in]
        n822 = local write "I_connect_TCP"(w1228) -> ()
        n823 = Replace Array Subset(array=w1275, new element #1=w1247, index #1=w1255, new element #2=w1247, index #2=w1256, new element #3=w1246, index #3=w1257, new element #4=w1246, index #4=w1258, new element #5=w1252, index #5=w1273, new element #6=w1251, index #6=w1272, new element #7=w1248, index #7=w1271, new element #8=w1249, index #8=w1270, new element #9=w1250, index #9=w1269) -> (w1274:u16[])
        n824 = call "myRIO_BRig_RT_dataAnalog_init.vi"() -> ("output_dataAnalog"=w1240:u16[][])  [unwired: 11 in]
        n825 = call "myRIO_BRig_RT_TCP__start_exp.vi"("input_hTCP"=w1230, "input_I_connected_TCP"=w1228, "input_error"=w1229) -> ("output_hTCP"=w1227:refnum<k5>, "output_error"=w1226:errorcluster)  [unwired: 11 in]
        n826 = Get Date/Time In Seconds() -> (seconds since 1Jan1904=w1254:timestamp)
        n827 = call "myRIO_BRig_RT_arrTrig_init.vi"() -> ("output_arrTrig"=w1223:bool[])  [unwired: 11 in]
        n828 = To Double Precision Float(number=w1254) -> (double precision float=w1253:dbl)
        n829 = node-c288() -> (w1294:T3)  [unwired: 4 in]
        n830 = timed-loop {
          timing: w1294 -> [_]
          timing-out: [_] -> w1293
          shift-right: [w1423] -> _
          shift-left: myRIO_BRig_RT__Case_Exp_stateList."Start1" ("Enum") -> [w1371]
          shift-right: [w1368] -> _
          shift-left: enum16{"Left", "Right"}."Left" -> [w1472]
          tunnel: w1222 -> [w1470]
          tunnel: w1221 -> [w1469]
          shift-right: [w1464] -> _
          shift-left: w1291 -> [w1468]
          shift-right: [w1463] -> _
          shift-left: w1290 -> [w1467]
          tunnel: [w1446] -> w1288
          tunnel: [w1447] -> w1289
          shift-right: [w1448] -> w1259
          shift-left: w1286 -> [w1415]
          shift-right: [w1462] -> _
          shift-left: w1285 -> [w1413]
          shift-right: [w1435] -> w1263
          shift-left: w1274 -> [w1436]
          shift-right: [w1460] -> _
          shift-left: w1284 -> [w1461]
          shift-right: [w1458] -> _
          shift-left: w1283 -> [w1459]
          shift-right: [w1450] -> w1265
          shift-left: w1279 -> [w1451]
          shift-right: [w1437] -> _
          shift-left: w1277 -> [w1445]
          shift-right: [w1410] -> _
          shift-left: w1243 -> [w1444]
          shift-right: [w1438] -> _
          shift-left: w1277 -> [w1443]
          shift-right: [w1439] -> _
          shift-left: w1243 -> [w1442]
          shift-right: [w1411] -> _
          shift-left: w1276 -> [w1440]
          shift-right: [w1412] -> _
          shift-left: w1276 -> [w1441]
          shift-right: [w1421] -> _
          shift-left: w1268 -> [w1422]
          shift-right: [w1420] -> w1261
          shift-left: w1267 -> [w1418]
          shift-right: [w1419] -> w1262
          shift-left: FALSE ("output_Iconnected") -> [w1417]
          tunnel: "Data Set Prefix" -> [w1416]
          tunnel: [w1416] -> w1260
          tunnel: w1253 -> [w1414]
          shift-right: [w1408] -> _
          shift-left: 0 ("idxDataBlock") -> [w1409]
          shift-right: [w1405] -> _
          shift-left: w1244 -> [w1407]
          shift-right: [w1404] -> _
          shift-left: w1244 -> [w1406]
          shift-right: [w1394] -> w1238
          shift-left: 0 -> [w1378]
          shift-right: [w1369] -> _
          shift-left: w1224 -> [w1389]
          shift-right: [w1370] -> _
          shift-left: w1224 -> [w1385]
          shift-right: [w1398] -> _
          shift-left: FALSE -> [w1398]
          shift-right: [w1384] -> _
          shift-left: w1224 -> [w1392]
          shift-right: [w1395] -> w1239
          shift-left: w1240 -> [w1396]
          tunnel: w1227 -> [w1383]
          tunnel: [w1382] -> w1237
          tunnel: w1228 -> [w1379]
          tunnel: [w1379] -> w1236
          tunnel: w1226 -> [w1381]
          tunnel: [w1380] -> w1232
          shift-right: [w1374] -> _
          shift-left: w1231 -> [w1375]
          shift-right: [w1372] -> _
          shift-left: w1231 -> [w1373]
          shift-right: [w1366] -> _
          shift-left: u16 0 -> [w1367]
          shift-right: [w1364] -> _
          shift-left: w1224 -> [w1365]
          shift-right: [w1361] -> _
          shift-left: w1223 -> [w1362]
          stop <- w1457 stop-if-true
          # "arrTrig"
          # "arrTrig"
          # "LC_Laser_l2"
          # "LC_Event_l2"
          # "LC_Laser_l1"
          # "LC_Event_l1"
          # "CueLed"
          # "LC_Laser_l2"
          # "LC_Event_l2"
          # "LC_Laser_l1"
          # "LC_Event_l1"
          # "solenoid__R"
          # "solenoid__L"
          # "spout"
          # "Sel"
          # "Sel"
          # "iState"
          # "dataAnalog"
          # "index"
          # "iEvent"
          # "iBlock"
          # "iTrial"
          # "Laser"
          # "Audio R"
          # "Audio L"
          # "Solenoid R"
          # "Solenoid L"
          # "manual triggering"
          # "dataTrial"
          # "dataBlock"
          # "nRewards"
          # "dataExp"
          # "dataCurrent"
          # "audio__L\naudio__R"
          # "time stamp"
          # "Audio params"
          # "nRewards"
          # "idxDataBlock"
          # "idxDataBlock"
          # "activate"
          # "audio__L\naudio__R"
          # "amp__R\nfreq__R"
          # "amp__L\nfreq__L"
          # "dataLC"
          # "solenoid__R"
          # "solenoid__L"
          # "Did a lick occur?"
          # "Update lick counter"
          # "spout"
          # "spout"
          # "state"
          # "state"
          n831 = node-c288() -> ()  [unwired: 1 in, 1 out]
          n832 = local read "MTrig_Solenoid_trig__L"() -> (w1433:bool)
          n833 = local read "MTrig_Solenoid_trig__R"() -> (w1432:bool)
          n834 = local read "MTrig_Audio_trig__L"() -> (w1431:bool)
          n835 = local read "MTrig_Audio_trig__R"() -> (w1430:bool)
          n836 = xnode "Read/Write Control"("FPGA VI Reference In"=w1470, "error in"=w1469) -> ("FPGA VI Reference Out"=w1403:refnum<k20>, "error out"=w1402:errorcluster, "A2_LickL"=w1464:u32, "A4_LickR"=w1463:u32)
          "A2" <- w1464
          "A4" <- w1463
          n837 = local read "MTrig_Laser_trig"() -> (w1429:bool)
          n838 = Greater?(x=w1464, y=w1468) -> (0:w1466:bool)
          n839 = Greater?(x=w1463, y=w1467) -> (0:w1465:bool)
          n840 = Or(x=w1466, y=w1465) -> (x .or. y?=w1471:bool)
          n841 = call "myRIO_BRig_RT_dataMTrig_main.vi"("input_dataMTrig"=w1436, "input_Solenoid_trig_L"=w1433, "input_Solenoid_trig_R"=w1432, "input_Audio_trig_L"=w1431, "input_Audio_trig_R"=w1430, "input_Laser_trig"=w1429) -> ("output_Laser"=w1357:bool, "output_dataMTrig"=w1435:u16[], "output_Solenoid_L"=w1360:bool, "output_Solenoid_R"=w1425:bool, "output_Audio_L"=w1427:bool, "output_Audio_R"=w1428:bool)  [unwired: 8 in]
          n842 = Compound Arithmetic op=OR(w1433, w1432, w1431, w1430, w1429) -> (w1434:bool)
          n843 = case shown="True" w1434 {
            frame False {
            }
            frame True {
              w1473 = FALSE
              n844 = local write "MTrig_Solenoid_trig__L"(w1473) -> ()
              n845 = local write "MTrig_Solenoid_trig__R"(w1473) -> ()
              n846 = local write "MTrig_Audio_trig__L"(w1473) -> ()
              n847 = local write "MTrig_Audio_trig__R"(w1473) -> ()
              n848 = local write "MTrig_Laser_trig"(w1473) -> ()
            }
          }
          n849 = case shown="\"saveSettings1\"" w1371 {
            selector: w1371 -> [_ _ _ _ _ _ _ _ _ _ _ _ _ _ _ _ _ _ _ _ _ _ _ _ _ _ w2546 _ w2605 _ _ _ _ _ w2748 _ w2819 _ _ _ _ _ w2963 _ w3036 _ w3100 _ w3144 _ _ w3214 _ _ _ _ _ w3385 _ _ _ _ _ _ _ _ _ _ _ _ w3666 w3699]
            tunnel: [myRIO_BRig_RT__Case_Exp_stateList."Start2" ("Enum") myRIO_BRig_RT__Case_Exp_stateList."Start3" ("Enum") myRIO_BRig_RT__Case_Exp_stateList."saveSettings1" ("Enum") myRIO_BRig_RT__Case_Exp_stateList."saveSettings2" ("Enum") myRIO_BRig_RT__Case_Exp_stateList."saveSettings3" ("Enum") myRIO_BRig_RT__Case_Exp_stateList."saveSettings4" ("Enum") myRIO_BRig_RT__Case_Exp_stateList."saveSettings_LC_ENL_l1" ("Enum") myRIO_BRig_RT__Case_Exp_stateList."saveSettings_LC_ENL_l2" ("Enum") myRIO_BRig_RT__Case_Exp_stateList."saveSettings_LC_Cue_l1" ("Enum") myRIO_BRig_RT__Case_Exp_stateList."saveSettings_LC_Cue_l2" ("Enum") myRIO_BRig_RT__Case_Exp_stateList."saveSettings6_LC_l1_Other" ("Enum") myRIO_BRig_RT__Case_Exp_stateList."SaveSettings6_LC_l2_Other" ("Enum") myRIO_BRig_RT__Case_Exp_stateList."setSettings_Audio" ("Enum") myRIO_BRig_RT__Case_Exp_stateList."setSettings_Laser" ("Enum") myRIO_BRig_RT__Case_Exp_stateList."commConnect" ("Enum") w2256 myRIO_BRig_RT__Case_Exp_stateList."initTrial" ("Enum") w2301 myRIO_BRig_RT__Case_Exp_stateList."initTrial3" ("Enum") myRIO_BRig_RT__Case_Exp_stateList."initTrial_LC_ENL1" ("Enum") myRIO_BRig_RT__Case_Exp_stateList."ENL1_pre" ("Enum") myRIO_BRig_RT__Case_Exp_stateList."initTrial_LC_Cue1" ("Enum") myRIO_BRig_RT__Case_Exp_stateList."initTrial_LC_Cue1_2" ("Enum") myRIO_BRig_RT__Case_Exp_stateList."initTrial_LC_Sel" ("Enum") myRIO_BRig_RT__Case_Exp_stateList."initTrial4" ("Enum") w2507 w2543 myRIO_BRig_RT__Case_Exp_stateList."ENL1Penalty" ("Enum") w2606 myRIO_BRig_RT__Case_Exp_stateList."endExp" ("Enum") myRIO_BRig_RT__Case_Exp_stateList."endExp" ("Enum") myRIO_BRig_RT__Case_Exp_stateList."endExp" ("Enum") myRIO_BRig_RT__Case_Exp_stateList."endExp" ("Enum") w2705 w2747 myRIO_BRig_RT__Case_Exp_stateList."Cue1Penalty" ("Enum") w2817 myRIO_BRig_RT__Case_Exp_stateList."endExp" ("Enum") myRIO_BRig_RT__Case_Exp_stateList."endExp" ("Enum") myRIO_BRig_RT__Case_Exp_stateList."endExp" ("Enum") myRIO_BRig_RT__Case_Exp_stateList."endExp" ("Enum") w2926 w2962 myRIO_BRig_RT__Case_Exp_stateList."SelectReward" ("Enum") w3037 myRIO_BRig_RT__Case_Exp_stateList."SelectRewardPost" ("Enum") w3101 myRIO_BRig_RT__Case_Exp_stateList."SelectWrong" ("Enum") w3140 myRIO_BRig_RT__Case_Exp_stateList."endTrial1" ("Enum") myRIO_BRig_RT__Case_Exp_stateList."SelectTimeout" ("Enum") w3216 myRIO_BRig_RT__Case_Exp_stateList."endTrial1" ("Enum") myRIO_BRig_RT__Case_Exp_stateList."endTrial2" ("Enum") myRIO_BRig_RT__Case_Exp_stateList."endTrial3" ("Enum") w3302 w3368 w3385 myRIO_BRig_RT__Case_Exp_stateList."initBlock" ("Enum") w3412 myRIO_BRig_RT__Case_Exp_stateList."commUpload_dataExp" ("Enum") myRIO_BRig_RT__Case_Exp_stateList."endBlock" ("Enum") myRIO_BRig_RT__Case_Exp_stateList."commUpload_dataLC" ("Enum") myRIO_BRig_RT__Case_Exp_stateList."commUpload_dataTrial" ("Enum") myRIO_BRig_RT__Case_Exp_stateList."commUpload_dataCurrent" ("Enum") myRIO_BRig_RT__Case_Exp_stateList."saveData_dataCurrent" ("Enum") myRIO_BRig_RT__Case_Exp_stateList."saveData_dataExp" ("Enum") myRIO_BRig_RT__Case_Exp_stateList."saveData_dataLC" ("Enum") myRIO_BRig_RT__Case_Exp_stateList."saveData_dataTrial" ("Enum") myRIO_BRig_RT__Case_Exp_stateList."commUpload_pre" ("Enum") w3665 w3698] -> w1423
            tunnel: [w1502 w1521 w1543 w1604 w1658 w1726 w1793 w1857 w1921 w1985 w2049 w2092 w2136 w2162 w2227 w2233 w2264 w2278 w2315 w2352 w2384 w2408 w2431 w2448 w2485 w2523 w2559 w2586 w2610 w2626 w2648 w2667 w2686 w2722 w2769 w2791 w2816 w2837 w2858 w2877 w2896 w2937 w2986 w3011 w3034 w3048 w3098 w3122 w3154 w3175 w3195 w3226 w3249 w3261 w3280 w3322 w3341 w3384 w3401 w3415 w3449 w3470 w3491 w3512 w3533 w3561 w3581 w3608 w3628 w3652 w3686 w3719] -> w1368
            tunnel: w1472 -> [w1502 w1521 w1543 w1604 w1658 w1726 w1793 w1857 w1921 w1985 w2049 w2092 w2136 w2162 w2227 w2255 w2264 w2278 w2315 w2352 w2384 w2408 w2431 w2448 w2485 w2523 w2559 w2586 w2610 w2626 w2648 w2667 w2686 w2722 w2769 w2791 w2816 w2837 w2858 w2877 w2896 w2937 w2986 w3011 w3034 w3048 w3098 w3122 w3154 w3175 w3195 w3226 w3249 w3261 w3280 w3322 w3341 w3384 w3401 w3415 w3449 w3470 w3491 w3512 w3533 w3561 w3581 w3608 w3628 w3652 w3686 w3719]
            tunnel: w1471 -> [w1505 w1524 w1540 w1607 w1661 w1729 w1796 w1860 w1924 w1988 w2052 w2095 w2139 w2165 w2230 w2249 w2275 w2302 w2339 w2368 w2398 w2421 w2444 w2473 w2498 w2510 w2542 w2589 w2613 w2632 w2651 w2670 w2689 w2704 w2746 w2799 w2823 w2842 w2861 w2880 w2899 w2935 w2984 w3021 w3044 w3079 w3106 w3133 w3157 w3174 w3207 w3231 w3246 w3269 w3279 w3333 w3367 w3388 w3398 w3424 w3452 w3473 w3494 w3515 w3536 w3564 w3584 w3611 w3631 w3655 w3689 w3722]
            tunnel: w1466 -> [w1504 w1523 w1541 w1606 w1660 w1728 w1795 w1859 w1923 w1987 w2051 w2094 w2138 w2164 w2229 w2248 w2274 w2303 w2338 w2369 w2399 w2422 w2445 w2474 w2499 w2533 w2561 w2588 w2612 w2631 w2650 w2669 w2688 w2736 w2770 w2798 w2822 w2841 w2860 w2879 w2898 w2936 w2983 w3020 w3043 w3078 w3105 w3132 w3156 w3173 w3206 w3230 w3247 w3270 w3278 w3332 w3366 w3387 w3399 w3425 w3451 w3472 w3493 w3514 w3535 w3563 w3583 w3610 w3630 w3654 w3688 w3721]
            tunnel: w1465 -> [w1503 w1522 w1542 w1605 w1659 w1727 w1794 w1858 w1922 w1986 w2050 w2093 w2137 w2163 w2228 w2247 w2273 w2304 w2337 w2370 w2400 w2423 w2446 w2475 w2500 w2532 w2560 w2587 w2611 w2630 w2649 w2668 w2687 w2735 w2771 w2797 w2821 w2840 w2859 w2878 w2897 w2954 w2987 w3019 w3042 w3077 w3104 w3131 w3155 w3172 w3205 w3229 w3248 w3271 w3277 w3331 w3365 w3386 w3400 w3426 w3450 w3471 w3492 w3513 w3534 w3562 w3582 w3609 w3629 w3653 w3687 w3720]
            tunnel: [w1505 w1524 w1540 w1607 w1661 w1729 w1796 w1860 w1924 w1988 w2052 w2095 w2139 w2165 w2230 w2249 w2275 w2302 w2339 w2368 w2398 w2421 w2444 w2473 w2498 w2510 w2542 w2589 w2613 w2632 w2651 w2670 w2689 w2704 w2746 w2799 w2823 w2842 w2861 w2880 w2899 w2935 w2984 w3021 w3044 w3079 w3106 w3133 w3157 w3174 w3207 w3231 w3246 w3269 w3279 w3333 w3367 w3388 w3398 w3424 w3452 w3473 w3494 w3515 w3536 w3564 w3584 w3611 w3631 w3655 w3689 w3722] -> w1454
            tunnel: [w1504 w1523 w1541 w1606 w1660 w1728 w1795 w1859 w1923 w1987 w2051 w2094 w2138 w2164 w2229 w2248 w2274 w2303 w2338 w2369 w2399 w2422 w2445 w2474 w2499 w2533 w2561 w2588 w2612 w2631 w2650 w2669 w2688 w2736 w2770 w2798 w2822 w2841 w2860 w2879 w2898 w2936 w2983 w3020 w3043 w3078 w3105 w3132 w3156 w3173 w3206 w3230 w3247 w3270 w3278 w3332 w3366 w3387 w3399 w3425 w3451 w3472 w3493 w3514 w3535 w3563 w3583 w3610 w3630 w3654 w3688 w3721] -> w1453
            tunnel: [w1503 w1522 w1542 w1605 w1659 w1727 w1794 w1858 w1922 w1986 w2050 w2093 w2137 w2163 w2228 w2247 w2273 w2304 w2337 w2370 w2400 w2423 w2446 w2475 w2500 w2532 w2560 w2587 w2611 w2630 w2649 w2668 w2687 w2735 w2771 w2797 w2821 w2840 w2859 w2878 w2897 w2954 w2987 w3019 w3042 w3077 w3104 w3131 w3155 w3172 w3205 w3229 w3248 w3271 w3277 w3331 w3365 w3386 w3400 w3426 w3450 w3471 w3492 w3513 w3534 w3562 w3582 w3609 w3629 w3653 w3687 w3720] -> w1452
            tunnel: w1415 -> [w1501 w1520 w1539 w1571 w1634 w1703 w1778 w1856 w1920 w1984 w2048 w2091 w2135 w2160 w2203 w2254 w2263 w2300 w2314 w2353 w2383 w2407 w2430 w2458 w2484 w2522 w2545 w2580 w2609 w2627 w2647 w2666 w2685 w2708 w2766 w2790 w2820 w2838 w2857 w2876 w2895 w2921 w2965 w3003 w3039 w3050 w3103 w3123 w3153 w3171 w3196 w3228 w3245 w3258 w3282 w3304 w3339 w3383 w3402 w3427 w3446 w3467 w3488 w3509 w3520 w3550 w3569 w3593 w3625 w3641 w3664 w3697]
            tunnel: w1413 -> [w1500 w1519 w1538 w1602 w1656 w1723 w1790 w1854 w1918 w1982 w2046 w2089 w2133 w2153 w2223 w2253 w2272 w2299 w2322 w2351 w2386 w2411 w2434 w2463 w2488 w2525 w2558 w2579 w2607 w2629 w2646 w2665 w2684 w2724 w2768 w2788 w2815 w2839 w2856 w2875 w2894 w2947 w2985 w3017 w3041 w3071 w3099 w3124 w3151 w3170 w3198 w3225 w3244 w3268 w3285 w3303 w3358 w3382 w3403 w3428 w3445 w3466 w3487 w3508 w3521 w3558 w3578 w3589 w3624 w3649 w3683 w3716]
            tunnel: [w1501 w1520 w1539 w1571 w1634 w1702 w1777 w1856 w1920 w1984 w2048 w2091 w2135 w2160 w2209 w2238 w2263 w2288 w2314 w2353 w2383 w2406 w2429 w2457 w2483 w2526 w2544 w2581 w2608 w2627 w2647 w2666 w2685 w2731 w2765 w2789 w2818 w2838 w2857 w2876 w2895 w2948 w2964 w3018 w3038 w3072 w3102 w3125 w3152 w3171 w3199 w3227 w3245 w3257 w3281 w3304 w3337 w3383 w3402 w3427 w3446 w3467 w3488 w3509 w3520 w3550 w3569 w3593 w3625 w3641 w3664 w3697] -> w1449
            tunnel: [w1500 w1519 w1538 w1601 w1655 w1718 w1789 w1854 w1918 w1982 w2046 w2089 w2133 w2153 w2223 w2252 w2272 w2298 w2322 w2351 w2386 w2411 w2434 w2463 w2488 w2525 w2558 w2579 w2607 w2629 w2646 w2665 w2684 w2724 w2768 w2788 w2815 w2839 w2856 w2875 w2894 w2947 w2985 w3017 w3041 w3071 w3099 w3124 w3151 w3170 w3198 w3225 w3244 w3268 w3285 w3303 w3358 w3382 w3403 w3428 w3445 w3466 w3487 w3508 w3521 w3558 w3578 w3592 w3624 w3649 w3683 w3716] -> w1462
            tunnel: [_ _ _ _ _ _ _ _ _ _ _ _ _ _ _ _ _ _ _ _ _ _ _ _ _ _ _ _ _ _ _ _ _ _ _ _ _ _ _ _ _ _ _ _ w3032 _ _ _ _ _ _ _ _ _ _ _ _ _ _ _ _ _ _ _ _ _ _ _ _ _ _ _] -> w1359
            tunnel: [_ _ _ _ _ _ _ _ _ _ _ _ _ _ _ _ _ _ _ _ _ _ _ _ _ _ _ _ _ _ _ _ _ _ _ _ _ _ _ _ _ _ _ _ w3033 _ _ _ _ _ _ _ _ _ _ _ _ _ _ _ _ _ _ _ _ _ _ _ _ _ _ _] -> w1426
            tunnel: w1461 -> [w1498 w1517 w1536 w1573 w1636 w1724 w1791 w1855 w1919 w1983 w2047 w2090 w2134 w2158 w2224 w2250 w2265 w2296 w2330 w2366 w2396 w2403 w2426 w2447 w2480 w2524 w2557 w2576 w2603 w2628 w2644 w2663 w2682 w2730 w2767 w2787 w2813 w2835 w2854 w2873 w2892 w2946 w2981 w3009 w3040 w3052 w3096 w3121 w3149 w3168 w3197 w3224 w3242 w3260 w3287 w3329 w3350 w3380 w3405 w3430 w3443 w3464 w3485 w3506 w3530 w3544 w3571 w3599 w3618 w3643 w3677 w3710]
            tunnel: [w1498 w1517 w1536 w1573 w1636 w1724 w1791 w1855 w1919 w1983 w2047 w2090 w2134 w2158 w2224 w2250 w2262 w2296 w2330 w2366 w2396 w2403 w2426 w2447 w2480 w2524 w2557 w2576 w2603 w2628 w2644 w2663 w2682 w2730 w2767 w2787 w2813 w2835 w2854 w2873 w2892 w2946 w2981 w3009 w3040 w3051 w3096 w3121 w3149 w3168 w3197 w3224 w3242 w3259 w3287 w3329 w3350 w3380 w3405 w3430 w3443 w3464 w3485 w3506 w3530 w3544 w3571 w3599 w3618 w3643 w3677 w3710] -> w1460
            tunnel: w1459 -> [w1499 w1518 w1537 w1572 w1635 w1725 w1792 w1852 w1916 w1980 w2044 w2087 w2131 w2159 w2225 w2251 w2271 w2297 w2313 w2367 w2397 w2409 w2432 w2461 w2486 w2521 w2541 w2577 w2604 w2625 w2645 w2664 w2683 w2729 w2745 w2786 w2814 w2836 w2855 w2874 w2893 w2945 w2982 w3010 w3035 w3069 w3097 w3120 w3150 w3169 w3194 w3223 w3243 w3267 w3286 w3330 w3357 w3381 w3404 w3429 w3444 w3465 w3486 w3507 w3531 w3557 w3577 w3605 w3616 w3648 w3682 w3715]
            tunnel: [w1499 w1518 w1537 w1572 w1635 w1725 w1792 w1853 w1917 w1981 w2045 w2088 w2132 w2159 w2225 w2251 w2271 w2297 w2313 w2367 w2397 w2409 w2432 w2461 w2486 w2521 w2541 w2577 w2604 w2625 w2645 w2664 w2683 w2729 w2745 w2786 w2814 w2836 w2855 w2874 w2893 w2945 w2982 w3010 w3035 w3069 w3097 w3120 w3150 w3169 w3194 w3223 w3243 w3267 w3286 w3330 w3357 w3381 w3404 w3429 w3444 w3465 w3486 w3507 w3531 w3557 w3577 w3605 w3616 w3648 w3682 w3715] -> w1458
            tunnel: [_ _ _ _ _ _ _ _ _ _ _ _ _ _ _ _ _ _ _ _ _ _ _ _ _ _ _ _ _ _ _ _ _ _ _ _ _ _ _ _ _ _ _ _ _ _ _ _ _ _ _ _ _ _ _ _ _ TRUE _ _ _ _ _ _ _ _ _ _ _ _ _ _] -> w1455
            tunnel: w1445 -> [w1496 w1515 w1534 w1563 w1629 w1713 w1788 w1839 w1908 w1967 w2031 w2059 w2113 _ w2215 w2246 w2270 w2295 w2329 w2365 w2395 w2420 w2443 w2472 w2497 w2520 w2556 w2574 w2602 w2623 w2642 w2661 w2680 w2728 w2762 w2784 w2812 w2833 w2852 w2871 w2890 w2944 w2980 w2999 w3031 w3067 w3095 w3118 w3148 w3167 w3192 w3222 w3241 w3265 w3291 w3328 w3354 w3378 w3396 w3423 w3441 w3462 w3483 w3504 w3528 w3555 w3575 w3603 w3622 w3647 w3681 w3714]
            tunnel: w1444 -> [w1495 w1514 w1533 w1562 w1628 w1712 w1787 w1838 w1907 w1966 w2030 w2060 w2114 _ w2214 w2245 w2269 w2294 w2328 w2364 w2394 w2419 w2442 w2471 w2496 w2519 w2555 w2573 w2601 w2622 w2641 w2660 w2679 w2727 w2761 w2783 w2811 w2832 w2851 w2870 w2889 w2943 w2979 w2998 w3030 w3066 w3094 w3117 w3147 w3166 w3191 w3221 w3240 w3264 w3290 w3327 w3353 w3377 w3395 w3422 w3440 w3461 w3482 w3503 w3527 w3554 w3574 w3602 w3621 w3646 w3680 w3713]
            tunnel: w1443 -> [w1494 w1513 w1532 w1561 w1627 w1711 w1786 w1837 w1906 w1965 w2029 w2061 w2115 _ w2213 w2244 w2268 w2293 w2327 w2363 w2393 w2418 w2441 w2470 w2495 w2518 w2554 w2572 w2600 w2621 w2640 w2659 w2678 w2726 w2760 w2782 w2810 w2831 w2850 w2869 w2888 w2942 w2978 w2997 w3029 w3065 w3093 w3116 w3146 w3165 w3190 w3220 w3239 w3263 w3289 w3326 w3352 w3376 w3394 w3421 w3439 w3460 w3481 w3502 w3526 w3553 w3573 w3601 w3620 w3645 w3679 w3712]
            tunnel: w1442 -> [w1493 w1512 w1531 w1560 w1626 w1710 w1785 w1836 w1905 w1964 w2028 w2062 w2116 _ w2212 w2243 w2267 w2292 w2326 w2362 w2392 w2417 w2440 w2469 w2494 w2517 w2553 w2571 w2599 w2620 w2639 w2658 w2677 w2725 w2759 w2781 w2809 w2830 w2849 w2868 w2887 w2941 w2977 w2996 w3028 w3064 w3092 w3115 w3145 w3164 w3189 w3219 w3238 w3262 w3288 w3325 w3351 w3375 w3393 w3420 w3438 w3459 w3480 w3501 w3525 w3552 w3572 w3600 w3619 w3644 w3678 w3711]
            tunnel: w1441 -> [_ _ _ _ _ _ _ _ _ _ _ _ _ _ _ _ _ _ _ _ _ _ _ _ _ _ _ _ _ _ _ _ _ _ w2764 _ _ _ _ _ _ _ _ _ _ _ _ _ _ _ _ _ _ _ _ _ _ _ _ _ _ _ _ _ _ _ _ _ _ _ _ _]
            tunnel: w1440 -> [_ _ _ _ _ _ _ _ _ _ _ _ _ _ _ _ _ _ _ _ _ _ _ _ _ _ _ _ _ _ _ _ _ _ w2763 _ _ _ _ _ _ _ _ _ _ _ _ _ _ _ _ _ _ _ _ _ _ _ _ _ _ _ _ _ _ _ _ _ _ _ _ _]
            tunnel: [w1496 w1515 w1534 w1563 w1629 w1713 w1788 w1839 w1908 w1967 w2031 w2059 w2113 w2152 w2215 w2246 w2270 w2295 w2329 w2365 w2395 w2420 w2443 w2472 w2497 w2520 w2556 w2574 w2602 w2623 w2642 w2661 w2680 w2728 w2762 w2784 w2812 w2833 w2852 w2871 w2890 w2944 w2980 w2999 w3031 w3067 w3095 w3118 w3148 w3167 w3192 w3222 w3241 w3265 w3291 w3328 w3354 w3378 w3396 w3423 w3441 w3462 w3483 w3504 w3528 w3555 w3575 w3603 w3622 w3647 w3681 w3714] -> w1437
            tunnel: [w1495 w1514 w1533 w1562 w1628 w1712 w1787 w1838 w1907 w1966 w2030 w2060 w2114 w2143 w2214 w2245 w2269 w2294 w2328 w2364 w2394 w2419 w2442 w2471 w2496 w2519 w2555 w2573 w2601 w2622 w2641 w2660 w2679 w2727 w2761 w2783 w2811 w2832 w2851 w2870 w2889 w2943 w2979 w2998 w3030 w3066 w3094 w3117 w3147 w3166 w3191 w3221 w3240 w3264 w3290 w3327 w3353 w3377 w3395 w3422 w3440 w3461 w3482 w3503 w3527 w3554 w3574 w3602 w3621 w3646 w3680 w3713] -> w1410
            tunnel: [w1494 w1513 w1532 w1561 w1627 w1711 w1786 w1837 w1906 w1965 w2029 w2061 w2115 w2151 w2213 w2244 w2268 w2293 w2327 w2363 w2393 w2418 w2441 w2470 w2495 w2518 w2554 w2572 w2600 w2621 w2640 w2659 w2678 w2726 w2760 w2782 w2810 w2831 w2850 w2869 w2888 w2942 w2978 w2997 w3029 w3065 w3093 w3116 w3146 w3165 w3190 w3220 w3239 w3263 w3289 w3326 w3352 w3376 w3394 w3421 w3439 w3460 w3481 w3502 w3526 w3553 w3573 w3601 w3620 w3645 w3679 w3712] -> w1438
            tunnel: [w1493 w1512 w1531 w1560 w1626 w1710 w1785 w1836 w1905 w1964 w2028 w2062 w2116 w2141 w2212 w2243 w2267 w2292 w2326 w2362 w2392 w2417 w2440 w2469 w2494 w2517 w2553 w2571 w2599 w2620 w2639 w2658 w2677 w2725 w2759 w2781 w2809 w2830 w2849 w2868 w2887 w2941 w2977 w2996 w3028 w3064 w3092 w3115 w3145 w3164 w3189 w3219 w3238 w3262 w3288 w3325 w3351 w3375 w3393 w3420 w3438 w3459 w3480 w3501 w3525 w3552 w3572 w3600 w3619 w3644 w3678 w3711] -> w1439
            tunnel: [_ _ _ _ _ _ _ _ _ _ _ _ _ _ _ _ _ _ _ _ _ _ _ _ _ _ _ _ _ _ _ _ _ w2693 w2764 _ _ _ _ _ _ _ _ _ _ _ _ _ _ _ _ _ _ _ _ _ _ _ _ _ _ _ _ _ _ _ _ _ _ _ _ _] -> w1412
            tunnel: [_ _ _ _ _ _ _ _ _ _ _ _ _ _ _ _ _ _ _ _ _ _ _ _ _ _ _ _ _ _ _ _ _ w2691 w2763 _ _ _ _ _ _ _ _ _ _ _ _ _ _ _ _ _ _ _ _ _ _ _ _ _ _ _ _ _ _ _ _ _ _ _ _ _] -> w1411
            tunnel: w1422 -> [w1492 w1511 w1530 w1559 w1625 w1709 w1784 w1835 w1904 w1963 w2027 w2058 w2112 w2150 w2222 w2242 w2266 w2291 w2317 w2355 w2382 w2405 w2428 w2459 w2482 w2516 w2552 w2570 w2598 w2619 w2638 w2657 w2676 w2715 w2758 w2780 w2808 w2829 w2848 w2867 w2886 w2940 w2976 w2993 w3027 w3063 w3091 w3112 w3139 w3163 w3186 w3213 w3237 w3256 w3284 w3318 w3349 w3374 w3406 w3431 w3442 w3463 w3484 w3505 w3529 w3556 w3576 w3604 w3623 w3638 w3676 w3709]
            tunnel: [w1492 w1511 w1530 w1559 w1625 w1709 w1784 w1835 w1904 w1963 w2027 w2058 w2112 w2150 w2222 w2242 w2266 w2291 w2316 w2354 w2375 w2404 w2427 w2459 w2481 w2516 w2552 w2570 w2598 w2619 w2638 w2657 w2676 w2715 w2758 w2780 w2808 w2829 w2848 w2867 w2886 w2940 w2976 w2993 w3027 w3063 w3091 w3112 w3139 w3163 w3186 w3213 w3237 w3256 w3283 w3318 w3349 w3374 w3406 w3431 w3442 w3463 w3484 w3505 w3529 w3556 w3576 w3604 w3623 w3638 w3676 w3709] -> w1421
            tunnel: [w1491 w1510 w1529 w1558 w1624 w1708 w1783 w1834 w1903 w1962 w2026 w2057 w2111 w2149 w2221 w2241 w2277 w2290 w2332 w2361 w2391 w2416 w2439 w2468 w2493 w2515 w2551 w2569 w2597 w2618 w2637 w2656 w2675 w2714 w2757 w2779 w2807 w2828 w2847 w2866 w2885 w2939 w2975 w2992 w3026 w3062 w3090 w3111 w3138 w3162 w3185 w3212 w3236 w3255 w3276 w3324 w3348 w3372 w3407 w3417 w3437 w3458 w3479 w3500 w3524 w3560 w3580 w3607 w3627 w3651 w3685 w3718] -> w1420
            tunnel: [w1490 w1509 w1528 w1557 w1623 w1707 w1782 w1833 w1902 w1961 w2025 w2056 w2110 w2148 w2220 w2240 w2276 w2289 w2331 w2360 w2390 w2415 w2438 w2467 w2492 w2514 w2550 w2568 w2596 w2617 w2636 w2655 w2674 w2713 w2756 w2778 w2806 w2827 w2846 w2865 w2884 w2938 w2974 w2991 w3025 w3061 w3089 w3110 w3137 w3161 w3184 w3211 w3235 w3254 w3275 w3323 w3347 w3373 w3389 w3414 w3447 w3468 w3489 w3510 w3532 w3559 w3579 w3606 w3626 w3650 w3684 w3717] -> w1419
            tunnel: w1418 -> [w1491 w1510 w1529 w1558 w1624 w1708 w1783 w1834 w1903 w1962 w2026 w2057 w2111 w2149 w2221 w2241 w2277 w2290 w2332 w2361 w2391 w2416 w2439 w2468 w2493 w2515 w2551 w2569 w2597 w2618 w2637 w2656 w2675 w2714 w2757 w2779 w2807 w2828 w2847 w2866 w2885 w2939 w2975 w2992 w3026 w3062 w3090 w3111 w3138 w3162 w3185 w3212 w3236 w3255 w3276 w3324 w3348 w3372 _ w3417 w3437 w3458 w3479 w3500 w3524 w3560 w3580 w3607 w3627 w3651 w3685 w3718]
            tunnel: w1417 -> [w1490 w1509 w1528 w1557 w1623 w1707 w1782 w1833 w1902 w1961 w2025 w2056 w2110 w2148 w2220 w2240 w2276 w2289 w2331 w2360 w2390 w2415 w2438 w2467 w2492 w2514 w2550 w2568 w2596 w2617 w2636 w2655 w2674 w2713 w2756 w2778 w2806 w2827 w2846 w2865 w2884 w2938 w2974 w2991 w3025 w3061 w3089 w3110 w3137 w3161 w3184 w3211 w3235 w3254 w3275 w3323 w3347 w3373 _ w3414 w3447 w3468 w3489 w3510 w3532 w3559 w3579 w3606 w3626 w3650 w3684 w3717]
            tunnel: w1416 -> [_ _ _ _ _ _ _ _ _ _ _ _ _ _ _ _ _ _ _ _ _ _ _ _ _ _ _ _ _ _ _ _ _ _ _ _ _ _ _ _ _ _ _ _ _ _ _ _ _ _ _ _ _ _ _ _ _ _ _ _ w3435 w3456 w3477 w3498 w3522 _ _ _ _ _ _ _]
            tunnel: w1414 -> [_ _ _ _ _ _ _ _ _ _ _ _ _ _ _ _ _ _ _ _ _ _ _ _ _ _ _ _ _ _ _ _ _ _ _ _ _ _ _ _ _ _ _ _ _ _ _ _ _ _ _ _ _ _ _ _ _ _ _ _ _ _ _ _ _ _ _ w3594 _ _ _ _]
            tunnel: [w1489 w1508 w1527 w1556 w1622 w1706 w1781 w1832 w1901 w1960 w2024 w2055 w2109 w2147 w2219 w2236 w2260 w2286 w2333 w2359 w2389 w2414 w2437 w2466 w2491 w2513 w2549 w2567 w2595 w2616 w2635 w2654 w2673 w2712 w2755 w2777 w2805 w2826 w2845 w2864 w2883 w2934 w2973 w2990 w3024 w3046 w3088 w3109 w3136 w3160 w3183 w3210 w3234 w3253 w3274 w3321 w3334 w3371 w3392 w3416 w3434 w3455 w3476 w3497 w3519 w3539 w3568 w3588 w3615 w3636 w3675 w3708] -> w1408
            tunnel: w1409 -> [w1489 w1508 w1527 w1556 w1622 w1706 w1781 w1832 w1901 w1960 w2024 w2055 w2109 w2147 w2219 w2236 _ w2286 w2333 w2359 w2389 w2414 w2437 w2466 w2491 w2513 w2549 w2567 w2595 w2616 w2635 w2654 w2673 w2712 w2755 w2777 w2805 w2826 w2845 w2864 w2883 w2934 w2973 w2990 w3024 w3046 w3088 w3109 w3136 w3160 w3183 w3210 w3234 w3253 w3274 w3321 w3335 w3371 w3392 w3416 w3434 w3455 w3476 w3497 w3519 w3539 w3568 w3588 w3615 w3636 w3675 w3708]
            tunnel: w1407 -> [w1488 w1507 w1526 w1555 w1621 w1705 w1780 w1831 w1900 w1959 w2023 w2054 w2108 w2146 w2218 w2235 w2259 w2285 w2325 w2358 w2388 w2413 w2436 w2465 w2490 w2512 w2548 w2566 w2594 w2615 w2634 w2653 w2672 w2711 w2754 w2776 w2804 w2825 w2844 w2863 w2882 w2933 w2972 w2989 w3023 w3060 w3087 w3108 w3135 w3159 w3182 w3209 w3233 w3252 w3273 w3320 w3346 w3370 w3391 w3419 w3433 w3454 w3475 w3496 w3518 w3538 w3567 w3587 w3614 w3635 w3674 w3707]
            tunnel: w1406 -> [w1487 w1506 w1525 w1554 w1620 w1704 w1779 w1830 w1899 w1958 w2022 w2053 w2107 w2145 w2217 w2234 w2258 w2284 w2324 w2357 w2387 w2412 w2435 w2464 w2489 w2511 w2547 w2565 w2593 w2614 w2633 w2652 w2671 w2710 w2753 w2775 w2803 w2824 w2843 w2862 w2881 w2932 w2971 w2988 w3022 w3057 w3086 w3107 w3134 w3158 w3181 w3208 w3232 w3251 w3272 w3319 w3345 w3369 w3390 w3418 w3432 w3453 w3474 w3495 w3517 w3537 w3566 w3586 w3613 w3634 w3673 w3706]
            tunnel: [w1488 w1507 w1526 w1555 w1621 w1705 w1780 w1831 w1900 w1959 w2023 w2054 w2108 w2146 w2218 w2235 w2259 w2285 w2325 w2358 w2388 w2413 w2436 w2465 w2490 w2512 w2548 w2566 w2594 w2615 w2634 w2653 w2672 w2711 w2754 w2776 w2804 w2825 w2844 w2863 w2882 w2933 w2972 w2989 w3023 w3059 w3087 w3108 w3135 w3159 w3182 w3209 w3233 w3252 w3273 w3320 w3346 w3370 w3391 w3419 w3433 w3454 w3475 w3496 w3518 w3538 w3567 w3587 w3614 w3635 w3674 w3707] -> w1405
            tunnel: [w1487 w1506 w1525 w1554 w1620 w1704 w1779 w1830 w1899 w1958 w2022 w2053 w2107 w2145 w2217 w2234 w2258 w2284 w2324 w2357 w2387 w2412 w2435 w2464 w2489 w2511 w2547 w2565 w2593 w2614 w2633 w2652 w2671 w2710 w2753 w2775 w2803 w2824 w2843 w2862 w2881 w2932 w2971 w2988 w3022 w3058 w3086 w3107 w3134 w3158 w3181 w3208 w3232 w3251 w3272 w3319 w3345 w3369 w3390 w3418 w3432 w3453 w3474 w3495 w3517 w3537 w3566 w3586 w3613 w3634 w3673 w3706] -> w1404
            tunnel: w1403 -> [w1486 _ _ _ _ _ _ _ _ _ _ _ _ _ w2210 _ _ _ w2336 w2347 _ _ _ _ _ _ _ _ _ _ _ _ _ _ w2750 _ _ _ _ _ _ w2930 w2970 _ _ _ _ _ _ _ w3180 _ _ _ _ w3300 _ _ _ _ _ _ _ _ _ _ _ _ _ _ _ _]
            tunnel: w1402 -> [w1485 _ _ _ _ _ _ _ _ _ _ _ _ _ w2211 _ _ _ w2335 w2346 _ _ _ _ _ _ _ _ _ _ _ _ _ _ w2749 _ _ _ _ _ _ w2931 w2969 _ _ _ _ _ _ _ w3179 _ _ _ _ w3299 _ _ _ _ _ _ _ _ _ _ _ _ _ _ _ _]
            tunnel: [_ _ _ _ _ _ _ _ _ _ _ _ _ _ _ _ _ _ _ _ _ _ _ _ _ _ w2537 _ _ _ _ _ _ _ w2741 _ _ _ _ _ _ w2904 w2958 _ _ _ _ _ _ _ _ _ _ _ _ _ _ _ _ _ _ _ _ _ _ _ _ _ _ _ _ _] -> w1350
            tunnel: [_ _ _ _ _ _ _ _ _ _ _ _ _ _ _ _ _ _ _ _ _ _ _ _ _ _ w2536 _ _ _ _ _ _ _ w2740 _ _ _ _ _ _ w2903 w2957 _ _ _ _ _ _ _ _ _ _ _ _ _ _ _ _ _ _ _ _ _ _ _ _ _ _ _ _ _] -> w1349
            tunnel: [_ _ _ _ _ _ _ _ _ _ _ _ _ _ _ _ _ _ _ _ _ _ _ w2460 w2479 _ _ _ _ _ _ _ _ _ _ _ _ _ _ _ _ _ _ _ _ _ _ _ _ _ _ _ _ _ _ _ _ _ _ _ _ _ _ _ _ _ _ _ _ _ _ _] -> w1400
            tunnel: [_ _ _ _ _ _ _ _ _ _ _ _ _ _ _ _ _ _ _ _ _ _ _ _ TRUE ("Recording") _ _ _ _ _ _ _ _ _ _ _ _ _ _ _ _ _ _ _ _ _ _ _ _ _ _ _ _ _ _ _ _ _ _ _ _ _ _ _ _ _ _ _ _ _ _ _] -> w1397
            tunnel: [_ _ _ _ _ _ _ _ _ _ _ _ _ _ _ _ _ _ _ _ _ _ _ w2460 _ _ _ _ _ _ _ _ _ _ _ _ _ _ _ _ _ _ _ _ _ _ _ _ _ _ _ _ _ _ _ _ _ _ _ _ _ _ _ _ _ _ _ _ _ _ _ _] -> w1393
            tunnel: [_ _ _ _ _ _ _ _ _ _ _ _ _ _ _ TRUE _ _ _ _ _ _ _ _ _ _ _ _ _ _ _ _ _ _ _ _ _ _ _ _ _ _ _ _ _ _ _ _ _ _ _ _ _ _ _ _ _ _ _ _ _ _ _ _ _ _ _ _ _ _ _ _] -> w1390
            tunnel: [_ _ _ _ _ _ _ _ _ _ _ _ _ _ _ w2231 _ _ _ _ _ _ _ _ _ _ _ _ _ _ _ _ _ _ _ _ _ _ _ _ _ _ _ _ _ _ _ _ _ _ _ _ _ _ _ _ _ _ _ _ _ _ _ _ _ _ _ _ _ _ _ _] -> w1388
            tunnel: [_ _ _ _ _ _ _ _ _ _ _ _ _ _ _ _ _ TRUE _ _ _ _ _ _ _ _ _ _ _ _ _ _ _ _ _ _ _ _ _ _ _ _ _ _ _ _ _ _ _ _ _ _ _ _ _ _ _ _ _ _ _ _ _ _ _ _ _ _ _ _ _ _] -> w1387
            tunnel: [_ _ _ _ _ _ _ _ _ _ _ _ _ _ _ _ _ w2279 _ _ _ _ _ _ _ _ _ _ _ _ _ _ _ _ _ _ _ _ _ _ _ _ _ _ _ _ _ _ _ _ _ _ _ _ _ _ _ _ _ _ _ _ _ _ _ _ _ _ _ _ _ _] -> w1386
            tunnel: w1375 -> [_ _ _ _ _ _ _ _ _ _ _ _ _ _ _ _ _ _ _ _ w2373 _ _ _ _ w2503 w2540 w2564 w2592 _ _ _ _ w2699 w2744 w2774 w2802 _ _ _ _ w2918 w2966 _ _ _ _ _ _ _ _ _ _ _ _ _ _ _ _ _ _ _ _ _ _ _ _ _ _ _ _ _]
            tunnel: [_ _ _ _ _ _ _ _ _ _ _ _ _ _ _ _ _ _ _ _ w2373 _ _ _ _ w2503 w2540 w2564 w2592 _ _ _ _ w2699 w2744 w2774 w2802 _ _ _ _ w2918 w2966 _ _ _ _ _ _ _ _ _ _ _ _ _ _ _ _ _ _ _ _ _ _ _ _ _ _ _ _ _] -> w1374
            tunnel: w1373 -> [_ _ _ _ _ _ _ _ _ _ _ _ _ _ _ _ _ _ _ _ w2372 _ _ _ _ w2502 w2539 w2563 w2591 _ _ _ _ w2698 w2743 w2773 w2801 _ _ _ _ w2916 w2967 _ _ _ _ _ _ _ _ _ _ _ _ _ _ _ _ _ _ _ _ _ _ _ _ _ _ _ _ _]
            tunnel: [_ _ _ _ _ _ _ _ _ _ _ _ _ _ _ _ _ _ _ _ w2372 _ _ _ _ w2502 w2539 w2563 w2591 _ _ _ _ w2698 w2743 w2773 w2801 _ _ _ _ w2916 w2967 _ _ _ _ _ _ _ _ _ _ _ _ _ _ _ _ _ _ _ _ _ _ _ _ _ _ _ _ _] -> w1372
            tunnel: w1367 -> [_ _ _ _ _ _ _ _ _ _ _ _ _ _ _ _ _ _ _ _ _ _ _ _ _ _ _ _ _ _ _ _ _ _ _ _ _ _ _ _ _ _ _ _ _ _ _ _ _ _ _ _ _ _ _ _ _ _ _ _ _ _ _ _ _ _ _ _ _ _ w3671 w3704]
            tunnel: [_ _ _ _ _ _ _ _ _ _ _ _ _ _ _ _ _ _ _ _ _ _ _ _ _ _ _ _ _ _ _ _ _ _ _ _ _ _ _ _ _ _ _ _ _ _ _ _ _ _ _ _ _ _ _ _ _ _ _ _ _ _ _ _ _ _ _ _ _ _ w3669 w3702] -> w1366
            tunnel: w1362 -> [_ _ _ _ _ _ _ _ _ _ _ _ _ _ _ _ _ _ _ _ w2371 w2402 w2425 w2456 w2477 w2501 w2538 w2562 w2590 _ _ _ _ w2697 w2742 w2772 w2800 _ _ _ _ w2900 w2959 _ _ _ _ _ _ _ _ _ _ _ _ _ _ _ _ _ _ _ _ _ _ _ _ _ _ _ _ _]
            tunnel: [_ _ _ _ _ _ _ _ _ _ _ _ _ _ _ _ _ _ _ w2342 w2371 w2401 w2424 w2455 w2476 w2501 w2538 w2562 w2590 _ _ _ _ w2697 w2742 w2772 w2800 _ _ _ _ w2900 w2959 _ _ _ _ _ _ _ _ _ _ _ _ _ _ _ _ _ _ _ _ _ _ _ _ _ _ _ _ _] -> w1361
            tunnel: [_ _ _ _ _ _ _ _ _ _ _ _ _ _ _ _ _ _ _ _ _ _ _ _ _ _ w2535 _ _ _ _ _ _ _ w2739 _ _ _ _ _ _ w2902 w2956 _ _ _ _ _ _ _ _ _ _ _ _ _ _ _ _ _ _ _ _ _ _ _ _ _ _ _ _ _] -> w1354
            tunnel: [_ _ _ _ _ _ _ _ _ _ _ _ _ _ _ _ _ _ _ _ _ _ _ _ _ _ w2534 _ _ _ _ _ _ _ w2738 _ _ _ _ _ _ w2901 w2955 _ _ _ _ _ _ _ _ _ _ _ _ _ _ _ _ _ _ _ _ _ _ _ _ _ _ _ _ _] -> w1352
            tunnel: [_ _ _ _ _ _ _ _ _ _ _ _ _ _ _ _ _ _ _ _ _ _ _ _ _ _ _ _ _ _ _ _ _ _ w2737 _ _ _ _ _ _ _ _ _ _ _ _ _ _ _ _ _ _ _ _ _ _ _ _ _ _ _ _ _ _ _ _ _ _ _ _ _] -> w1358
            frame "Start1", Default {
              w1484 = FALSE ("SelectionState")
              n850 = xnode "Read/Write Control"("FPGA VI Reference In"=w1486, "error in"=w1485, "SelectionState"=w1484, "LR_reward_Laser_l1"=w1484, "LR_wrong_Laser_l1"=w1484, "LR_reward_Event_l1"=w1484, "LR_wrong_Event_l1"=w1484, "Left(F)_or_Right(T)"=w1484, "ignoreWrong"=w1484, "SelectionState"=w1484, "LR_reward_Laser_l2"=w1484, "LR_wrong_laser_l2"=w1484, "LR_reward_Event_l2"=w1484, "LR_wrong_Event_l2"=w1484, "LC_Event_l1"=w1484, "LC_Laser_l1"=w1484, "LC_Laser_l2"=w1484, "LC_Event_l2"=w1484, "CueLed_Event"=w1484) -> ()  [unwired: 2 out]
            }
            frame "Start2" {
            }
            frame "Start3" {
            }
            frame "saveSettings1" {
              n851 = call "myRIO_BRig_RT_dataExp_Audio_freq__L.vi"() -> ("output_Audio_freq__L"=w1579:i32)  [unwired: 11 in]
              n852 = call "myRIO_BRig_RT_dataExp_Audio_freq__R.vi"() -> ("output_Audio_freq__R"=w1578:i32)  [unwired: 11 in]
              n853 = call "myRIO_BRig_RT_dataExp_Audio_amp__L.vi"() -> ("output_Audio_amp__L"=w1577:i32)  [unwired: 11 in]
              n854 = call "myRIO_BRig_RT_dataExp_Audio_amp__R.vi"() -> ("output_Audio_amp__R"=w1575:i32)  [unwired: 11 in]
              n855 = call "myRIO_BRig_RT_dataExp_TPB_min__L.vi"() -> ("output_TPB_min__L"=w1587:i32)  [unwired: 11 in]
              n856 = call "myRIO_BRig_RT_dataExp_TPB_min__R.vi"() -> ("output_TPB_min__R"=w1585:i32)  [unwired: 11 in]
              n857 = call "myRIO_BRig_RT_dataExp_TPB_max__L.vi"() -> ("output_TPB_max__L"=w1583:i32)  [unwired: 11 in]
              n858 = call "myRIO_BRig_RT_dataExp_TPB_max__R.vi"() -> ("output_TPB_max__R"=w1581:i32)  [unwired: 11 in]
              n859 = call "myRIO_BRig_RT_dataExp_Cue1Param_AudioLed_Count_Switch.vi"() -> ("output_Cue1Param_AudioLed_Count_Switch"=w1549:i32)  [unwired: 11 in]
              n860 = call "myRIO_BRig_RT_dataExp_Cue1Param_AudioLed_Probability_Switch.vi"() -> ("output_Cue1Param_AudioLed_Probability_Switch"=w1547:i32)  [unwired: 11 in]
              n861 = call "myRIO_BRig_RT_dataExp_Cue1Param_CueType_Switch.vi"() -> ("output_Cue1Param_CueType_Switch"=w1545:i32)  [unwired: 11 in]
              n862 = call "myRIO_BRig_RT_dataExp_ItrialUntilReward.vi"() -> ("output_I_trialUntilReward"=w1600:i32)  [unwired: 11 in]
              n863 = call "myRIO_BRig_RT_dataExp_IblockUntilReward.vi"() -> ("output_I_blockUntilReward"=w1596:i32)  [unwired: 11 in]
              n864 = call "myRIO_BRig_RT_dataExp_CueCycles.vi"() -> ("output_CueCycles"=w1595:i32)  [unwired: 11 in]
              n865 = call "myRIO_BRig_RT_dataExp_ENL_min.vi"() -> ("output_ENL_min"=w1593:i32)  [unwired: 11 in]
              n866 = call "myRIO_BRig_RT_dataExp_ENL_max.vi"() -> ("output_ENL_max"=w1591:i32)  [unwired: 11 in]
              n867 = call "myRIO_BRig_RT_dataExp_ENL_penalty.vi"() -> ("output_ENL_penalty"=w1589:i32)  [unwired: 11 in]
              n868 = local read "Audio_Freq__L"() -> (w1553:u8)
              n869 = local read "Audio_Freq__R"() -> (w1551:u8)
              n870 = local read "Audio_Amp__L"() -> (w1576:u16)
              n871 = local read "TpB_Min_L"() -> (w1586:u16)
              n872 = local read "TpB_Min_R"() -> (w1584:u16)
              n873 = local read "TpB_Max_L"() -> (w1582:u16)
              n874 = local read "TpB_Max_R"() -> (w1580:u16)
              n875 = local read "Audio_Amp__R"() -> (w1574:u16)
              n876 = local read "TrialUntilReward"() -> (w1599:bool)
              n877 = local read "CueCycles"() -> (w1594:u16)
              n878 = local read "Tcycle_ENL_min"() -> (w1592:u16)
              n879 = local read "Tcycle_ENL_max"() -> (w1590:u16)
              n880 = local read "Tcycle_ENLPenalty"() -> (w1588:u16)
              n881 = local read "Cue1Param_AudioLed_Count_Switch"() -> (w1548:u16)
              n882 = local read "Cue1Param_AudioLed_Probability_Switch"() -> (w1546:u16)
              n883 = local read "Cue1Param_CueType_Switch"() -> (w1544:u16)
              n884 = To Unsigned Word Integer(number=w1551) -> (unsigned 16bit integer=w1550:u16)
              n885 = To Unsigned Word Integer(number=w1553) -> (unsigned 16bit integer=w1552:u16)
              n886 = Boolean To (0,1)(Boolean=w1599) -> (0, 1=w1598:i16)
              n887 = To Unsigned Word Integer(number=w1598) -> (unsigned 16bit integer=w1597:u16)
              n888 = local read "BUR_min"() -> (w1568:u16)
              n889 = local read "BUR_max"() -> (w1569:u16)
              n890 = Not Equal To 0?(x=w1568) -> (x != 0?=w1567:bool)
              n891 = Not Equal To 0?(x=w1569) -> (x != 0?=w1566:bool)
              n892 = And(x=w1567, y=w1566) -> (x .and. y?=w1565:bool)
              n893 = Boolean To (0,1)(Boolean=w1565) -> (0, 1=w1570:i16)
              n894 = To Unsigned Word Integer(number=w1570) -> (unsigned 16bit integer=w1564:u16)
              n895 = Replace Array Subset(array=w1602, new element #1=w1597, index #1=w1600, new element #2=w1564, index #2=w1596, new element #3=w1594, index #3=w1595, new element #4=w1592, index #4=w1593, new element #5=w1590, index #5=w1591, new element #6=w1588, index #6=w1589, new element #7=w1586, index #7=w1587, new element #8=w1584, index #8=w1585, new element #9=w1582, index #9=w1583, new element #10=w1580, index #10=w1581, new element #11=w1552, index #11=w1579, new element #12=w1550, index #12=w1578, new element #13=w1576, index #13=w1577, new element #14=w1574, index #14=w1575, new element #15=w1548, index #15=w1549, new element #16=w1546, index #16=w1547, new element #17=w1544, index #17=w1545) -> (w1601:u16[])
            }
            frame "saveSettings2" {
              n896 = call "myRIO_BRig_RT_dataExp_Tcycle_RewardPost.vi"() -> ("output_Tcycle_RewardPost"=w1645:i32)  [unwired: 11 in]
              n897 = call "myRIO_BRig_RT_dataExp_Tcycle_Wrong.vi"() -> ("output_Tcycle_Wrong"=w1643:i32)  [unwired: 11 in]
              n898 = call "myRIO_BRig_RT_dataExp_Tcycle_Timeout.vi"() -> ("output_Tcycle_Timeout"=w1641:i32)  [unwired: 11 in]
              n899 = call "myRIO_BRig_RT_dataExp_Tcycle_Cue_min.vi"() -> ("output_Tcycle_Cue_min"=w1639:i32)  [unwired: 11 in]
              n900 = call "myRIO_BRig_RT_dataExp_Tcycle_Cue_max.vi"() -> ("output_Tcycle_Cue_max"=w1638:i32)  [unwired: 11 in]
              n901 = call "myRIO_BRig_RT_dataExp_Tcycle_CuePenalty.vi"() -> ("output_Tcycle_CuePenalty"=w1637:i32)  [unwired: 11 in]
              n902 = call "myRIO_BRig_RT_dataExp_SolenoidProbability_L.vi"() -> ("output_SolenoidProbability_L"=w1617:i32)  [unwired: 11 in]
              n903 = call "myRIO_BRig_RT_dataExp_SolenoidProbability_R.vi"() -> ("output_SolenoidProbability_R"=w1616:i32)  [unwired: 11 in]
              n904 = call "myRIO_BRig_RT_dataExp_nBlock.vi"() -> ("output_nBlock"=w1654:i32)  [unwired: 11 in]
              n905 = call "myRIO_BRig_RT_dataExp_nTrial.vi"() -> ("output_nTrial"=w1653:i32)  [unwired: 11 in]
              n906 = call "myRIO_BRig_RT_dataExp_runTime_seconds.vi"() -> ("output_RunTime_minutes"=w1652:i32)  [unwired: 11 in]
              n907 = call "myRIO_BRig_RT_dataExp_Tcycle_Selection.vi"() -> ("output_Tcycle_Selection"=w1651:i32)  [unwired: 11 in]
              n908 = call "myRIO_BRig_RT_dataExp_Tcycle_Reward__L.vi"() -> ("output_Tcycle_Reward__L"=w1649:i32)  [unwired: 11 in]
              n909 = call "myRIO_BRig_RT_dataExp_Tcycle_Reward__R.vi"() -> ("output_Tcycle_Reward__R"=w1647:i32)  [unwired: 11 in]
              n910 = local read "Tcycle_RewardPost"() -> (w1644:u16)
              n911 = local read "Tcycle_Wrong"() -> (w1642:u16)
              n912 = local read "Tcycle_Timeout"() -> (w1640:u16)
              n913 = call "myRIO_BRig_RT_dataExp_Cue1Param_AudioLed_Count_NS.vi"() -> ("output_Cue1Param_AudioLed_Count_NS"=w1613:i32)  [unwired: 11 in]
              n914 = call "myRIO_BRig_RT_dataExp_Cue1Param_AudioLed_Probability_NS.vi"() -> ("output_Cue1Param_AudioLed_Probability_NS"=w1611:i32)  [unwired: 11 in]
              n915 = call "myRIO_BRig_RT_dataExp_Cue1Param_CueType_NS.vi"() -> ("output_Cue1Param_CueType_NS"=w1609:i32)  [unwired: 11 in]
              n916 = local read "Tcycle_CuePenalty"() -> (w1630:u16)
              n917 = local read "Tcycle_Cue_max"() -> (w1618:u16)
              n918 = local read "Tcycle_Cue_min"() -> (w1619:u16)
              n919 = local read "Tcycle_Selection"() -> (w1650:u16)
              n920 = local read "Tcycle_Reward_L"() -> (w1648:u16)
              n921 = local read "Tcycle_Reward_R"() -> (w1646:u16)
              n922 = local read "SolenoidProbability_R"() -> (w1614:u16)
              n923 = local read "SolenoidProbability_L"() -> (w1615:u16)
              n924 = local read "Cue1Param_AudioLed_Count_NS"() -> (w1612:u16)
              n925 = local read "Cue1Param_AudioLed_Probability_NS"() -> (w1610:u16)
              n926 = local read "Cue1Param_CueType_NS"() -> (w1608:u16)
              n927 = Replace Array Subset(array=w1656, new element #1=u16 0, index #1=w1654, new element #2=u16 0, index #2=w1653, new element #3=u16 0, index #3=w1652, new element #4=w1650, index #4=w1651, new element #5=w1648, index #5=w1649, new element #6=w1646, index #6=w1647, new element #7=w1644, index #7=w1645, new element #8=w1642, index #8=w1643, new element #9=w1640, index #9=w1641, new element #10=w1619, index #10=w1639, new element #11=w1618, index #11=w1638, new element #12=w1630, index #12=w1637, new element #13=w1615, index #13=w1617, new element #14=w1614, index #14=w1616, new element #15=w1612, index #15=w1613, new element #16=w1610, index #16=w1611, new element #17=w1608, index #17=w1609) -> (w1655:u16[])
            }
            frame "saveSettings3" {
              w1667 = 100.0 ("y")
              n928 = call "myRIO_BRig_RT_dataExp_laser1_Freq.vi"() -> ("output_laser1_Freq"=w1700:i32)  [unwired: 11 in]
              n929 = call "myRIO_BRig_RT_dataExp_laser1_Tpeak.vi"() -> ("output_laser1_Tpeak"=w1695:i32)  [unwired: 11 in]
              n930 = call "myRIO_BRig_RT_dataExp_laser1_Tshutter.vi"() -> ("output_laser1_Tshutter"=w1690:i32)  [unwired: 11 in]
              n931 = call "myRIO_BRig_RT_dataExp_FPGA_f_count2ms.vi"() -> ("output_FPGA_f_count2ms"=w1685:i32)  [unwired: 11 in]
              n932 = call "myRIO_BRig_RT_dataExp_laser1_Power_min.vi"() -> ("output_laser1_Power_min"=w1680:i32)  [unwired: 11 in]
              n933 = call "myRIO_BRig_RT_dataExp_laser1_Power_max.vi"() -> ("output_laser1_Power_max"=w1673:i32)  [unwired: 11 in]
              n934 = call "myRIO_BRig_RT_dataExp_laser1_Power_step.vi"() -> ("output_laser1_Power_step"=w1672:i32)  [unwired: 11 in]
              n935 = call "myRIO_BRig_RT_dataExp_laser1_duration.vi"() -> ("output_laser1_duration"=w1675:i32)  [unwired: 11 in]
              n936 = local read "Laser_Tshutter_l1"() -> (w1687:dbl)
              n937 = local read "Laser_Tpeak_l1"() -> (w1692:dbl)
              n938 = local read "Laser_power_max_l1"() -> (w1666:dbl)
              n939 = local read "Laser_power_step_l1"() -> (w1665:dbl)
              n940 = local read "Laser_power_min_l1"() -> (w1677:dbl)
              n941 = local read "Laser_Freq_l1"() -> (w1699:dbl)
              n942 = call "myRIO_BRig_RT_dataExp_BUR_min.vi"() -> ("output_BUR_min"=w1722:i32)  [unwired: 11 in]
              n943 = call "myRIO_BRig_RT_dataExp_BUR_max.vi"() -> ("output_BUR_max"=w1720:i32)  [unwired: 11 in]
              n944 = call "myRIO_BRig_RT_dataExp_Audio_sp__L.vi"() -> ("output_Audio_sp__L"=w1717:i32)  [unwired: 11 in]
              n945 = call "myRIO_BRig_RT_dataExp_Audio_sp__R.vi"() -> ("output_Audio_sp__R"=w1716:i32)  [unwired: 11 in]
              n946 = local read "FPGA_count2ms"() -> (w1682:dbl)
              n947 = local read "sp_LeftSpout"() -> (w1715:u16)
              n948 = local read "BUR_max"() -> (w1719:u16)
              n949 = local read "sp_RightSpout"() -> (w1714:u16)
              n950 = local read "BUR_min"() -> (w1721:u16)
              n951 = Multiply(x=w1699, y=w1667) -> (x*y=w1698:dbl)
              n952 = Multiply(x=w1692, y=w1667) -> (x*y=w1694:dbl)
              n953 = Multiply(x=w1687, y=w1667) -> (x*y=w1689:dbl)
              n954 = Multiply(x=w1682, y=w1667) -> (x*y=w1684:dbl)
              n955 = Multiply(x=w1677, y=w1667) -> (x*y=w1679:dbl)
              n956 = Multiply(x=w1666, y=w1667) -> (x*y=w1671:dbl)
              n957 = Multiply(x=w1665, y=w1667) -> (x*y=w1669:dbl)
              n958 = Round To Nearest(number=w1698) -> (nearest integer value=w1697:dbl)
              n959 = Round To Nearest(number=w1694) -> (nearest integer value=w1693:dbl)
              n960 = Round To Nearest(number=w1689) -> (nearest integer value=w1688:dbl)
              n961 = Round To Nearest(number=w1684) -> (nearest integer value=w1683:dbl)
              n962 = Round To Nearest(number=w1679) -> (nearest integer value=w1678:dbl)
              n963 = Round To Nearest(number=w1671) -> (nearest integer value=w1670:dbl)
              n964 = Round To Nearest(number=w1669) -> (nearest integer value=w1668:dbl)
              n965 = To Unsigned Word Integer(number=w1697) -> (unsigned 16bit integer=w1696:u16)
              n966 = To Unsigned Word Integer(number=w1693) -> (unsigned 16bit integer=w1691:u16)
              n967 = To Unsigned Word Integer(number=w1688) -> (unsigned 16bit integer=w1686:u16)
              n968 = To Unsigned Word Integer(number=w1683) -> (unsigned 16bit integer=w1681:u16)
              n969 = To Unsigned Word Integer(number=w1678) -> (unsigned 16bit integer=w1676:u16)
              n970 = To Unsigned Word Integer(number=w1670) -> (unsigned 16bit integer=w1664:u16)
              n971 = To Unsigned Word Integer(number=w1668) -> (unsigned 16bit integer=w1663:u16)
              n972 = local read "Laser_duration_l1"() -> (w1674:u16)
              n973 = call "myRIO_BRig_RT_dataCurrent_laser1_pulse_duration.vi"() -> ("output_laser1_pulse_duration"=w1701:i32)  [unwired: 11 in]
              n974 = Replace Array Subset(array=w1723, new element #1=w1721, index #1=w1722, new element #2=w1719, index #2=w1720, new element #3=w1715, index #3=w1717, new element #4=w1714, index #4=w1716, new element #5=w1696, index #5=w1700, new element #6=w1691, index #6=w1695, new element #7=w1686, index #7=w1690, new element #8=w1681, index #8=w1685, new element #9=w1676, index #9=w1680, new element #10=w1664, index #10=w1673, new element #11=w1663, index #11=w1672, new element #12=w1674, index #12=w1675) -> (w1718:u16[])
              n975 = Replace Array Subset(array=w1703, new element=w1674, index=w1701) -> (w1702:u16[])
            }
            frame "saveSettings4" {
              w1744 = 100.0 ("y")
              n976 = call "myRIO_BRig_RT_dataExp_laser2_Freq.vi"() -> ("output_laser2_Freq"=w1731:i32)  [unwired: 11 in]
              n977 = call "myRIO_BRig_RT_dataExp_laser2_Tpeak.vi"() -> ("output_laser2_Tpeak"=w1733:i32)  [unwired: 11 in]
              n978 = call "myRIO_BRig_RT_dataExp_laser2_Tshutter.vi"() -> ("output_laser2_Tshutter"=w1735:i32)  [unwired: 11 in]
              n979 = call "myRIO_BRig_RT_dataExp_laser2_Power_min.vi"() -> ("output_laser2_Power_min"=w1752:i32)  [unwired: 11 in]
              n980 = call "myRIO_BRig_RT_dataExp_laser2_Power_max.vi"() -> ("output_laser2_Power_max"=w1751:i32)  [unwired: 11 in]
              n981 = call "myRIO_BRig_RT_dataExp_laser2_Power_step.vi"() -> ("output_laser2_Power_step"=w1750:i32)  [unwired: 11 in]
              n982 = call "myRIO_BRig_RT_dataExp_laser2_duration.vi"() -> ("output_laser2_duration"=w1749:i32)  [unwired: 11 in]
              n983 = call "myRIO_BRig_RT_dataExp_CueLed_Freq.vi"() -> ("output_CueLed_Freq"=w1741:i32)  [unwired: 11 in]
              n984 = call "myRIO_BRig_RT_dataExp_CueLed_Tpeak.vi"() -> ("output_CueLed_Tpeak"=w1740:i32)  [unwired: 11 in]
              n985 = call "myRIO_BRig_RT_dataExp_CueLed_duration.vi"() -> ("output_CueLed_duration"=w1737:i32)  [unwired: 11 in]
              n986 = local read "Laser_Tshutter_l2"() -> (w1768:dbl)
              n987 = local read "Laser_Tpeak_l2"() -> (w1771:dbl)
              n988 = local read "Laser_power_max_l2"() -> (w1758:dbl)
              n989 = local read "Laser_power_step_l2"() -> (w1757:dbl)
              n990 = local read "Laser_power_min_l2"() -> (w1765:dbl)
              n991 = local read "Laser_Freq_l2"() -> (w1776:dbl)
              n992 = local read "CueLed_Tpeak"() -> (w1742:dbl)
              n993 = local read "CueLed_duration"() -> (w1736:u16)
              n994 = local read "CueLed_Freq"() -> (w1743:dbl)
              n995 = Multiply(x=w1776, y=w1744) -> (x*y=w1775:dbl)
              n996 = Multiply(x=w1771, y=w1744) -> (x*y=w1773:dbl)
              n997 = Multiply(x=w1768, y=w1744) -> (x*y=w1770:dbl)
              n998 = Multiply(x=w1765, y=w1744) -> (x*y=w1767:dbl)
              n999 = Multiply(x=w1758, y=w1744) -> (x*y=w1762:dbl)
              n1000 = Multiply(x=w1757, y=w1744) -> (x*y=w1760:dbl)
              n1001 = Multiply(x=w1743, y=w1744) -> (x*y=w1745:dbl)
              n1002 = Multiply(x=w1742, y=w1744) -> (x*y=w1746:dbl)
              n1003 = Round To Nearest(number=w1775) -> (nearest integer value=w1774:dbl)
              n1004 = Round To Nearest(number=w1773) -> (nearest integer value=w1772:dbl)
              n1005 = Round To Nearest(number=w1770) -> (nearest integer value=w1769:dbl)
              n1006 = Round To Nearest(number=w1767) -> (nearest integer value=w1766:dbl)
              n1007 = Round To Nearest(number=w1762) -> (nearest integer value=w1761:dbl)
              n1008 = Round To Nearest(number=w1760) -> (nearest integer value=w1759:dbl)
              n1009 = Round To Nearest(number=w1745) -> (nearest integer value=w1748:dbl)
              n1010 = Round To Nearest(number=w1746) -> (nearest integer value=w1747:dbl)
              n1011 = To Unsigned Word Integer(number=w1774) -> (unsigned 16bit integer=w1730:u16)
              n1012 = To Unsigned Word Integer(number=w1772) -> (unsigned 16bit integer=w1732:u16)
              n1013 = To Unsigned Word Integer(number=w1769) -> (unsigned 16bit integer=w1734:u16)
              n1014 = To Unsigned Word Integer(number=w1766) -> (unsigned 16bit integer=w1764:u16)
              n1015 = To Unsigned Word Integer(number=w1761) -> (unsigned 16bit integer=w1756:u16)
              n1016 = To Unsigned Word Integer(number=w1759) -> (unsigned 16bit integer=w1755:u16)
              n1017 = To Unsigned Word Integer(number=w1748) -> (unsigned 16bit integer=w1739:u16)
              n1018 = To Unsigned Word Integer(number=w1747) -> (unsigned 16bit integer=w1738:u16)
              n1019 = local read "Laser_duration_l2"() -> (w1763:u16)
              n1020 = call "myRIO_BRig_RT_dataCurrent_laser2_pulse_duration.vi"() -> ("output_laser2_pulse_duration"=w1753:i32)  [unwired: 11 in]
              n1021 = Replace Array Subset(array=w1778, new element=w1763, index=w1753) -> (w1777:u16[])
              n1022 = Replace Array Subset(array=w1790, new element #1=w1730, index #1=w1731, new element #2=w1732, index #2=w1733, new element #3=w1734, index #3=w1735, new element #4=w1764, index #4=w1752, new element #5=w1756, index #5=w1751, new element #6=w1755, index #6=w1750, new element #7=w1763, index #7=w1749, new element #8=w1739, index #8=w1741, new element #9=w1738, index #9=w1740, new element #10=w1736, index #10=w1737) -> (w1789:u16[])
            }
            frame "saveSettings_LC_ENL_l1" {
              # "Selection First"
              # "Count"
              # "Tdelay"
              # "Probability"
              # "OnOff"
              # "Block"
              # "delayOpt"
              # "Count"
              # "Tdelay"
              # "Probability"
              # "OnOff"
              # "Block"
              # "ENL1 All"
              # "delayOpt"
              # "Count"
              # "Tdelay"
              # "Probability"
              # "OnOff"
              # "Block"
              # "ENL1 First"
              n1023 = local read "LC_ENL1_delayOpt_Switch_l1"() -> (w1828:bool)
              n1024 = call "myRIO_BRig_RT_dataLC_ENL1_Block_NS_l1.vi"() -> ("output_ENL1_All_Block"=w1825:i32)  [unwired: 11 in]
              n1025 = call "myRIO_BRig_RT_dataLC_ENL1_OnOff_NS_l1.vi"() -> ("output_ENL1_OnOff_NS_l1"=w1815:i32)  [unwired: 11 in]
              n1026 = call "myRIO_BRig_RT_dataLC_ENL1_Probability_NS_l1.vi"() -> ("output_ENL1_Probability_NS_l1"=w1814:i32)  [unwired: 11 in]
              n1027 = call "myRIO_BRig_RT_dataLC_ENL1_Tdelay_NS_l1.vi"() -> ("output_ENL1_Tdelay_NS_l1"=w1813:i32)  [unwired: 11 in]
              n1028 = call "myRIO_BRig_RT_dataLC_ENL1_Count_NS_l1.vi"() -> ("output_ENL1_Count_NS_l1"=w1812:i32)  [unwired: 11 in]
              n1029 = call "myRIO_BRig_RT_dataLC_ENL1_delayOpt_NS_l1.vi"() -> ("output_ENL1_delayOpt_NS_l1"=w1811:i32)  [unwired: 11 in]
              n1030 = call "myRIO_BRig_RT_dataLC_ENL1_Block_Switch_l1.vi"() -> ("output_ENL1_Block_Switch_l1"=w1851:i32)  [unwired: 11 in]
              n1031 = call "myRIO_BRig_RT_dataLC_ENL1_OnOff_Switch_l1.vi"() -> ("output_ENL1_OnOff_Switch_l1"=w1849:i32)  [unwired: 11 in]
              n1032 = call "myRIO_BRig_RT_dataLC_ENL1_Probability_Switch_l1.vi"() -> ("output_ENL1_Probability_Switch_l1"=w1845:i32)  [unwired: 11 in]
              n1033 = call "myRIO_BRig_RT_dataLC_ENL1_Tdelay_Switch_l1.vi"() -> ("output_ENL1_Tdelay_Switch_l1"=w1843:i32)  [unwired: 11 in]
              n1034 = call "myRIO_BRig_RT_dataLC_ENL1_Count_Switch_l1.vi"() -> ("output_ENL1_Count_Switch_l1"=w1841:i32)  [unwired: 11 in]
              n1035 = call "myRIO_BRig_RT_dataLC_ENL1_delayOpt_Switch_l1.vi"() -> ("output_ENL1_delayOpt_Switch_l1"=w1827:i32)  [unwired: 11 in]
              n1036 = local read "LC_ENL1_Count_Switch_l1"() -> (w1840:u16)
              n1037 = local read "LC_ENL1_Probability_Switch_l1"() -> (w1844:u16)
              n1038 = local read "LC_ENL1_Block_Switch_l1"() -> (w1850:u16)
              n1039 = local read "LC_ENL1_Tdelay_Switch_l1"() -> (w1842:u16)
              n1040 = local read "LC_ENL1_OnOff_Switch_l1"() -> (w1848:bool)
              n1041 = call "myRIO_BRig_RT_dataLC_Selection_Block_Switch_l1.vi"() -> ("output_Selection_Block_Switch_l1"=w1809:i32)  [unwired: 11 in]
              n1042 = call "myRIO_BRig_RT_dataLC_Selection_OnOff_Switch_l1.vi"() -> ("output_Selection_OnOff_Switch_l1"=w1808:i32)  [unwired: 11 in]
              n1043 = call "myRIO_BRig_RT_dataLC_Selection_Probability_Switch_l1.vi"() -> ("output_Selection_Probability_Switch_l1"=w1807:i32)  [unwired: 11 in]
              n1044 = call "myRIO_BRig_RT_dataLC_Selection_Tdelay_Switch_l1.vi"() -> ("output_Selection_Tdelay_Switch_l1"=w1806:i32)  [unwired: 11 in]
              n1045 = call "myRIO_BRig_RT_dataLC_Selection_Count_Switch_l1.vi"() -> ("output_Selection_Count_Switch_l1"=w1805:i32)  [unwired: 11 in]
              n1046 = local read "LC_ENL1_OnOff_NS_l1"() -> (w1821:bool)
              n1047 = local read "LC_ENL1_Probability_NS_l1"() -> (w1819:u16)
              n1048 = local read "LC_ENL1_delayOpt_NS_l1"() -> (w1817:bool)
              n1049 = local read "LC_Sel_Probability_Switch_l1"() -> (w1800:u16)
              n1050 = local read "LC_ENL1_Tdelay_NS_l1"() -> (w1810:u16)
              n1051 = local read "LC_ENL1_Block_NS_l1"() -> (w1822:u16)
              n1052 = local read "LC_ENL1_Count_NS_l1"() -> (w1818:u16)
              n1053 = local read "LC_Sel_Tdelay_Switch_l1"() -> (w1799:u16)
              n1054 = local read "LC_Sel_OnOff_Switch_l1"() -> (w1803:bool)
              n1055 = local read "LC_Sel_Count_Switch_l1"() -> (w1798:u16)
              n1056 = local read "LC_Sel_Block_Switch_l1"() -> (w1802:u16)
              n1057 = Boolean To (0,1)(Boolean=w1828) -> (0, 1=w1829:i16)
              n1058 = Boolean To (0,1)(Boolean=w1848) -> (0, 1=w1847:i16)
              n1059 = Boolean To (0,1)(Boolean=w1821) -> (0, 1=w1824:i16)
              n1060 = To Unsigned Word Integer(number=w1829) -> (unsigned 16bit integer=w1826:u16)
              n1061 = To Unsigned Word Integer(number=w1847) -> (unsigned 16bit integer=w1846:u16)
              n1062 = Boolean To (0,1)(Boolean=w1817) -> (0, 1=w1823:i16)
              n1063 = To Unsigned Word Integer(number=w1824) -> (unsigned 16bit integer=w1820:u16)
              n1064 = Boolean To (0,1)(Boolean=w1803) -> (0, 1=w1804:i16)
              n1065 = To Unsigned Word Integer(number=w1823) -> (unsigned 16bit integer=w1816:u16)
              n1066 = To Unsigned Word Integer(number=w1804) -> (unsigned 16bit integer=w1801:u16)
              n1067 = Replace Array Subset(array=w1852, new element #1=w1850, index #1=w1851, new element #2=w1846, index #2=w1849, new element #3=w1844, index #3=w1845, new element #4=w1842, index #4=w1843, new element #5=w1840, index #5=w1841, new element #6=w1826, index #6=w1827, new element #7=w1822, index #7=w1825, new element #8=w1820, index #8=w1815, new element #9=w1819, index #9=w1814, new element #10=w1810, index #10=w1813, new element #11=w1818, index #11=w1812, new element #12=w1816, index #12=w1811, new element #13=w1802, index #13=w1809, new element #14=w1801, index #14=w1808, new element #15=w1800, index #15=w1807, new element #16=w1799, index #16=w1806, new element #17=w1798, index #17=w1805) -> (w1853:u16[])
            }
            frame "saveSettings_LC_ENL_l2" {
              # "Selection First"
              # "Count"
              # "Tdelay"
              # "Probability"
              # "OnOff"
              # "Block"
              # "delayOpt"
              # "Count"
              # "Tdelay"
              # "Probability"
              # "OnOff"
              # "Block"
              # "ENL1 All"
              # "delayOpt"
              # "Count"
              # "Tdelay"
              # "Probability"
              # "OnOff"
              # "Block"
              # "ENL1 First"
              n1068 = call "myRIO_BRig_RT_dataLC_ENL1_Block_Switch_l2.vi"() -> ("output_ENL1_Block_Switch_l2"=w1872:i32)  [unwired: 11 in]
              n1069 = call "myRIO_BRig_RT_dataLC_ENL1_OnOff_Switch_l2.vi"() -> ("output_ENL1_OnOff_Switch_l2"=w1873:i32)  [unwired: 11 in]
              n1070 = call "myRIO_BRig_RT_dataLC_ENL1_Probability_Switch_l2.vi"() -> ("output_ENL1_Probability_Switch_l2"=w1874:i32)  [unwired: 11 in]
              n1071 = call "myRIO_BRig_RT_dataLC_ENL1_Tdelay_Switch_l2.vi"() -> ("output_ENL1_Tdelay_Switch_l2"=w1875:i32)  [unwired: 11 in]
              n1072 = call "myRIO_BRig_RT_dataLC_ENL1_Count_Switch_l2.vi"() -> ("output_ENL1_Count_Switch_l2"=w1876:i32)  [unwired: 11 in]
              n1073 = call "myRIO_BRig_RT_dataLC_ENL1_delayOpt_Switch_l2.vi"() -> ("output_ENL1_delayOpt_Switch_l2"=w1877:i32)  [unwired: 11 in]
              n1074 = local read "LC_ENL1_delayOpt_Switch_l2"() -> (w1897:bool)
              n1075 = call "myRIO_BRig_RT_dataLC_ENL1_Block_NS_l2.vi"() -> ("output_ENL1_Block_NS_l2"=w1866:i32)  [unwired: 11 in]
              n1076 = call "myRIO_BRig_RT_dataLC_ENL1_OnOff_NS_l2.vi"() -> ("output_ENL1_OnOff_NS_l2"=w1867:i32)  [unwired: 11 in]
              n1077 = call "myRIO_BRig_RT_dataLC_ENL1_Probability_NS_l2.vi"() -> ("output_ENL1_Probability_NS_l2"=w1868:i32)  [unwired: 11 in]
              n1078 = call "myRIO_BRig_RT_dataLC_ENL1_Tdelay_NS_l2.vi"() -> ("output_ENL1_Tdelay_NS_l2"=w1869:i32)  [unwired: 11 in]
              n1079 = call "myRIO_BRig_RT_dataLC_ENL1_Count_NS_l2.vi"() -> ("output_ENL1_Count_NS_l2"=w1870:i32)  [unwired: 11 in]
              n1080 = call "myRIO_BRig_RT_dataLC_ENL1_delayOpt_NS_l2.vi"() -> ("output_ENL1_delayOpt_NS_l2"=w1871:i32)  [unwired: 11 in]
              n1081 = local read "LC_ENL1_Count_Switch_l2"() -> (w1909:u16)
              n1082 = local read "LC_ENL1_Probability_Switch_l2"() -> (w1911:u16)
              n1083 = local read "LC_ENL1_Block_Switch_l2"() -> (w1915:u16)
              n1084 = local read "LC_ENL1_Tdelay_Switch_l2"() -> (w1910:u16)
              n1085 = local read "LC_ENL1_OnOff_Switch_l2"() -> (w1914:bool)
              n1086 = call "myRIO_BRig_RT_dataLC_Selection_Block_Switch_l2.vi"() -> ("output_Selection_Block_Switch_l2"=w1865:i32)  [unwired: 11 in]
              n1087 = call "myRIO_BRig_RT_dataLC_Selection_OnOff_Switch_l2.vi"() -> ("output_Selection_OnOff_Switch_l2"=w1864:i32)  [unwired: 11 in]
              n1088 = call "myRIO_BRig_RT_dataLC_Selection_Probability_Switch_l2.vi"() -> ("output_Selection_Probability_Switch_l1"=w1863:i32)  [unwired: 11 in]
              n1089 = call "myRIO_BRig_RT_dataLC_Selection_Tdelay_Switch_l2.vi"() -> ("output_Selection_Tdelay_Switch_l2"=w1862:i32)  [unwired: 11 in]
              n1090 = call "myRIO_BRig_RT_dataLC_Selection_Count_Switch_l2.vi"() -> ("output_Selection_Count_Switch_l2"=w1861:i32)  [unwired: 11 in]
              n1091 = local read "LC_ENL1_OnOff_NS_l2"() -> (w1892:bool)
              n1092 = local read "LC_ENL1_Probability_NS_l2"() -> (w1890:u16)
              n1093 = local read "LC_ENL1_delayOpt_NS_l2"() -> (w1888:bool)
              n1094 = local read "LC_Sel_Probability_Switch_l2"() -> (w1881:u16)
              n1095 = local read "LC_ENL1_Tdelay_NS_l2"() -> (w1886:u16)
              n1096 = local read "LC_ENL1_Block_NS_l2"() -> (w1893:u16)
              n1097 = local read "LC_ENL1_Count_NS_l2"() -> (w1889:u16)
              n1098 = local read "LC_Sel_Tdelay_Switch_l2"() -> (w1880:u16)
              n1099 = local read "LC_Sel_OnOff_Switch_l2"() -> (w1884:bool)
              n1100 = local read "LC_Sel_Count_Switch_l2"() -> (w1879:u16)
              n1101 = local read "LC_Sel_Block_Switch_l2"() -> (w1883:u16)
              n1102 = Boolean To (0,1)(Boolean=w1897) -> (0, 1=w1898:i16)
              n1103 = Boolean To (0,1)(Boolean=w1914) -> (0, 1=w1913:i16)
              n1104 = Boolean To (0,1)(Boolean=w1892) -> (0, 1=w1895:i16)
              n1105 = To Unsigned Word Integer(number=w1898) -> (unsigned 16bit integer=w1896:u16)
              n1106 = To Unsigned Word Integer(number=w1913) -> (unsigned 16bit integer=w1912:u16)
              n1107 = Boolean To (0,1)(Boolean=w1888) -> (0, 1=w1894:i16)
              n1108 = To Unsigned Word Integer(number=w1895) -> (unsigned 16bit integer=w1891:u16)
              n1109 = Boolean To (0,1)(Boolean=w1884) -> (0, 1=w1885:i16)
              n1110 = To Unsigned Word Integer(number=w1894) -> (unsigned 16bit integer=w1887:u16)
              n1111 = To Unsigned Word Integer(number=w1885) -> (unsigned 16bit integer=w1882:u16)
              n1112 = Replace Array Subset(array=w1916, new element #1=w1915, index #1=w1872, new element #2=w1912, index #2=w1873, new element #3=w1911, index #3=w1874, new element #4=w1910, index #4=w1875, new element #5=w1909, index #5=w1876, new element #6=w1896, index #6=w1877, new element #7=w1893, index #7=w1866, new element #8=w1891, index #8=w1867, new element #9=w1890, index #9=w1868, new element #10=w1886, index #10=w1869, new element #11=w1889, index #11=w1870, new element #12=w1887, index #12=w1871, new element #13=w1883, index #13=w1865, new element #14=w1882, index #14=w1864, new element #15=w1881, index #15=w1863, new element #16=w1880, index #16=w1862, new element #17=w1879, index #17=w1861) -> (w1917:u16[])
            }
            frame "saveSettings_LC_Cue_l1" {
              # "Selection All"
              # "Count"
              # "Tdelay"
              # "Probability"
              # "OnOff"
              # "Block"
              # "delayOpt"
              # "Count"
              # "Tdelay"
              # "Probability"
              # "OnOff"
              # "Block"
              # "Cue1 All"
              # "delayOpt"
              # "Count"
              # "Tdelay"
              # "Probability"
              # "OnOff"
              # "Block"
              # "Cue1 First"
              n1113 = call "myRIO_BRig_RT_dataLC_Cue1_delayOpt_Switch_l1.vi"() -> ("output_Cue1_delayOpt_Switch_l1"=w1956:i32)  [unwired: 11 in]
              n1114 = call "myRIO_BRig_RT_dataLC_Cue1_Block_Switch_l1.vi"() -> ("output_Cue1_Block_Switch_l1"=w1979:i32)  [unwired: 11 in]
              n1115 = call "myRIO_BRig_RT_dataLC_Cue1_OnOff_Switch_l1.vi"() -> ("output_Cue1_OnOff_Switch_l1"=w1977:i32)  [unwired: 11 in]
              n1116 = call "myRIO_BRig_RT_dataLC_Cue1_Probability_Switch_l1.vi"() -> ("output_Cue1_Probability_Switch_l1"=w1973:i32)  [unwired: 11 in]
              n1117 = call "myRIO_BRig_RT_dataLC_Cue1_Tdelay_Switch_l1.vi"() -> ("output_Cue1_Tdelay_Switch_l1"=w1971:i32)  [unwired: 11 in]
              n1118 = call "myRIO_BRig_RT_dataLC_Cue1_Count_Switch_l1.vi"() -> ("output_Cue1_Count_Switch_l1"=w1969:i32)  [unwired: 11 in]
              n1119 = local read "LC_Cue1_delayOpt_Switch_l1"() -> (w1955:bool)
              n1120 = call "myRIO_BRig_RT_dataLC_Cue1_Block_NS_l1.vi"() -> ("output_Cue1_Block_NS_l1"=w1953:i32)  [unwired: 11 in]
              n1121 = call "myRIO_BRig_RT_dataLC_Cue1_OnOff_NS_l1.vi"() -> ("output_Cue1_OnOff_NS_l1"=w1952:i32)  [unwired: 11 in]
              n1122 = call "myRIO_BRig_RT_dataLC_Cue1_Probability_NS_l1.vi"() -> ("output_Cue1_l1_All_Probability"=w1951:i32)  [unwired: 11 in]
              n1123 = call "myRIO_BRig_RT_dataLC_Cue1_Tdelay_NS_l1.vi"() -> ("output_Cue1_Tdelay_NS_l1"=w1950:i32)  [unwired: 11 in]
              n1124 = call "myRIO_BRig_RT_dataLC_Cue1_Count_NS_l1.vi"() -> ("output_Cue1_Count_NS_l1"=w1949:i32)  [unwired: 11 in]
              n1125 = call "myRIO_BRig_RT_dataLC_Cue1_delayOpt_NS_l1.vi"() -> ("output_Cue1_delayOpt_NS_l1"=w1948:i32)  [unwired: 11 in]
              n1126 = local read "LC_Cue1_Count_Switch_l1"() -> (w1968:u16)
              n1127 = local read "LC_Cue1_Probability_Switch_l1"() -> (w1972:u16)
              n1128 = local read "LC_Cue1_Block_Switch_l1"() -> (w1978:u16)
              n1129 = local read "LC_Cue1_Tdelay_Switch_l1"() -> (w1970:u16)
              n1130 = local read "LC_Cue1_OnOff_Switch_l1"() -> (w1976:bool)
              n1131 = local read "LC_Cue1_OnOff_NS_l1"() -> (w1944:bool)
              n1132 = call "myRIO_BRig_RT_dataLC_Selection_Block_NS_l1.vi"() -> ("output_Selection_Block_NS_l1"=w1937:i32)  [unwired: 11 in]
              n1133 = call "myRIO_BRig_RT_dataLC_Selection_OnOff_NS_l1.vi"() -> ("output_Selection_OnOff_NS_l1"=w1936:i32)  [unwired: 11 in]
              n1134 = call "myRIO_BRig_RT_dataLC_Selection_Probability_NS_l1.vi"() -> ("output_Selection_Probability_NS_l1"=w1935:i32)  [unwired: 11 in]
              n1135 = call "myRIO_BRig_RT_dataLC_Selection_Tdelay_NS_l1.vi"() -> ("output_Selection_Tdelay_NS_l1"=w1934:i32)  [unwired: 11 in]
              n1136 = call "myRIO_BRig_RT_dataLC_Selection_Count_NS_l1.vi"() -> ("output_Selection_Count_NS_l1"=w1927:i32)  [unwired: 11 in]
              n1137 = local read "LC_Cue1_delayOpt_NS_l1"() -> (w1945:bool)
              n1138 = local read "LC_Cue1_Probability_NS_l1"() -> (w1941:u16)
              n1139 = local read "LC_Cue1_Tdelay_NS_l1"() -> (w1940:u16)
              n1140 = local read "LC_Cue1_Count_NS_l1"() -> (w1939:u16)
              n1141 = local read "LC_Cue1_Block_NS_l1"() -> (w1943:u16)
              n1142 = local read "LC_Sel_Probability_NS_l1"() -> (w1929:u16)
              n1143 = local read "LC_Sel_Tdelay_NS_l1"() -> (w1928:u16)
              n1144 = local read "LC_Sel_OnOff_NS_l1"() -> (w1931:bool)
              n1145 = local read "LC_Sel_Count_NS_l1"() -> (w1926:u16)
              n1146 = local read "LC_Sel_Block_NS_l1"() -> (w1933:u16)
              n1147 = Boolean To (0,1)(Boolean=w1955) -> (0, 1=w1957:i16)
              n1148 = Boolean To (0,1)(Boolean=w1976) -> (0, 1=w1975:i16)
              n1149 = Boolean To (0,1)(Boolean=w1944) -> (0, 1=w1947:i16)
              n1150 = To Unsigned Word Integer(number=w1957) -> (unsigned 16bit integer=w1954:u16)
              n1151 = To Unsigned Word Integer(number=w1975) -> (unsigned 16bit integer=w1974:u16)
              n1152 = To Unsigned Word Integer(number=w1947) -> (unsigned 16bit integer=w1942:u16)
              n1153 = Boolean To (0,1)(Boolean=w1945) -> (0, 1=w1946:i16)
              n1154 = Boolean To (0,1)(Boolean=w1931) -> (0, 1=w1932:i16)
              n1155 = To Unsigned Word Integer(number=w1946) -> (unsigned 16bit integer=w1938:u16)
              n1156 = To Unsigned Word Integer(number=w1932) -> (unsigned 16bit integer=w1930:u16)
              n1157 = Replace Array Subset(array=w1980, new element #1=w1978, index #1=w1979, new element #2=w1974, index #2=w1977, new element #3=w1972, index #3=w1973, new element #4=w1970, index #4=w1971, new element #5=w1968, index #5=w1969, new element #6=w1954, index #6=w1956, new element #7=w1943, index #7=w1953, new element #8=w1942, index #8=w1952, new element #9=w1941, index #9=w1951, new element #10=w1940, index #10=w1950, new element #11=w1939, index #11=w1949, new element #12=w1938, index #12=w1948, new element #13=w1933, index #13=w1937, new element #14=w1930, index #14=w1936, new element #15=w1929, index #15=w1935, new element #16=w1928, index #16=w1934, new element #17=w1926, index #17=w1927) -> (w1981:u16[])
            }
            frame "saveSettings_LC_Cue_l2" {
              # "Selection All"
              # "Count"
              # "Tdelay"
              # "Probability"
              # "OnOff"
              # "Block"
              # "delayOpt"
              # "Count"
              # "Tdelay"
              # "Probability"
              # "OnOff"
              # "Block"
              # "Cue1 All"
              # "delayOpt"
              # "Count"
              # "Tdelay"
              # "Probability"
              # "OnOff"
              # "Block"
              # "Cue1 First"
              n1158 = call "myRIO_BRig_RT_dataLC_Cue1_delayOpt_Switch_l2.vi"() -> ("output_Cue1_delayOpt_Switch_l2"=w2020:i32)  [unwired: 11 in]
              n1159 = call "myRIO_BRig_RT_dataLC_Cue1_Block_Switch_l2.vi"() -> ("output_Cue1_Block_Switch_l2"=w2043:i32)  [unwired: 11 in]
              n1160 = call "myRIO_BRig_RT_dataLC_Cue1_OnOff_Switch_l2.vi"() -> ("output_Cue1_OnOff_Switch_l2"=w2041:i32)  [unwired: 11 in]
              n1161 = call "myRIO_BRig_RT_dataLC_Cue1_Probability_Switch_l2.vi"() -> ("output_Cue1_l2_First_Probability"=w2037:i32)  [unwired: 11 in]
              n1162 = call "myRIO_BRig_RT_dataLC_Cue1_Tdelay_Switch_l2.vi"() -> ("output_Cue1_Tdelay_Switch_l2"=w2035:i32)  [unwired: 11 in]
              n1163 = call "myRIO_BRig_RT_dataLC_Cue1_Count_Switch_l2.vi"() -> ("output_Cue1_Count_Switch_l2"=w2033:i32)  [unwired: 11 in]
              n1164 = local read "LC_Cue1_delayOpt_Switch_l2"() -> (w2019:bool)
              n1165 = call "myRIO_BRig_RT_dataLC_Cue1_Block_NS_l2.vi"() -> ("output_Cue1_Block_NS_l2"=w2017:i32)  [unwired: 11 in]
              n1166 = call "myRIO_BRig_RT_dataLC_Cue1_OnOff_NS_l2.vi"() -> ("output_Cue1_OnOff_NS_l2"=w2016:i32)  [unwired: 11 in]
              n1167 = call "myRIO_BRig_RT_dataLC_Cue1_Probability_NS_l2.vi"() -> ("output_Cue1_l2_All_Probability"=w2015:i32)  [unwired: 11 in]
              n1168 = call "myRIO_BRig_RT_dataLC_Cue1_Tdelay_NS_l2.vi"() -> ("output_Cue1_Tdelay_NS_l2"=w2014:i32)  [unwired: 11 in]
              n1169 = call "myRIO_BRig_RT_dataLC_Cue1_Count_NS_l2.vi"() -> ("output_Cue1_Count_NS_l2"=w2013:i32)  [unwired: 11 in]
              n1170 = call "myRIO_BRig_RT_dataLC_Cue1_delayOpt_NS_l2.vi"() -> ("output_Cue1_delayOpt_NS_l2"=w2012:i32)  [unwired: 11 in]
              n1171 = local read "LC_Cue1_Count_Switch_l2"() -> (w2032:u16)
              n1172 = local read "LC_Cue1_Probability_Switch_l2"() -> (w2036:u16)
              n1173 = local read "LC_Cue1_Block_Switch_l2"() -> (w2042:u16)
              n1174 = local read "LC_Cue1_Tdelay_Switch_l2"() -> (w2034:u16)
              n1175 = local read "LC_Cue1_OnOff_Switch_l2"() -> (w2040:bool)
              n1176 = local read "LC_Cue1_OnOff_NS_l2"() -> (w2008:bool)
              n1177 = call "myRIO_BRig_RT_dataLC_Selection_Block_NS_l2.vi"() -> ("output_Selection_Block_NS_l2"=w1993:i32)  [unwired: 11 in]
              n1178 = call "myRIO_BRig_RT_dataLC_Selection_OnOff_NS_l2.vi"() -> ("output_Selection_OnOff_NS_l2"=w1992:i32)  [unwired: 11 in]
              n1179 = call "myRIO_BRig_RT_dataLC_Selection_Probability_NS_l2.vi"() -> ("output_Selection_Probability_NS_l2"=w1991:i32)  [unwired: 11 in]
              n1180 = call "myRIO_BRig_RT_dataLC_Selection_Tdelay_NS_l2.vi"() -> ("output_Selection_Tdelay_NS_l2"=w1990:i32)  [unwired: 11 in]
              n1181 = call "myRIO_BRig_RT_dataLC_Selection_Count_NS_l2.vi"() -> ("output_Selection_Count_NS_l2"=w1989:i32)  [unwired: 11 in]
              n1182 = local read "LC_Cue1_delayOpt_NS_l2"() -> (w2009:bool)
              n1183 = local read "LC_Cue1_Probability_NS_l2"() -> (w2005:u16)
              n1184 = local read "LC_Cue1_Tdelay_NS_l2"() -> (w2004:u16)
              n1185 = local read "LC_Cue1_Count_NS_l2"() -> (w2003:u16)
              n1186 = local read "LC_Cue1_Block_NS_l2"() -> (w2007:u16)
              n1187 = local read "LC_Sel_Probability_NS_l2"() -> (w1997:u16)
              n1188 = local read "LC_Sel_Tdelay_NS_l2"() -> (w1996:u16)
              n1189 = local read "LC_Sel_OnOff_NS_l2"() -> (w1999:bool)
              n1190 = local read "LC_Sel_Count_NS_l2"() -> (w1995:u16)
              n1191 = local read "LC_Sel_Block_NS_l2"() -> (w2001:u16)
              n1192 = Boolean To (0,1)(Boolean=w2019) -> (0, 1=w2021:i16)
              n1193 = Boolean To (0,1)(Boolean=w2040) -> (0, 1=w2039:i16)
              n1194 = Boolean To (0,1)(Boolean=w2008) -> (0, 1=w2011:i16)
              n1195 = To Unsigned Word Integer(number=w2021) -> (unsigned 16bit integer=w2018:u16)
              n1196 = To Unsigned Word Integer(number=w2039) -> (unsigned 16bit integer=w2038:u16)
              n1197 = To Unsigned Word Integer(number=w2011) -> (unsigned 16bit integer=w2006:u16)
              n1198 = Boolean To (0,1)(Boolean=w2009) -> (0, 1=w2010:i16)
              n1199 = Boolean To (0,1)(Boolean=w1999) -> (0, 1=w2000:i16)
              n1200 = To Unsigned Word Integer(number=w2010) -> (unsigned 16bit integer=w2002:u16)
              n1201 = To Unsigned Word Integer(number=w2000) -> (unsigned 16bit integer=w1998:u16)
              n1202 = Replace Array Subset(array=w2044, new element #1=w2042, index #1=w2043, new element #2=w2038, index #2=w2041, new element #3=w2036, index #3=w2037, new element #4=w2034, index #4=w2035, new element #5=w2032, index #5=w2033, new element #6=w2018, index #6=w2020, new element #7=w2007, index #7=w2017, new element #8=w2006, index #8=w2016, new element #9=w2005, index #9=w2015, new element #10=w2004, index #10=w2014, new element #11=w2003, index #11=w2013, new element #12=w2002, index #12=w2012, new element #13=w2001, index #13=w1993, new element #14=w1998, index #14=w1992, new element #15=w1997, index #15=w1991, new element #16=w1996, index #16=w1990, new element #17=w1995, index #17=w1989) -> (w2045:u16[])
            }
            frame "saveSettings6_LC_l1_Other" {
              # "Trial"
              # "Tdelay"
              # "Probability"
              # "OnOff"
              # "Block"
              # "Wrong"
              # "Trial"
              # "Tdelay"
              # "Probability"
              # "OnOff"
              # "Block"
              # "Reward"
              n1203 = call "myRIO_BRig_RT_dataLC_Wrong_Block_l1.vi"() -> ("output_Wrong_Block_l1"=w2074:i32)  [unwired: 11 in]
              n1204 = call "myRIO_BRig_RT_dataLC_Wrong_OnOff_l1.vi"() -> ("output_Wrong_OnOff_l1"=w2073:i32)  [unwired: 11 in]
              n1205 = call "myRIO_BRig_RT_dataLC_Wrong_Probability_l1.vi"() -> ("output_Wrong_Probability_l1"=w2072:i32)  [unwired: 11 in]
              n1206 = call "myRIO_BRig_RT_dataLC_Wrong_Tdelay_l1.vi"() -> ("output_Wrong_Tdelay_l1"=w2071:i32)  [unwired: 11 in]
              n1207 = call "myRIO_BRig_RT_dataLC_Wrong_Trial_l1.vi"() -> ("output_Wrong_Trial_l1"=w2070:i32)  [unwired: 11 in]
              n1208 = call "myRIO_BRig_RT_dataLC_Reward_Block_l1.vi"() -> ("output_Reward_Block_l1"=w2086:i32)  [unwired: 11 in]
              n1209 = call "myRIO_BRig_RT_dataLC_Reward_OnOff_l1.vi"() -> ("output_Reward_OnOff_l1"=w2084:i32)  [unwired: 11 in]
              n1210 = call "myRIO_BRig_RT_dataLC_Reward_Probability_l1.vi"() -> ("output_Reward_Probability_l1"=w2080:i32)  [unwired: 11 in]
              n1211 = call "myRIO_BRig_RT_dataLC_Reward_Tdelay_l1.vi"() -> ("output_Reward_Tdelay_l1"=w2078:i32)  [unwired: 11 in]
              n1212 = call "myRIO_BRig_RT_dataLC_Reward_Trial_l1.vi"() -> ("output_Reward_Trial_l1"=w2076:i32)  [unwired: 11 in]
              n1213 = local read "LC_Wrong_OnOff_l1"() -> (w2068:bool)
              n1214 = local read "LC_Wrong_Probability_l1"() -> (w2065:u16)
              n1215 = local read "LC_Wrong_Block_l1"() -> (w2067:u16)
              n1216 = local read "LC_Wrong_Tdelay_l1"() -> (w2064:u16)
              n1217 = local read "LC_Wrong_Trial_l1"() -> (w2063:u16)
              n1218 = local read "LC_Reward_Probability_l1"() -> (w2079:u16)
              n1219 = local read "LC_Reward_Block_l1"() -> (w2085:u16)
              n1220 = local read "LC_Reward_Tdelay_l1"() -> (w2077:u16)
              n1221 = local read "LC_Reward_OnOff_l1"() -> (w2083:bool)
              n1222 = local read "LC_Reward_Trial_l1"() -> (w2075:u16)
              n1223 = Boolean To (0,1)(Boolean=w2068) -> (0, 1=w2069:i16)
              n1224 = Boolean To (0,1)(Boolean=w2083) -> (0, 1=w2082:i16)
              n1225 = To Unsigned Word Integer(number=w2069) -> (unsigned 16bit integer=w2066:u16)
              n1226 = To Unsigned Word Integer(number=w2082) -> (unsigned 16bit integer=w2081:u16)
              n1227 = Replace Array Subset(array=w2087, new element #1=w2085, index #1=w2086, new element #2=w2081, index #2=w2084, new element #3=w2079, index #3=w2080, new element #4=w2077, index #4=w2078, new element #5=w2075, index #5=w2076, new element #6=w2067, index #6=w2074, new element #7=w2066, index #7=w2073, new element #8=w2065, index #8=w2072, new element #9=w2064, index #9=w2071, new element #10=w2063, index #10=w2070) -> (w2088:u16[])
            }
            frame "SaveSettings6_LC_l2_Other" {
              # "Trial"
              # "Tdelay"
              # "Probability"
              # "OnOff"
              # "Block"
              # "Wrong"
              # "Trial"
              # "Tdelay"
              # "Probability"
              # "OnOff"
              # "Block"
              # "Reward"
              n1228 = call "myRIO_BRig_RT_dataLC_Wrong_Block_l2.vi"() -> ("output_Wrong_Block_l2"=w2097:i32)  [unwired: 11 in]
              n1229 = call "myRIO_BRig_RT_dataLC_Wrong_OnOff_l2.vi"() -> ("output_Wrong_OnOff_l2"=w2098:i32)  [unwired: 11 in]
              n1230 = call "myRIO_BRig_RT_dataLC_Wrong_Probability_l2.vi"() -> ("output_Wrong_Probability_l2"=w2099:i32)  [unwired: 11 in]
              n1231 = call "myRIO_BRig_RT_dataLC_Wrong_Tdelay_l2.vi"() -> ("output_Wrong_Tdelay_l2"=w2100:i32)  [unwired: 11 in]
              n1232 = call "myRIO_BRig_RT_dataLC_Wrong_Trial_l2.vi"() -> ("output_Wrong_Trial_l2"=w2101:i32)  [unwired: 11 in]
              n1233 = call "myRIO_BRig_RT_dataLC_Reward_Block_l2.vi"() -> ("output_Reward_Block_l2"=w2102:i32)  [unwired: 11 in]
              n1234 = call "myRIO_BRig_RT_dataLC_Reward_OnOff_l2.vi"() -> ("output_Reward_OnOff_l2"=w2103:i32)  [unwired: 11 in]
              n1235 = call "myRIO_BRig_RT_dataLC_Reward_Probability_l2.vi"() -> ("output_Reward_Probability_l2"=w2104:i32)  [unwired: 11 in]
              n1236 = call "myRIO_BRig_RT_dataLC_Reward_Tdelay_l2.vi"() -> ("output_Reward_Tdelay_l2"=w2105:i32)  [unwired: 11 in]
              n1237 = call "myRIO_BRig_RT_dataLC_Reward_Trial_l2.vi"() -> ("output_Reward_Trial_l2"=w2106:i32)  [unwired: 11 in]
              n1238 = local read "LC_Wrong_OnOff_l2"() -> (w2122:bool)
              n1239 = local read "LC_Wrong_Probability_l2"() -> (w2119:u16)
              n1240 = local read "LC_Wrong_Block_l2"() -> (w2121:u16)
              n1241 = local read "LC_Wrong_Tdelay_l2"() -> (w2118:u16)
              n1242 = local read "LC_Wrong_Trial_l2"() -> (w2117:u16)
              n1243 = local read "LC_Reward_Probability_l2"() -> (w2126:u16)
              n1244 = local read "LC_Reward_Block_l2"() -> (w2130:u16)
              n1245 = local read "LC_Reward_Tdelay_l2"() -> (w2125:u16)
              n1246 = local read "LC_Reward_OnOff_l2"() -> (w2129:bool)
              n1247 = local read "LC_Reward_Trial_l2"() -> (w2124:u16)
              n1248 = Boolean To (0,1)(Boolean=w2122) -> (0, 1=w2123:i16)
              n1249 = Boolean To (0,1)(Boolean=w2129) -> (0, 1=w2128:i16)
              n1250 = To Unsigned Word Integer(number=w2123) -> (unsigned 16bit integer=w2120:u16)
              n1251 = To Unsigned Word Integer(number=w2128) -> (unsigned 16bit integer=w2127:u16)
              n1252 = Replace Array Subset(array=w2131, new element #1=w2130, index #1=w2102, new element #2=w2127, index #2=w2103, new element #3=w2126, index #3=w2104, new element #4=w2125, index #4=w2105, new element #5=w2124, index #5=w2106, new element #6=w2121, index #6=w2097, new element #7=w2120, index #7=w2098, new element #8=w2119, index #8=w2099, new element #9=w2118, index #9=w2100, new element #10=w2117, index #10=w2101) -> (w2132:u16[])
            }
            frame "setSettings_Audio" {
              # "amp_L"
              # "amp_R"
              # "freq_L"
              # "freq_R"
              n1253 = call "myRIO_BRig_RT_dataExp_Audio_amp__L.vi"() -> ("output_Audio_amp__L"=w2157:i32)  [unwired: 11 in]
              n1254 = call "myRIO_BRig_RT_dataExp_Audio_amp__R.vi"() -> ("output_Audio_amp__R"=w2156:i32)  [unwired: 11 in]
              n1255 = call "myRIO_BRig_RT_dataExp_Audio_freq__L.vi"() -> ("output_Audio_freq__L"=w2155:i32)  [unwired: 11 in]
              n1256 = call "myRIO_BRig_RT_dataExp_Audio_freq__R.vi"() -> ("output_Audio_freq__R"=w2154:i32)  [unwired: 11 in]
              n1257 = Index Array(array=w2153, index #1=w2157, index #2=w2156, index #3=w2155, index #4=w2154) -> (element #1=w2152:u16, element #2=w2151:u16, element #3=w2144:u16, element #4=w2142:u16)
              n1258 = To Unsigned Byte Integer(number=w2144) -> (unsigned 8bit integer=w2143:u8)
              n1259 = To Unsigned Byte Integer(number=w2142) -> (unsigned 8bit integer=w2141:u8)
            }
            frame "setSettings_Laser" {
              w2179 = u32 0 ("laser2_selRew_Ndelay")
              # "tDelay"
              # "Wrong l1"
              # "Reward l1"
              n1260 = local read "Laser_Tpeak_l1"() -> (w2193:dbl)
              n1261 = local read "Laser_Tshutter_l1"() -> (w2191:dbl)
              n1262 = local read "Laser_Freq_l1"() -> (w2192:dbl)
              n1263 = local read "Laser_duration_l1"() -> (w2188:u16)
              n1264 = local read "Laser_Tpeak_l2"() -> (w2187:dbl)
              n1265 = local read "Laser_Tshutter_l2"() -> (w2185:dbl)
              n1266 = local read "Laser_Freq_l2"() -> (w2186:dbl)
              n1267 = local read "Laser_duration_l2"() -> (w2184:u16)
              n1268 = local read "CueLed_Freq"() -> (w2171:dbl)
              n1269 = local read "CueLed_duration"() -> (w2170:u16)
              n1270 = local read "CueLed_Tpeak"() -> (w2172:dbl)
              n1271 = call "myRIO_BRig_RT_dataLC_Reward_Tdelay_l1.vi"() -> ("output_Reward_Tdelay_l1"=w2206:i32)  [unwired: 11 in]
              n1272 = call "myRIO_BRig_RT_dataLC_Wrong_Tdelay_l1.vi"() -> ("output_Wrong_Tdelay_l1"=w2207:i32)  [unwired: 11 in]
              n1273 = local read "FPGA_count2ms"() -> (w2173:dbl)
              n1274 = Index Array(array=w2203, index #1=w2206, index #2=w2207) -> (element #1=w2205:u16, element #2=w2204:u16)
              n1275 = To Double Precision Float(number=w2205) -> (double precision float=w2200:dbl)
              n1276 = To Double Precision Float(number=w2204) -> (double precision float=w2197:dbl)
              n1277 = To Unsigned Word Integer(number=w2173) -> (unsigned 16bit integer=w2194:u16)
              n1278 = call "myRIO_BRig_RT__calc_laser_FPGA_N.vi"("input_FPGA_count2ms"=w2173, "input_Tpeak"=w2193, "input_Freq"=w2192, "input_Tshutter"=w2191, "input_duration"=w2188) -> ("output_laser_Npeak"=w2178:u32, "output_laser_Nvalley"=w2177:u32, "output_laser_Nshutter"=w2176:u32, "output_laser_Nduration"=w2190:u32, "output_laser_Tduration"=w2189:u16)  [unwired: 6 in]
              n1279 = Multiply(x=w2173, y=w2200) -> (x*y=w2201:dbl)
              n1280 = Multiply(x=w2173, y=w2197) -> (x*y=w2198:dbl)
              n1281 = call "myRIO_BRig_RT__calc_laser_FPGA_N__CueLed.vi"("input_FPGA_count2ms"=w2173, "input_Tpeak"=w2172, "input_Freq"=w2171, "input_duration"=w2170) -> ("output_laser_Npeak"=w2169:u32, "output_laser_Nvalley"=w2168:u32, "output_laser_Tduration"=w2166:u16)  [unwired: 9 in]
              n1282 = call "myRIO_BRig_RT__calc_laser_FPGA_N.vi"("input_FPGA_count2ms"=w2173, "input_Tpeak"=w2187, "input_Freq"=w2186, "input_Tshutter"=w2185, "input_duration"=w2184) -> ("output_laser_Npeak"=w2183:u32, "output_laser_Nvalley"=w2182:u32, "output_laser_Nshutter"=w2181:u32, "output_laser_Nduration"=w2180:u32, "output_laser_Tduration"=w2174:u16)  [unwired: 6 in]
              n1283 = Round Toward +Infinity(x=w2201) -> (ceil(x): smallest int >= x=w2202:dbl)
              n1284 = Round Toward +Infinity(x=w2198) -> (ceil(x): smallest int >= x=w2199:dbl)
              n1285 = To Unsigned Long Integer(number=w2202) -> (unsigned 32bit integer=w2196:u32)
              n1286 = To Unsigned Long Integer(number=w2199) -> (unsigned 32bit integer=w2195:u32)
              n1287 = xnode "Read/Write Control"("FPGA VI Reference In"=w2210, "error in"=w2211, "LC_nPeak_l1"=w2178, "LC_nValley_l1"=w2177, "LC_nShutter_l1"=w2176, "LR_reward_nDelay_l1"=w2196, "LR_wrong_nDelay_l1"=w2195, "LR_reward_nTotal_l1"=w2190, "LR_wrong_nTotal_l1"=w2190, "k1__counter_per_ms"=w2194, "LC_nPeak_l2"=w2183, "LC_nValley_l2"=w2182, "LC_nShutter_l2"=w2181, "LR_reward_nDelay_l2"=w2179, "LR_wrong_nDelay_l2"=w2179, "LR_reward_nTotal_l2"=w2180, "LR_wrong_nTotal_l2"=w2180, "CueLed_nPeak"=w2169, "CueLed_nValley"=w2168) -> ("error out"=→"error out":errorcluster)  [unwired: 1 out]
              n1288 = call "myRIO_BRig_RT_dataCurrent_laser1_pulse_duration.vi"() -> ("output_laser1_pulse_duration"=w2208:i32)  [unwired: 11 in]
              n1289 = call "myRIO_BRig_RT_dataCurrent_laser2_pulse_duration.vi"() -> ("output_laser2_pulse_duration"=w2175:i32)  [unwired: 11 in]
              n1290 = call "myRIO_BRig_RT_dataCurrent_CueLed_pulse_duration.vi"() -> ("output_CueLed_pulse_duration"=w2167:i32)  [unwired: 11 in]
              n1291 = Replace Array Subset(array=w2203, new element #1=w2189, index #1=w2208, new element #2=w2174, index #2=w2175, new element #3=w2166, index #3=w2167) -> (w2209:u16[])
            }
            frame "initBlock" {
              n1292 = call "myRIO_Brig_RT__Case_Exp_State_initBlock.vi"("input_spout"=w2255, "input_dataExp"=w2253, "input_dataCurrent"=w2254) -> ("output_spout"=w2233:enum16{"Left", "Right"}, "output_state"=w2256:T2, "output_dataExp"=w2252:u16[], "output_dataCurrent"=w2238:u16[], "output_TpB_target"=→"TpB_target":u16)  [unwired: 4 in]
              "cSpout" <- w2233
              n1293 = call "myRIO_BRig_RT_dataCurrent_iBlock.vi"() -> ("output_iBlock"=w2237:i32)  [unwired: 11 in]
              n1294 = Index Array(array=w2238, index=w2237) -> (element=w2231:u16)
              "iBlock" <- w2231
            }
            frame "initBlock2" {
              n1295 = local write "nRewards_cur"(u16 0 ("nRewards_cur")) -> ()
              n1296 = call "myRIO_BRig_RT__Case_Exp_State_initBlock2.vi"("input_spout"=w2264, "input_dataBlock"=w2265, "input_dataCurrent"=w2263) -> ("idxDataBlock"=w2260:i32, "output_dataBlock"=w2262:u16[][])  [unwired: 7 in]
            }
            frame "initTrial" {
              n1297 = call "myRIO_Brig_RT__Case_Exp_State_initTrial.vi"("input_spout"=w2278, "input_dataExp"=w2299, "input_dataCurrent"=w2300) -> ("output_state"=w2301:T2, "output_dataExp"=w2298:u16[], "output_dataCurrent"=w2288:u16[])  [unwired: 6 in]
              n1298 = call "myRIO_BRig_RT_dataCurrent_iTrial.vi"() -> ("output_iTrial"=w2287:i32)  [unwired: 11 in]
              n1299 = call "myRIO_BRig_RT_dataCurrent_SolenoidReward.vi"() -> ("output_SolenoidReward"=w2283:i32)  [unwired: 11 in]
              n1300 = Index Array(array=w2288, index #1=w2287, index #2=w2283) -> (element #1=w2279:u16, element #2=w2282:u16)
              "iTrial" <- w2279
              n1301 = Not Equal To 0?(x=w2282) -> (x != 0?=→"SolenoidReward":bool)
            }
            frame "initTrial2" {
              # "trialUntilReward"
              n1302 = call "myRIO_BRig_RT__Case_Exp_subState_LC__initTrial__v3.vi"("input_dataCurrent"=w2314, "input_dataLC"=w2313, "input_spout"=w2315, "input_dataTrial"=w2317) -> ("output_dataTrial"=w2316:u16[][], "output_LR_Wrong_Laser_l2"=w2305:bool, "output_LR_Reward_Laser_l2"=w2306:bool, "output_LR_Reward_Event_l1"=w2312:bool, "output_LR_Wrong_Event_l1"=w2311:bool, "output_LR_Reward_Laser_l1"=w2310:bool, "output_LR_Wrong_Laser_l1"=w2309:bool, "output_LR_Reward_Event_l2"=w2308:bool, "output_LR_Wrong_Event_l2"=w2307:bool)  [unwired: 7 in]
              n1303 = call "myRIO_BRig_RT_dataExp_ItrialUntilReward.vi"() -> ("output_I_trialUntilReward"=w2321:i32)  [unwired: 11 in]
              n1304 = Index Array(array=w2322, index=w2321) -> (element=w2320:u16)
              n1305 = Equal?(x=w2315, y=enum16{"Left", "Right"}."Right") -> (x = y?=w2319:bool)
              n1306 = Not Equal To 0?(x=w2320) -> (x != 0?=w2318:bool)
              n1307 = xnode "Read/Write Control"("FPGA VI Reference In"=w2336, "error in"=w2335, "SelectionState"=FALSE, "Left(F)_or_Right(T)"=w2319, "ignoreWrong"=w2318, "LR_reward_Event_l1"=w2312, "LR_wrong_Event_l1"=w2311, "LR_reward_Laser_l1"=w2310, "LR_wrong_Laser_l1"=w2309, "LR_reward_Event_l2"=w2308, "LR_wrong_Event_l2"=w2307, "LR_reward_Laser_l2"=w2306, "LR_wrong_laser_l2"=w2305) -> ("error out"=→"error_initTrial":errorcluster)  [unwired: 1 out]
            }
            frame "initTrial3" {
              n1308 = call "myRIO_BRig_RT_arrTrig_init.vi"() -> ("output_arrTrig"=w2342:bool[])  [unwired: 11 in]
              n1309 = call "myRIO_BRig_RT__Case_Exp_State_initTrial_dataTrial.vi"("input_spout"=w2352, "input_dataCurrent"=w2353, "input_dataExp"=w2351, "input_dataTrial"=w2355) -> ("output_dataTrial"=w2354:u16[][], "output_laserPower_l1"=w2348:u16)  [unwired: 5 in, 1 out]
              n1310 = To Double Precision Float(number=w2348) -> (double precision float=w2350:dbl)
              n1311 = Divide(x=w2350, y=100.0 ("x")) -> (x/y=w2344:dbl)
              "output_PortA" <- w2344
              n1312 = call "myRIO__convert__Voltage_to_FPGAvalue.vi"("input_voltage"=w2344) -> ("output_PortC"=w2343:i16)  [unwired: 9 in, 1 out]
              n1313 = xnode "Read/Write Control"("FPGA VI Reference In"=w2347, "error in"=w2346, "AnaOut_0"=w2343) -> ("error out"=→"error out 4":errorcluster)  [unwired: 1 out]
            }
            frame "initTrial4" {
              n1314 = call "myRIO_BRig_RT_dataCurrent_idxDataTrial.vi"() -> ("output_idxDataTrial"=w2381:i32)  [unwired: 11 in]
              n1315 = call "myRIO_BRig_RT_dataTrial_activeRecording.vi"() -> ("output_activeRecording"=w2378:i32)  [unwired: 11 in]
              n1316 = Index Array(array=w2383, index=w2381) -> (element=w2380:u16)
              n1317 = Boolean To (0,1)(Boolean="Recording") -> (0, 1=w2377:i16)
              n1318 = To Long Integer(number=w2380) -> (32bit integer=w2379:i32)
              n1319 = To Unsigned Word Integer(number=w2377) -> (unsigned 16bit integer=w2376:u16)
              n1320 = Replace Array Subset(array=w2382, new element=w2376, index (row)=w2379, index (col)=w2378) -> (w2375:u16[][])
            }
            frame "initTrial_LC_ENL1" {
              n1321 = call "myRIO_BRig_RT__Case_Exp_State_initTrial_LC_ENL1__v3.vi"("input_dataTrial"=w2405, "input_spout"=w2408, "input_arrTrig"=w2402, "input_dataBlock"=w2403, "input_dataLC"=w2409, "input_dataCurrent"=w2407) -> ("output_arrTrig"=w2401:bool[], "output_dataTrial"=w2404:u16[][], "output_dataCurrent"=w2406:u16[])  [unwired: 3 in]
            }
            frame "initTrial_LC_Cue1" {
              n1322 = call "myRIO_BRig_RT__Case_Exp_State_initTrial_LC_Cue1__v3.vi"("input_dataTrial"=w2428, "input_spout"=w2431, "input_arrTrig"=w2425, "input_dataBlock"=w2426, "input_dataLC"=w2432, "input_dataCurrent"=w2430) -> ("output_arrTrig"=w2424:bool[], "output_dataTrial"=w2427:u16[][], "output_dataCurrent"=w2429:u16[])  [unwired: 3 in]
            }
            frame "initTrial_LC_Cue1_2" {
              w2460 = TRUE ("Recording")
              n1323 = local read "Cue1Param_AudioLed_Probability_Switch"() -> (w2453:u16)
              n1324 = local read "Cue1Param_AudioLed_Count_Switch"() -> (w2452:u16)
              n1325 = local read "Cue1Param_AudioLed_Probability_NS"() -> (w2450:u16)
              n1326 = local read "Cue1Param_AudioLed_Count_NS"() -> (w2449:u16)
              n1327 = local read "Cue1Param_CueType_Switch"() -> (w2454:u16)
              n1328 = local read "Cue1Param_CueType_NS"() -> (w2451:u16)
              n1329 = call "myRIO_BRig_RT__Case_Exp_State_initTrial_LC_Cue1_2.vi"("input_CueType_Switch"=w2454, "input_Probability_Switch"=w2453, "input_Count_Switch"=w2452, "input_CueType_NS"=w2451, "input_Probability_NS"=w2450, "input_Count_NS"=w2449, "input_spout"=w2448, "input_dataBlock"=w2447, "input_dataCurrent"=w2458, "input_arrTrig"=w2456) -> ("output_dataCurrent"=w2457:u16[], "output_arrTrig"=w2455:bool[])  [unwired: 8 in]
            }
            frame "initTrial_LC_Sel" {
              n1330 = call "myRIO_BRig_RT__Case_Exp_State_initTrial_LC_Sel__v3.vi"("input_dataTrial"=w2482, "input_spout"=w2485, "input_arrTrig"=w2477, "input_dataBlock"=w2480, "input_dataLC"=w2486, "input_dataCurrent"=w2484) -> ("output_arrTrig"=w2476:bool[], "output_dataTrial"=w2481:u16[][], "output_dataCurrent"=w2483:u16[])  [unwired: 3 in]
              n1331 = local read "Recording"() -> (w2479:bool)
            }
            frame "ENL1_pre" {
              # "ENL1_n"
              # "Tcycle"
              # "counter"
              n1332 = call "myRIO_BRig_RT_dataCurrent_Tcycle_generic.vi"() -> ("output_Tcycle_generic"=w2529:i32)  [unwired: 11 in]
              n1333 = call "myRIO_BRig_RT_dataCurrent_count_generic.vi"() -> ("output_count_generic"=w2531:i32)  [unwired: 11 in]
              n1334 = call "myRIO_BRig_RT_dataCurrent_Tcycle_ENL.vi"() -> ("output_ENL"=w2528:i32)  [unwired: 11 in]
              n1335 = call "myRIO_BRig_RT_dataCurrent_nENL1.vi"() -> ("output_nENL1"=w2506:i32)  [unwired: 11 in]
              n1336 = Index Array(array=w2522, index #1=w2528, index #2=w2506) -> (element #1=w2527:u16, element #2=w2505:u16)
              n1337 = Increment(x=w2505) -> (x+1=w2504:u16)
              n1338 = Replace Array Subset(array=w2522, new element #1=u16 0 ("new element/subarray"), index #1=w2531, new element #2=w2527, index #2=w2529, new element #3=w2504, index #3=w2506) -> (w2526:u16[])
              n1339 = Select(t=myRIO_BRig_RT__Case_Exp_stateList."ENL1Penalty_pre" ("Enum"), s=w2510, f=myRIO_BRig_RT__Case_Exp_stateList."ENL1" ("Enum")) -> (s? t:f=w2507:T2)
            }
            frame "ENL1" {
              n1340 = call "myRIO_BRig_RT__Case_Exp_State_ENL1__v3.vi"("I_lick"=w2542, "input_arrTrig"=w2538, "input_state"=w2546, "input_dataCurrent"=w2545) -> ("output_l1_laserOn"=w2536:bool, "output_l1_laserEvent"=w2537:bool, "output_state"=w2543:T2, "output_dataCurrent"=w2544:u16[], "output_l2_laserEvent"=w2535:bool, "output_l2_laserOn"=w2534:bool)  [unwired: 2 in]
            }
            frame "ENL1Penalty_pre" {
              # "Tcycle"
              # "counter"
              n1341 = call "myRIO_BRig_RT_dataCurrent_Tcycle_generic.vi"() -> ("output_Tcycle_generic"=w2583:i32)  [unwired: 11 in]
              n1342 = call "myRIO_BRig_RT_dataCurrent_count_generic.vi"() -> ("output_count_generic"=w2585:i32)  [unwired: 11 in]
              n1343 = call "myRIO_BRig_RT_dataExp_ENL_penalty.vi"() -> ("output_ENL_penalty"=w2578:i32)  [unwired: 11 in]
              n1344 = Index Array(array=w2579, index=w2578) -> (element=w2582:u16)
              n1345 = Replace Array Subset(array=w2580, new element #1=u16 0 ("new element/subarray"), index #1=w2585, new element #2=w2582, index #2=w2583) -> (w2581:u16[])
            }
            frame "ENL1Penalty" {
              n1346 = call "myRIO_BRig_RT__Case_Exp_State_ENL1Penalty.vi"("input_state"=w2605, "input_dataCurrent"=w2609) -> ("output_state"=w2606:T2, "output_dataCurrent"=w2608:u16[])  [unwired: 8 in]
            }
            frame "ENL2_pre" {
            }
            frame "ENL2" {
            }
            frame "ENL2Penalty_pre" {
            }
            frame "ENL2Penalty" {
            }
            frame "Cue1_pre" {
              # "Cue1_n"
              # "Tcycle_Cue1"
              # "0 = L, 1 = R, 2 = both"
              # "sp_R"
              # "sp_L"
              # "Tcycle"
              # "counter"
              n1347 = call "myRIO_BRig_RT_arrTrig_Cue1_CueType_AudioLed.vi"() -> ("output_arrTrig_Cue1_CueType_AudioLed"=w2696:i32)  [unwired: 11 in]
              n1348 = Index Array(array=w2697, index=w2696) -> (element=w2695:bool)
              n1349 = Equal?(x=w2722, y=enum16{"Left", "Right"}."Left") -> (x = y?=w2721:bool)
              n1350 = call "myRIO_BRig_RT_dataExp_Audio_sp__L.vi"() -> ("output_Audio_sp__L"=w2720:i32)  [unwired: 11 in]
              n1351 = call "myRIO_BRig_RT_dataExp_Audio_sp__R.vi"() -> ("output_Audio_sp__R"=w2719:i32)  [unwired: 11 in]
              n1352 = call "myRIO_BRig_RT_dataCurrent_Tcycle_generic.vi"() -> ("output_Tcycle_generic"=w2732:i32)  [unwired: 11 in]
              n1353 = call "myRIO_BRig_RT_dataCurrent_count_generic.vi"() -> ("output_count_generic"=w2734:i32)  [unwired: 11 in]
              n1354 = Not(x=w2695) -> (.not. x?=w2690:bool)
              n1355 = Select(t=w2720, s=w2721, f=w2719) -> (s? t:f=w2718:i32)
              n1356 = call "myRIO_BRig_RT_dataCurrent_nCue1.vi"() -> ("output_nCue1"=w2700:i32)  [unwired: 11 in]
              n1357 = call "myRIO_BRig_RT_dataCurrent_Tcycle_cue.vi"() -> ("output_Tcycle_cue"=w2707:i32)  [unwired: 11 in]
              n1358 = Index Array(array=w2724, index=w2718) -> (element=w2716:u16)
              n1359 = Index Array(array=w2708, index #1=w2707, index #2=w2700) -> (element #1=w2709:u16, element #2=w2702:u16)
              n1360 = Increment(x=w2702) -> (x+1=w2701:u16)
              n1361 = Not Equal To 0?(x=w2716) -> (x != 0?=w2692:bool)
              n1362 = Not Equal?(x=w2716, y=u16 1) -> (x != y?=w2694:bool)
              n1363 = Replace Array Subset(array=w2708, new element #1=u16 0 ("new element/subarray"), index #1=w2734, new element #2=w2709, index #2=w2732, new element #3=w2701, index #3=w2700) -> (w2731:u16[])
              n1364 = Select(t=myRIO_BRig_RT__Case_Exp_stateList."Cue1Penalty_pre" ("Enum"), s=w2704, f=myRIO_BRig_RT__Case_Exp_stateList."Cue1" ("Enum")) -> (s? t:f=w2705:T2)
              n1365 = And(x=w2692, y=w2690) -> (x .and. y?=w2691:bool)
              n1366 = And(x=w2694, y=w2690) -> (x .and. y?=w2693:bool)
            }
            frame "Cue1" {
              n1367 = call "myRIO_BRig_RT__Case_Exp_State_Cue1__v3.vi"("I_lick"=w2746, "input_arrTrig"=w2742, "input_state"=w2748, "input_dataCurrent"=w2766) -> ("output_l1_laserOn"=w2740:bool, "output_l1_laserEvent"=w2741:bool, "output_state"=w2747:T2, "output_dataCurrent"=w2765:u16[], "output_l2_laserEvent"=w2739:bool, "output_CueLed_Event"=w2737:bool, "output_l2_laserOn"=w2738:bool)  [unwired: 1 in]
              n1368 = Equal?(x=myRIO_BRig_RT__Case_Exp_stateList."Selection_pre", y=w2747) -> (x = y?=w2751:bool)
              n1369 = xnode "Read/Write Control"("FPGA VI Reference In"=w2750, "error in"=w2749, "SelectionState"=w2751) -> ()  [unwired: 2 out]
            }
            frame "Cue1Penalty_pre" {
              # "Tcycle"
              # "counter"
              n1370 = call "myRIO_BRig_RT_dataCurrent_Tcycle_generic.vi"() -> ("output_Tcycle_generic"=w2794:i32)  [unwired: 11 in]
              n1371 = call "myRIO_BRig_RT_dataCurrent_count_generic.vi"() -> ("output_count_generic"=w2796:i32)  [unwired: 11 in]
              n1372 = call "myRIO_BRig_RT_dataExp_Tcycle_CuePenalty.vi"() -> ("output_Tcycle_CuePenalty"=w2793:i32)  [unwired: 11 in]
              n1373 = Index Array(array=w2788, index=w2793) -> (element=w2792:u16)
              n1374 = Replace Array Subset(array=w2790, new element #1=u16 0 ("new element/subarray"), index #1=w2796, new element #2=w2792, index #2=w2794) -> (w2789:u16[])
            }
            frame "Cue1Penalty" {
              n1375 = call "myRIO_BRig_RT__Case_Exp_State_Cue1Penalty.vi"("input_state"=w2819, "input_dataCurrent"=w2820) -> ("output_state"=w2817:T2, "output_dataCurrent"=w2818:u16[])  [unwired: 8 in]
            }
            frame "Cue2_pre" {
              n1376 = call "myRIO_BRig_RT__Case_Exp_subState_LC__Cue2.vi"("input_spout"=w2837, "input_dataCurrent"=w2838, "input_dataLC"=w2836) -> ()  [unwired: 6 in, 2 out]
            }
            frame "Cue2" {
            }
            frame "Cue2Penalty_pre" {
            }
            frame "Cue2Penalty" {
            }
            frame "Selection_pre" {
              # "Tcycle"
              # "counter"
              n1377 = call "myRIO_BRig_RT_arrTrig_Select_laserEvent_l1.vi"() -> ("output_arrTrig_Select_laserEvent_l1"=w2913:i32)  [unwired: 11 in]
              n1378 = call "myRIO_BRig_RT_arrTrig_Select_laserOn_l1.vi"() -> ("output_arrTrig_Select_laserOn_l1"=w2912:i32)  [unwired: 11 in]
              n1379 = call "myRIO_BRig_RT_arrTrig_Select_laserEvent_l2.vi"() -> ("output_arrTrig_Select_laserEvent_l2"=w2911:i32)  [unwired: 11 in]
              n1380 = call "myRIO_BRig_RT_arrTrig_Select_laserOn_l2.vi"() -> ("output_arrTrig_Select_laserOn_l2"=w2910:i32)  [unwired: 11 in]
              n1381 = call "myRIO_BRig_RT_dataCurrent_laser1_tSel_start.vi"() -> ("output_laser1_tSel_start"=w2920:i32)  [unwired: 11 in]
              n1382 = xnode "Read/Write Control"("FPGA VI Reference In"=w2930, "error in"=w2931) -> ("error out"=→"error_Selection_pre":errorcluster, "SelectReward"=w2924:bool, "SelectWrong"=w2925:bool)  [unwired: 1 out]
              n1383 = call "myRIO_BRig_RT_dataExp_Tcycle_Selection.vi"() -> ("output_Tcycle_Selection"=w2950:i32)  [unwired: 11 in]
              n1384 = call "myRIO_BRig_RT_dataCurrent_Tcycle_generic.vi"() -> ("output_Tcycle_generic"=w2951:i32)  [unwired: 11 in]
              n1385 = call "myRIO_BRig_RT_dataCurrent_count_generic.vi"() -> ("output_count_generic"=w2953:i32)  [unwired: 11 in]
              n1386 = Index Array(array=w2921, index=w2920) -> (element=w2919:u16)
              n1387 = Index Array(array=w2900, index #1=w2913, index #2=w2912, index #3=w2911, index #4=w2910) -> (element #1=w2908:bool, element #2=w2907:bool, element #3=w2906:bool, element #4=w2905:bool)
              n1388 = Index Array(array=w2947, index=w2950) -> (element=w2949:u16)
              n1389 = Equal To 0?(x=w2919) -> (x = 0?=w2914:bool)
              n1390 = Replace Array Subset(array=w2921, new element #1=u16 0 ("new element/subarray"), index #1=w2953, new element #2=w2949, index #2=w2951) -> (w2948:u16[])
              n1391 = Or(x=w2924, y=w2925) -> (x .or. y?=w2917:bool)
              n1392 = Not(x=w2917) -> (.not. x?=w2915:bool)
              n1393 = And(x=w2915, y=w2914) -> (x .and. y?=w2909:bool)
              n1394 = And(x=w2909, y=w2908) -> (x .and. y?=w2904:bool)
              n1395 = And(x=w2909, y=w2907) -> (x .and. y?=w2903:bool)
              n1396 = And(x=w2909, y=w2906) -> (x .and. y?=w2902:bool)
              n1397 = And(x=w2909, y=w2905) -> (x .and. y?=w2901:bool)
              n1398 = Select(t=myRIO_BRig_RT__Case_Exp_stateList."SelectReward_pre" ("Enum"), s=w2924, f=myRIO_BRig_RT__Case_Exp_stateList."SelectWrong_pre" ("Enum")) -> (s? t:f=w2929:T2)
              n1399 = Select(t=w2929, s=w2917, f=myRIO_BRig_RT__Case_Exp_stateList."Selection" ("Enum")) -> (s? t:f=w2926:T2)
            }
            frame "Selection" {
              n1400 = xnode "Read/Write Control"("FPGA VI Reference In"=w2970, "error in"=w2969) -> ("error out"=→"error_Selection":errorcluster, "SelectReward"=w2961:bool, "SelectWrong"=w2960:bool)  [unwired: 1 out]
              n1401 = call "myRIO_BRig_RT__Case_Exp_State_Selection__v2.vi"("input_dataCurrent"=w2965, "input_state"=w2963, "input_FPGA_SelectReward"=w2961, "input_FPGA_SelectWrong"=w2960, "input_arrTrig"=w2959) -> ("output_state"=w2962:T2, "output_dataCurrent"=w2964:u16[], "output_LC_Event_l1"=w2958:bool, "output_LC_Laser_l2"=w2955:bool, "output_LC_Event_l2"=w2956:bool, "output_LC_Laser_l1"=w2957:bool)  [unwired: 5 in]
            }
            frame "SelectReward_pre" {
              # "iState"
              # "Tcycle\nReward"
              # "nRewTrials"
              # "Tcycle\nGeneric"
              # "counter"
              n1402 = call "myRIO_BRig_RT_dataCurrent_nRewTrials.vi"() -> ("output_nRewTrials"=w3002:i32)  [unwired: 11 in]
              n1403 = Equal?(x=w3011, y=enum16{"Left", "Right"}."Left") -> (x = y?=w3012:bool)
              n1404 = Index Array(array=w3003, index=w3002) -> (element=w3001:u16)
              n1405 = call "myRIO_BRig_RT_dataExp_Tcycle_Reward__L.vi"() -> ("output_Tcycle_Reward__L"=w3015:i32)  [unwired: 11 in]
              n1406 = call "myRIO_BRig_RT_dataExp_Tcycle_Reward__R.vi"() -> ("output_Tcycle_Reward__R"=w3016:i32)  [unwired: 11 in]
              n1407 = Increment(x=w3001) -> (x+1=w3000:u16)
              n1408 = Select(t=w3015, s=w3012, f=w3016) -> (s? t:f=w3014:i32)
              n1409 = call "myRIO_BRig_RT__Case_Exp_subState_LC__Reward.vi"("input_spout"=w3011, "input_dataCurrent"=w3003, "input_dataLC"=w3010) -> ()  [unwired: 6 in, 2 out]
              n1410 = call "myRIO_BRig_RT_dataCurrent_count_generic.vi"() -> ("output_count_generic"=w3005:i32)  [unwired: 11 in]
              n1411 = call "myRIO_BRig_RT_dataCurrent_Tcycle_generic.vi"() -> ("output_Tcycle_generic"=w3006:i32)  [unwired: 11 in]
              n1412 = Index Array(array=w3017, index=w3014) -> (element=w3007:u16)
              n1413 = call "myRIO_BRig_RT_dataCurrent_iState.vi"() -> ("output_iState"=w2995:i32)  [unwired: 11 in]
              n1414 = Replace Array Subset(array=w3003, new element #1=w3000, index #1=w3002, new element #2=u16 0 ("new element/subarray"), index #2=w3005, new element #3=w3007, index #3=w3006, new element #4=u16 1 ("new element/subarray"), index #4=w2995) -> (w3018:u16[])
            }
            frame "SelectReward" {
              n1415 = call "myRIO_BRig_RT__Case_Exp_State_Reward.vi"("input_dataCurrent"=w3039, "input_state"=w3036, "input_spout"=w3034) -> ("output_dataCurrent"=w3038:u16[], "output_state"=w3037:T2, "output__L"=w3032:bool, "output__R"=w3033:bool)  [unwired: 9 in]
            }
            frame "SelectRewardPost_pre" {
              # "nRewards"
              # "nRewTrials"
              # "Tcycle"
              # "counter"
              n1416 = call "myRIO_BRig_RT_dataBlock_nRewards__L.vi"() -> ("output_nRewards__L"=w3055:i32)  [unwired: 11 in]
              n1417 = call "myRIO_BRig_RT_dataBlock_nRewards__R.vi"() -> ("output_nRewards__R"=w3054:i32)  [unwired: 11 in]
              n1418 = call "myRIO_BRig_RT_dataCurrent_Tcycle_generic.vi"() -> ("output_Tcycle_generic"=w3074:i32)  [unwired: 11 in]
              n1419 = call "myRIO_BRig_RT_dataCurrent_count_generic.vi"() -> ("output_count_generic"=w3076:i32)  [unwired: 11 in]
              n1420 = case shown="\"Left\", Default" w3048 {
                tunnel: w3060 -> [w3081 w3085]
                tunnel: [w3080 w3085] -> w3059
                tunnel: [w3082 w3083] -> w3058
                tunnel: w3057 -> [w3082 w3084]
                frame "Left", Default {
                  n1421 = Increment(x=w3081) -> (x+1=w3080:u16)
                }
                frame "Right" {
                  n1422 = Increment(x=w3084) -> (x+1=w3083:u16)
                }
              }
              "nRewards_Left" <- w3059
              "nRewards_Right" <- w3058
              n1423 = Equal?(x=w3048, y=enum16{"Left", "Right"}."Left") -> (x = y?=w3047:bool)
              n1424 = Select(t=w3055, s=w3047, f=w3054) -> (s? t:f=w3053:i32)
              n1425 = call "myRIO_BRig_RT_dataExp_Tcycle_RewardPost.vi"() -> ("output_Tcycle_RewardPost"=w3070:i32)  [unwired: 11 in]
              n1426 = call "myRIO_BRig_RT_dataCurrent_nRewTrials.vi"() -> ("output_nRewTrials"=w3056:i32)  [unwired: 11 in]
              n1427 = Index Array(array=w3071, index=w3070) -> (element=w3073:u16)
              n1428 = Index Array(array=w3050, index=w3056) -> (element=w3045:u16)
              n1429 = Replace Array Subset(array=w3050, new element #1=u16 0 ("new element/subarray"), index #1=w3076, new element #2=w3073, index #2=w3074) -> (w3072:u16[])
              n1430 = Replace Array Subset(array=w3052, new element=w3045, index (row)=w3046, index (col)=w3053) -> (w3051:u16[][])
              n1431 = local write "nRewards_cur"(w3045) -> ()
            }
            frame "SelectRewardPost" {
              n1432 = call "myRIO_BRig_RT__Case_Exp_State_RewardPost.vi"("input_state"=w3100, "input_dataCurrent"=w3103) -> ("output_state"=w3101:T2, "output_dataCurrent"=w3102:u16[])  [unwired: 8 in]
            }
            frame "SelectWrong_pre" {
              # "iState"
              # "Tcycle"
              # "counter"
              n1433 = call "myRIO_BRig_RT_dataCurrent_Tcycle_generic.vi"() -> ("output_Tcycle_generic"=w3128:i32)  [unwired: 11 in]
              n1434 = call "myRIO_BRig_RT_dataCurrent_count_generic.vi"() -> ("output_count_generic"=w3130:i32)  [unwired: 11 in]
              n1435 = call "myRIO_BRig_RT_dataExp_Tcycle_Wrong.vi"() -> ("output_Tcycle_Wrong"=w3126:i32)  [unwired: 11 in]
              n1436 = call "myRIO_BRig_RT__Case_Exp_subState_LC__Wrong.vi"("input_spout"=w3122, "input_dataCurrent"=w3123, "input_dataLC"=w3120) -> ()  [unwired: 6 in, 2 out]
              n1437 = Index Array(array=w3124, index=w3126) -> (element=w3127:u16)
              n1438 = call "myRIO_BRig_RT_dataCurrent_iState.vi"() -> ("output_iState"=w3114:i32)  [unwired: 11 in]
              n1439 = Replace Array Subset(array=w3123, new element #1=u16 0 ("new element/subarray"), index #1=w3130, new element #2=w3127, index #2=w3128, new element #3=u16 2 ("new element/subarray"), index #3=w3114) -> (w3125:u16[])
            }
            frame "SelectWrong" {
              n1440 = call "myRIO_BRig_RT__Case_Exp_State_Wrong.vi"("input_state"=w3144, "input_dataCurrent"=w3153) -> ("output_state"=w3141:T2, "output_dataCurrent"=w3152:u16[])  [unwired: 8 in]
              n1441 = Not Equal?(x=w3144, y=w3141) -> (x != y?=w3143:bool)
              n1442 = Select(t=myRIO_BRig_RT__Case_Exp_stateList."SelectWrong_post" ("Enum"), s=w3143, f=w3141) -> (s? t:f=w3140:T2)
            }
            frame "SelectWrong_post" {
            }
            frame "SelectTimeout_pre" {
              # "iState"
              # "Tcycle"
              # "counter"
              n1443 = xnode "Read/Write Control"("FPGA VI Reference In"=w3180, "error in"=w3179, "SelectionState"=FALSE) -> ("error out"=→"error out 3":errorcluster)  [unwired: 1 out]
              n1444 = call "myRIO_BRig_RT_dataCurrent_Tcycle_generic.vi"() -> ("output_Tcycle_generic"=w3202:i32)  [unwired: 11 in]
              n1445 = call "myRIO_BRig_RT_dataCurrent_count_generic.vi"() -> ("output_count_generic"=w3200:i32)  [unwired: 11 in]
              n1446 = call "myRIO_BRig_RT_dataExp_Tcycle_Timeout.vi"() -> ("output_Tcycle_Timeout"=w3204:i32)  [unwired: 11 in]
              n1447 = call "myRIO_BRig_RT__Case_Exp_subState_LC__Timeout.vi"("input_spout"=w3195, "input_dataCurrent"=w3196, "input_dataLC"=w3194) -> ()  [unwired: 6 in, 2 out]
              n1448 = Index Array(array=w3198, index=w3204) -> (element=w3203:u16)
              n1449 = call "myRIO_BRig_RT_dataCurrent_iState.vi"() -> ("output_iState"=w3188:i32)  [unwired: 11 in]
              n1450 = Replace Array Subset(array=w3196, new element #1=u16 0 ("new element/subarray"), index #1=w3200, new element #2=w3203, index #2=w3202, new element #3=u16 3 ("new element/subarray"), index #3=w3188) -> (w3199:u16[])
            }
            frame "SelectTimeout" {
              n1451 = call "myRIO_BRig_RT__Case_Exp_State_Timeout.vi"("input_dataLC"=w3223, "input_state"=w3214, "input_dataCurrent"=w3228) -> ("output_state"=w3215:T2, "output_dataCurrent"=w3227:u16[])  [unwired: 6 in, 1 out]
              n1452 = Not Equal?(x=w3214, y=w3215) -> (x != y?=w3218:bool)
              n1453 = Select(t=myRIO_BRig_RT__Case_Exp_stateList."SelectTimeout_post" ("Enum"), s=w3218, f=w3215) -> (s? t:f=w3216:T2)
            }
            frame "SelectTimeout_post" {
            }
            frame "endTrial1" {
              # "Update dataBlock"
              n1454 = call "myRIO_BRig_RT__Case_Exp_State_endTrial1.vi"("input_spout"=w3261, "input_dataBlock"=w3260, "input_dataCurrent"=w3258) -> ("output_dataBlock"=w3259:u16[][], "output_dataCurrent"=w3257:u16[])  [unwired: 7 in]
            }
            frame "endTrial2" {
              # "update dataTrial"
              n1455 = call "myRIO_BRig_RT__Case_Exp_State_endTrial2.vi"("input_spout"=w3280, "input_dataTrial"=w3284, "input_dataCurrent"=w3282) -> ("output_dataTrial"=w3283:u16[][], "output_dataCurrent"=w3281:u16[])  [unwired: 7 in]
            }
            frame "endTrial3" {
              # "nRewTrials"
              # "iTrial"
              # "I_blockUntilReward"
              # "TPB"
              # "end block?"
              n1456 = local read "STOP_endTrial"() -> (w3310:bool)
              n1457 = local read "STOP_abort"() -> (w3309:bool)
              n1458 = xnode "Read/Write Control"("FPGA VI Reference In"=w3300, "error in"=w3299, "SelectionState"=FALSE) -> ("error out"=→"error out 2":errorcluster)  [unwired: 1 out]
              n1459 = local read "START"() -> (w3307:bool)
              n1460 = call "myRIO_BRig_RT_dataExp_IblockUntilReward.vi"() -> ("output_I_blockUntilReward"=w3317:i32)  [unwired: 11 in]
              n1461 = Index Array(array=w3303, index=w3317) -> (element=w3301:u16)
              n1462 = Not(x=w3307) -> (.not. x?=w3308:bool)
              n1463 = Not Equal To 0?(x=w3301) -> (x != 0?=w3315:bool)
              n1464 = Compound Arithmetic op=OR(w3310, w3308, w3309) -> (w3295:bool)
              n1465 = call "myRIO_BRig_RT_dataCurrent_nRewTrials.vi"() -> ("output_nRewTrials"=w3313:i32)  [unwired: 11 in]
              n1466 = call "myRIO_BRig_RT_dataCurrent_iTrial.vi"() -> ("output_iTrial"=w3314:i32)  [unwired: 11 in]
              n1467 = Select(t=w3313, s=w3315, f=w3314) -> (s? t:f=w3312:i32)
              n1468 = call "myRIO_BRig_RT_dataCurrent_TpB.vi"() -> ("output_TpB"=w3316:i32)  [unwired: 11 in]
              n1469 = Index Array(array=w3304, index #1=w3316, index #2=w3312) -> (element #1=w3305:u16, element #2=w3306:u16)
              n1470 = Less Or Equal?(x=w3305, y=w3306) -> (x <= y?=w3296:bool)
              n1471 = Or(x=w3295, y=w3296) -> (x .or. y?=w3293:bool)
              n1472 = Select(t=myRIO_BRig_RT__Case_Exp_stateList."saveData_dataBlock" ("Enum"), s=w3293, f=myRIO_BRig_RT__Case_Exp_stateList."dummyState" ("Enum")) -> (s? t:f=w3302:T2)
            }
            frame "endBlock" {
              # "R"
              # "L"
              # "idxDataBlock"
              n1473 = Equal?(x=w3341, y=enum16{"Left", "Right"}."Left") -> (x = y?=w3340:bool)
              n1474 = call "myRIO_BRig_RT_dataCurrent_idxDataBlockL.vi"() -> ("output_idxDataBlock__L"=w3344:i32)  [unwired: 11 in]
              n1475 = call "myRIO_BRig_RT_dataCurrent_idxDataBlockR.vi"() -> ("output_idxDataBlock__R"=w3343:i32)  [unwired: 11 in]
              n1476 = Increment(x=w3335) -> (x+1=w3334:i32)
              n1477 = local read "START"() -> (w3364:bool)
              n1478 = local read "STOP_endBlock"() -> (w3359:bool)
              n1479 = local read "STOP_endTrial"() -> (w3362:bool)
              n1480 = local read "STOP_abort"() -> (w3361:bool)
              n1481 = Select(t=w3344, s=w3340, f=w3343) -> (s? t:f=w3338:i32)
              n1482 = To Unsigned Word Integer(number=w3334) -> (unsigned 16bit integer=w3336:u16)
              n1483 = Not(x=w3364) -> (.not. x?=w3363:bool)
              n1484 = Replace Array Subset(array=w3339, new element=w3336, index=w3338) -> (w3337:u16[])
              n1485 = Compound Arithmetic op=OR(w3363, w3359, w3362, w3361) -> (w3360:bool)
              n1486 = Select(t=myRIO_BRig_RT__Case_Exp_stateList."endExp" ("Enum"), s=w3360, f=myRIO_BRig_RT__Case_Exp_stateList."dummyState_endBlock" ("Enum")) -> (s? t:f=w3368:T2)
            }
            frame "endExp" {
            }
            frame "commConnect" {
              n1487 = call "myRIO_BRig_RT_comm_webdav_connect.vi"("input_password"="Host Password", "input_username"="Host UserName") -> ("output_Iconnected"=w3389:bool, "output_hSession"=w3407:T6)  [unwired: 7 in, 1 out]
              "Connected To Host?" <- w3389
              n1488 = case shown="False" w3389 {
                frame False {
                  n1489 = One Button Dialog(message="Connection Failed!\nData not being saved!") -> ()  [unwired: 1 in, 1 out]
                }
                frame True {
                }
              }
            }
            frame "commUpload_pre" {
              n1490 = Select(t=myRIO_BRig_RT__Case_Exp_stateList."commUpload_dataBlock" ("Enum"), s=w3414, f=myRIO_BRig_RT__Case_Exp_stateList."endBlock") -> (s? t:f=w3412:T2)
            }
            frame "commUpload_dataBlock" {
              n1491 = call "myRIO_BRig_RT_comm_webdav_uploadFile__data.vi"("input_fileName_prefix"=w3435, "input_fileName"="dataBlock" ("input_filename"), "input_hSession"=w3437) -> ()  [unwired: 8 in, 1 out]
            }
            frame "commUpload_dataCurrent" {
              n1492 = call "myRIO_BRig_RT_comm_webdav_uploadFile__data.vi"("input_fileName_prefix"=w3456, "input_fileName"="dataCurrent" ("input_filename"), "input_hSession"=w3458) -> ()  [unwired: 8 in, 1 out]
            }
            frame "commUpload_dataExp" {
              n1493 = call "myRIO_BRig_RT_comm_webdav_uploadFile__data.vi"("input_fileName_prefix"=w3477, "input_fileName"="dataExp" ("input_filename"), "input_hSession"=w3479) -> ()  [unwired: 8 in, 1 out]
            }
            frame "commUpload_dataLC" {
              n1494 = call "myRIO_BRig_RT_comm_webdav_uploadFile__data.vi"("input_fileName_prefix"=w3498, "input_fileName"="dataLC" ("input_filename"), "input_hSession"=w3500) -> ()  [unwired: 8 in, 1 out]
            }
            frame "commUpload_dataTrial" {
              n1495 = call "myRIO_BRig_RT_comm_webdav_uploadFile__data.vi"("input_fileName_prefix"=w3522, "input_fileName"="dataTrial" ("input_filename"), "input_hSession"=w3524) -> ()  [unwired: 8 in, 1 out]
            }
            frame "saveData_dataBlock" {
              # "idxDataBlockR"
              # "idxDataBlockL"
              n1496 = call "myRIO_BRig_RT_dataCurrent_idxDataBlockL.vi"() -> ("output_idxDataBlock__L"=w3548:i32)  [unwired: 11 in]
              n1497 = call "myRIO_BRig_RT_dataCurrent_idxDataBlockR.vi"() -> ("output_idxDataBlock__R"=w3549:i32)  [unwired: 11 in]
              n1498 = Index Array(array=w3550, index #1=w3548, index #2=w3549) -> (element #1=w3547:u16, element #2=w3546:u16)
              n1499 = Greater?(x=w3547, y=w3546) -> (0:w3545:bool)
              n1500 = Select(t=w3547, s=w3545, f=w3546) -> (s? t:f=w3543:u16)
              n1501 = Increment(x=w3543) -> (x+1=w3542:u16)
              n1502 = To Long Integer(number=w3542) -> (32bit integer=w3541:i32)
              n1503 = Array Subset(array=w3544, length (row)=w3541) -> (w3540:u16[][])  [unwired: 3 in]
              n1504 = call "myRIO_BRig_RT_comm_webdav_saveArrayToFile__2D_u16.vi"("Array"=w3540, "input_filename"="dataBlock") -> ()  [unwired: 10 in]
            }
            frame "saveData_dataCurrent" {
              n1505 = call "myRIO_BRig_RT_comm_webdav_saveArrayToFile__1D_u16.vi"("Array"=w3569, "input_filename"="dataCurrent") -> ()  [unwired: 10 in]
            }
            frame "saveData_dataExp" {
              # "runTime"
              n1506 = Get Date/Time In Seconds() -> (seconds since 1Jan1904=w3597:timestamp)
              n1507 = To Double Precision Float(number=w3597) -> (double precision float=w3596:dbl)
              n1508 = call "myRIO_BRig_RT_dataExp_runTime_seconds.vi"() -> ("output_RunTime_minutes"=w3595:i32)  [unwired: 11 in]
              n1509 = Subtract(x=w3596, y=w3594) -> (x-y=w3591:dbl)
              n1510 = To Unsigned Word Integer(number=w3591) -> (unsigned 16bit integer=w3590:u16)
              n1511 = Replace Array Subset(array=w3589, new element=w3590, index=w3595) -> (w3592:u16[])
              n1512 = call "myRIO_BRig_RT_comm_webdav_saveArrayToFile__1D_u16.vi"("Array"=w3592, "input_filename"="dataExp") -> ()  [unwired: 10 in]
            }
            frame "saveData_dataLC" {
              n1513 = call "myRIO_BRig_RT_comm_webdav_saveArrayToFile__1D_u16.vi"("Array"=w3616, "input_filename"="dataLC") -> ()  [unwired: 10 in]
            }
            frame "saveData_dataTrial" {
              # "idxTrial"
              n1514 = call "myRIO_BRig_RT_dataCurrent_idxDataTrial.vi"() -> ("output_idxDataTrial"=w3640:i32)  [unwired: 11 in]
              n1515 = Index Array(array=w3641, index=w3640) -> (element=w3633:u16)
              n1516 = Increment(x=w3633) -> ()  [unwired: 1 out]
              n1517 = To Long Integer(number=w3633) -> (32bit integer=w3637:i32)
              n1518 = Array Subset(array=w3638, length (row)=w3637) -> (w3639:u16[][])  [unwired: 3 in]
              n1519 = call "myRIO_BRig_RT_comm_webdav_saveArrayToFile__2D_u16.vi"("Array"=w3639, "input_filename"="dataTrial") -> ()  [unwired: 10 in]
            }
            frame "dummyState" {
              n1520 = call "myRIO_BRig_RT_dataCurrent_iTrial.vi"() -> ("output_iTrial"=w3663:i32)  [unwired: 11 in]
              n1521 = Index Array(array=w3664, index=w3663) -> (element=w3662:u16)
              n1522 = Equal?(x=w3662, y=u16 1) -> (x = y?=w3660:bool)
              n1523 = Equal To 0?(x=w3671) -> (x = 0?=w3672:bool)
              n1524 = Select(t=u16 13, s=w3660, f=u16 15) -> (s? t:f=w3657:u16)
              n1525 = Select(t=w3657, s=w3672, f=w3671) -> (s? t:f=w3670:u16)
              n1526 = Decrement(x=w3670) -> (x-1=w3669:u16)
              n1527 = Equal To 0?(x=w3669) -> (x = 0?=w3668:bool)
              n1528 = Select(t=myRIO_BRig_RT__Case_Exp_stateList."initTrial" ("Enum"), s=w3668, f=w3666) -> (s? t:f=w3665:T2)
            }
            frame "dummyState_endBlock" {
              n1529 = call "myRIO_BRig_RT_dataCurrent_iTrial.vi"() -> ("output_iTrial"=w3696:i32)  [unwired: 11 in]
              n1530 = Index Array(array=w3697, index=w3696) -> (element=w3695:u16)
              n1531 = Equal?(x=w3695, y=u16 1) -> (x = y?=w3693:bool)
              n1532 = Equal To 0?(x=w3704) -> (x = 0?=w3705:bool)
              n1533 = Select(t=u16 1, s=w3693, f=u16 3) -> (s? t:f=w3690:u16)
              n1534 = Select(t=w3690, s=w3705, f=w3704) -> (s? t:f=w3703:u16)
              n1535 = Decrement(x=w3703) -> (x-1=w3702:u16)
              n1536 = Equal To 0?(x=w3702) -> (x = 0?=w3701:bool)
              n1537 = Select(t=myRIO_BRig_RT__Case_Exp_stateList."initBlock" ("Enum"), s=w3701, f=w3699) -> (s? t:f=w3698:T2)
            }
          }
          n1538 = local read "MTrig_Laser_Switch"() -> (w1355:bool)
          n1539 = Not(x=w1355) -> (.not. x?=w1356:bool)
          n1540 = Select(t=w1397, s=w1400, f=w1398) -> (s? t:f=w1399:bool)
          n1541 = And(x=w1357, y=w1356) -> (x .and. y?=w1351:bool)
          n1542 = And(x=w1357, y=w1355) -> (x .and. y?=w1353:bool)
          n1543 = Or(x=w1354, y=w1353) -> (x .or. y?=w1344:bool)
          n1544 = Or(x=w1353, y=w1352) -> (x .or. y?=w1343:bool)
          n1545 = Or(x=w1350, y=w1351) -> (x .or. y?=w1346:bool)
          n1546 = Or(x=w1351, y=w1349) -> (x .or. y?=w1345:bool)
          n1547 = Or(x=w1359, y=w1360) -> (x .or. y?=w1348:bool)
          n1548 = Or(x=w1426, y=w1425) -> (x .or. y?=w1347:bool)
          n1549 = case shown="True" w1454 {
            tunnel: w1451 -> [w1475 w1483]
            tunnel: w1453 -> [_ w1479]
            tunnel: w1452 -> [_ w1478]
            tunnel: w1371 -> [_ w1477]
            tunnel: w1423 -> [_ w1476]
            tunnel: [w1475 w1482] -> w1450
            tunnel: w1449 -> [w1474 w1481]
            tunnel: [w1474 w1480] -> w1448
            frame False {
            }
            frame True {
              n1550 = call "myRIO_BRig_RT__Case_Exp__recordLick.vi"("intput_state__trialEnd"=w1476, "intput_state__trialStart"=w1477, "input_lick__R"=w1478, "input_lick__L"=w1479, "input_dataCurrent"=w1481, "input_dataLick"=w1483) -> ("output_dataCurrent"=w1480:u16[], "output_dataLick"=w1482:u16[][])  [unwired: 4 in]
            }
          }
          n1551 = Or(x=w1427, y=w1412) -> (x .or. y?=w1401:bool)
          n1552 = Or(x=w1411, y=w1428) -> (x .or. y?=w1424:bool)
          n1553 = Or(x=w1455, y="STOP_abort") -> (x .or. y?=w1457:bool)
          n1554 = Select(t=w1386, s=w1387, f=w1385) -> (s? t:f=w1370:u16)
          n1555 = Select(t=w1388, s=w1390, f=w1389) -> (s? t:f=w1369:u16)
          n1556 = Select(t=u16 0, s=w1393, f=w1392) -> (s? t:f=w1377:u16)
          n1557 = xnode "Read/Write Control"("FPGA VI Reference In"=w1403, "error in"=w1402, "A6_Act"=w1399, "audioTrigger_L"=w1401, "audioAmp_L"=w1437, "audioFreq_L_kHz"=w1410, "audioTrigger_R"=w1424, "audioAmp_R"=w1438, "audioFreq_R_kHz"=w1439, "CueLed_Event"=w1358, "A3_SL"=w1348, "A1_SR"=w1347, "LC_Event_l1"=w1346, "LC_Laser_l1"=w1345, "LC_Event_l2"=w1344, "LC_Laser_l2"=w1343) -> ("FPGA VI Reference Out"=w1447:refnum<k20>, "error out"=w1446:errorcluster, "AnaIn_0"=w1363:i16, "AnaIn_1"=w1376:i16)
          n1558 = call "myRIO_BRig_RT_dataAnalog_enterData__PortC.vi"("input_iState"=w1371, "input_AI0"=w1363, "input_iEvent"=w1377, "input_AI1"=w1376, "input_iTrial"=w1370, "input_iBlock"=w1369, "input_index"=w1378, "input_dataAnalog"=w1396) -> ("output_dataAnalog"=w1395:u16[][])  [unwired: 3 in]
          n1559 = call "myRIO_BRig_RT_TCP__v3__PortC.vi"("input_hTCP"=w1383, "input_AI1"=w1376, "input_AI0"=w1363, "input_I_connected_TCP"=w1379, "input_iBlock"=w1369, "input_spout"=w1368, "input_iTrial"=w1370, "input_error"=w1381, "input_countTrial"=w1365, "input_iState"=w1371) -> ("output_hTCP"=w1382:refnum<k5>, "output_countTrial"=w1364:u16, "output_error"=w1380:errorcluster)  [unwired: 3 in]
          n1560 = node-c288() -> ()  [unwired: 1 in, 1 out]
          n1561 = Increment(x=w1377) -> (x+1=w1384:u16)
          n1562 = Increment(x=w1378) -> (x+1=w1394:i32)
          "cState" <- w1371
        }
        n1563 = node-c288(w1293) -> ()  [unwired: 1 out]
        n1564 = flat-sequence {
          tunnel: w1289 -> [w1338]
          tunnel: w1288 -> [w1337]
          tunnel: [w1336] -> w1281
          tunnel: [w1335] -> w1280
          tunnel: [w1341] -> w1282
          tunnel: [w1342] -> w1287
          tunnel: w1281 -> [w1342]
          tunnel: w1280 -> [w1341]
          frame #0 {
            w1332 = u8 0
            w1333 = u16 0 ("AudioLeft_phase_inc")
            w1334 = FALSE
            n1565 = xnode "Read/Write Control"("FPGA VI Reference In"=w1338, "error in"=w1337, "Counts_Reset"=TRUE, "audioTrigger_L"=w1334, "audioFreq_L_kHz"=w1332, "audioAmp_L"=w1333, "audioTrigger_R"=w1334, "audioFreq_R_kHz"=w1332, "audioAmp_R"=w1333, "A3_SL"=w1334, "A1_SR"=w1334, "A6_Act"=w1334) -> ("FPGA VI Reference Out"=w1336:refnum<k20>, "error out"=w1335:errorcluster)
          }
          frame #1 {
            w1340 = FALSE ("START")
            n1566 = local write "START"(w1340) -> ()
            n1567 = local write "STOP_endTrial"(w1340) -> ()
            n1568 = local write "STOP_endBlock"(w1340) -> ()
          }
        }
        n1569 = stacked-sequence {
          tunnel: w1265 -> [w1312 _]
          tunnel: w1263 -> [w1313 _]
          tunnel: w1262 -> [_ w1318]
          tunnel: w1261 -> [_ w1317]
          tunnel: w1260 -> [_ w1316]
          tunnel: w1259 -> [w1306 _]
          tunnel: w1239 -> [w1303 _]
          tunnel: w1238 -> [w1302 _]
          frame #0 {
            n1570 = call "myRIO_BRig_RT_dataCurrent_idxDataLick.vi"() -> ("output_idxDataLick"=w1307:i32)  [unwired: 11 in]
            n1571 = Index Array(array=w1306, index=w1307) -> (element=w1309:u16)
            n1572 = Array Subset(array=w1303, length (row)=w1302) -> (w1304:u16[][])  [unwired: 3 in]
            n1573 = Increment(x=w1309) -> (x+1=w1310:u16)
            n1574 = call "myRIO_BRig_RT_comm_webdav_saveArrayToFile__1D_u16.vi"("Array"=w1313, "input_filename"="dataMTrig") -> ()  [unwired: 10 in]
            n1575 = To Long Integer(number=w1310) -> (32bit integer=w1308:i32)
            n1576 = Array Subset(array=w1312, length (row)=w1308) -> (w1311:u16[][])  [unwired: 3 in]
            n1577 = call "myRIO_BRig_RT_comm_webdav_saveArrayToFile__2D_u16.vi"("Array"=w1311, "input_filename"="dataLick") -> ()  [unwired: 10 in]
            n1578 = call "myRIO_BRig_RT_comm_webdav_saveArrayToFile__2D_u16.vi"("Array"=w1304, "input_filename"="dataAnalog") -> ()  [unwired: 10 in]
          }
          frame #1 {
            n1579 = case shown="True" w1318 {
              tunnel: w1317 -> [_ w1320]
              tunnel: w1316 -> [_ w1319]
              frame False {
              }
              frame True {
                n1580 = stacked-sequence {
                  tunnel: w1320 -> [w1322 w1329 w1331]
                  tunnel: w1319 -> [w1323 w1328 _]
                  frame #0 {
                    n1581 = call "myRIO_BRig_RT_comm_webdav_uploadFile__announce.vi"("input_addText"=TRUE, "input_fileName_prefix"=w1323, "intput_fileName"="curExp_end", "intput_hSession"=w1322) -> ("output_Isuccess"=w1321:bool)  [unwired: 6 in, 1 out]
                    n1582 = case shown="True" w1321 {
                      frame False {
                        n1583 = One Button Dialog(message="!!! Warning !!! Your data is located at C:\\BehaviorRig\\commTransfer") -> ()  [unwired: 1 in, 1 out]
                      }
                      frame True {
                        n1584 = Wait (ms)(milliseconds to wait=u32 20) -> ()  [unwired: 1 out]
                      }
                    }
                  }
                  frame #1 {
                    n1585 = call "myRIO_BRig_RT__endExp_sendData.vi"("input_fileName_prefix"=w1328, "input_hSession"=w1329) -> ()  [unwired: 8 in, 2 out]
                  }
                  frame #2 {
                    n1586 = local write "Connected To Host?"(FALSE ("Connected To Host?")) -> ()
                    n1587 = call <vilib>:"Close Session.vi"("session handle"=w1331) -> ()  [unwired: 14 in, 1 out]
                  }
                }
              }
            }
          }
        }
      }
    }
    n1588 = local read "STOP_abort"() -> (w44:bool)
  }
  n1589 = case shown="True" w5 {
    tunnel: w4 -> [_ w3728]
    tunnel: w3 -> [_ w3727]
    frame False {
    }
    frame True {
      n1590 = call "myRIO__TCP_disconnect_forWrite.vi"("input_error"=w3727, "input_hTCP"=w3728) -> ()  [unwired: 9 in, 1 out]
    }
  }
  n1591 = xnode "Read/Write Control"("FPGA VI Reference In"=w16, "error in"=w15, "FPGA_Stop"=TRUE) -> ("FPGA VI Reference Out"=w21:refnum<k20>, "error out"=w22:errorcluster)
  n1592 = xnode "Close FPGA VI Reference"("FPGA VI Reference In"=w21, "error in"=w22) -> ("error out"=w20:errorcluster)
  n1593 = call <vilib>:"Reset myRIO.vi"("error in (no error)"=w20) -> ()  [unwired: 10 in, 1 out]
